vi "MainKinetics.vi"() -> ()   [LabVIEW 2017]
uses:
  <vilib>/Utility/miscctls.llb/LVRowAndColumnTypeDef.ctl
  <vilib>/Utility/sysdir.llb/System Directory Type.ctl
  <vilib>/Utility/config.llb/Read Key (String).vi
  <vilib>/Utility/config.llb/Write Key (String).vi
  <vilib>/Utility/cursorutil.llb/Set Cursor (Icon Pict).vi
  PCAN_Driver/ControlCAN.lvlib
  <vilib>/Utility/config.llb/NI_LVConfig.lvlib
panel:
  out "Motor Speed RPM Serial":dbl
  out "DAQmx Device Name":tag
  out "PN":string
  out "FileName":string
  out "Numeric":dbl
  out "BurnInSpeed":u16
  out "VenableSpeed":u16
  out "CurrentTest":T1(ring)
  out "TesterVersion":string
  out "ClosePanel":bool=TRUE
  out "UUT SN Report":string
  out "Automation":bool
  out "Test Failed":bool
  out "AuxiOFFResult":bool
  out "AuxiONResult":bool
  out "SensCalResult":bool
  out "VisualInspectionResult":bool
  out "BurnResult":bool
  out "BurnSpeed":bool
  out "BurnTemp":bool
  out "BurnDC":bool
  out "TempControlResult":bool
  out "MotorTempResult":bool
  out "VenableDirectionResult":bool
  out "VenableResult":bool
  out "ComTestResult":bool=TRUE
  out "UUT SoftwareVer":string
  out "Next SN":i32
  in  "SetSN":bool
  out "Current SN":i32
  out "AO[1]Meas":dbl
  out "FullSpeed2 Speed":dbl
  out "FullSpeed2 Current":dbl
  out "FullSpeed1 Current":dbl
  out "FullSpeed1 Speed":dbl
  out "MaxBurnInTempVal":dbl
  out "UUT":u8
  out "CAN Status":bool
  out "Array":u64[][](array[numeric]) format="%016x"
  out "Motor Phase Current RMS":dbl
  out "Ambient Temperature":dbl
  out "Speed error":bool
  out "Commutation err":bool
  out "Under voltage/Over voltage":bool
  out "Derated drive temp":bool
  out "Motor Over temperature":bool
  out "Motor Sensor temp Fauilre":bool
  out "Drive Over temperature":bool
  out "Drive Sensor temp Failure":bool
  out "Ambient Over temp":bool
  out "Ambient Sensor temp":bool
  out "DC Voltage":dbl
  out "DC Current":dbl
  out "Power transistor Heat sink Temp.":dbl
  out "Motor Stator Temp.":dbl
  out "Motor Speed RPM":dbl
  out "ECS State":u16
  out "UUT":string="EBAY"
  in  "Logger Path":path
  in  "Report":bool
  in  "Start":bool
  in  "ATR":string[][](table)=[["Test Communication", "-", "-", "-", "-", ""], ["Set S/N", "-", "-", "-", "-", ""], ["Set Board Number", "-", "-", "-", "-", ""], [" ", "", "", "", "", ""], ["Test Communication", "-", "-", "-", "-", ""], ["Get S/N", "-", "-", "-", "", ""], ["Get Board Number", "-", "-", "-", "", ""], ["Get FW", "-", "-", "-", "", ""], ["Enable Motor", "", "", "", "", ""], ["Small position command", "", "", "", "", ""], ["Measure delta", "", "", "", "", ""], ["Velocity command", "", "", "", "", ""]]
  in  "Settings":bool
  in  "Refresh Button":bool
  out "Status":bool
  in  "VISA Kinetics":refnum<visa-resource-name>="COM6"
  in  "Serial Com":bool
  in  "Help Button":bool
  out "Pannel User Message":string
  in  "Stop Button":bool
  # "Kinetics"
  # "REDLER TECHNOLOGIES LTD"
  # "ver 1.2p"
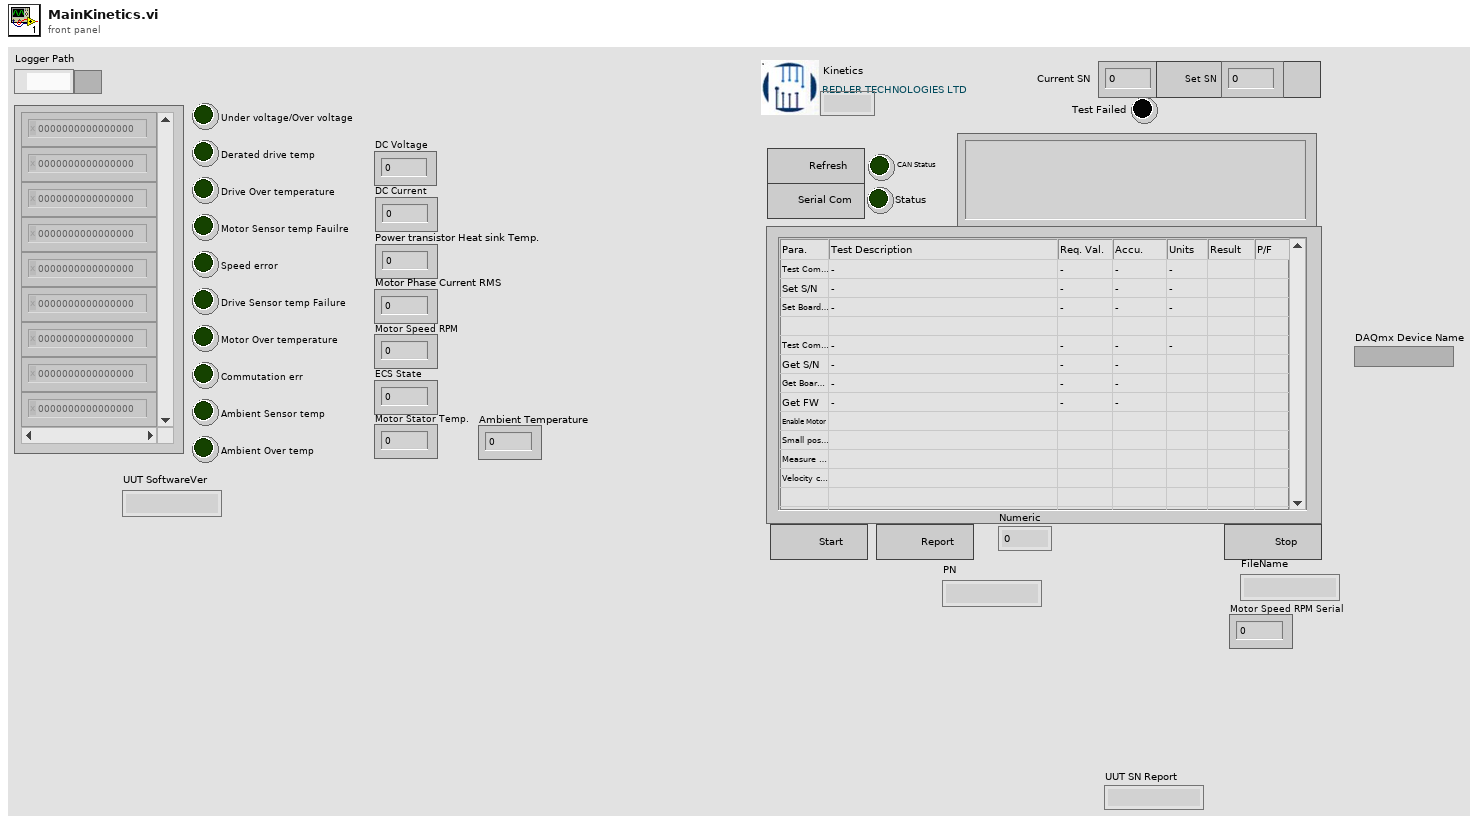
[diagram p1: front panel]
types:
  T1 = enum16{"Auxiliary", "Temp Sens Cal", "Com Test", "Enable Test", "Speed Command", "Stop Time", "Temp Control", "Burn in", "Visual Inspec", "Empty"}
  T2 = cluster{"VISA":refnum<visa-resource-name>, "Array Test":enum16{"Auxiliary", "Temp Sens Cal", "Com Test", "Enable Test", "Speed Command", "Stop Time", "Temp Control", "Burn in", "Visual Inspec", "Empty"}[]}
  T3 = cluster{"ID":u32, "MSGTYPE":u8, "LEN":u8, "aDATA":u8[]}[]
  T4 = enum16{"Erase ATR Table", "Stop", "MainProgram", "Initialize"}
  T5 = typedef "NI_LVConfig.lvlib/Config Data RefNum.ctl" = refnum<k1>
  T6 = enum16{"K15", "K16", "K17", "Venable", "Firmeware", "Fan", "Power", "120C", "110C", "100C", "90C", "80C", "70C", "60C", "50C", "40C", "30C", "25C", "20C", "10C", "0C"}
  T7 = enum16{"Stop", "Result", "FullSpeed2", "MD[1]=1", "FullSpeed1", "MD[1]=0"}
  T8 = enum8{"Term1", "Term2", "Current", "Fan", "TempCPU"}
  T9 = enum16{"Stop", "AO[1]=Meas.", "TA[5]", "AO[1]=0", "Start"}
  T10 = enum16{"Stop", "BurnIn", "Ambient Temp", "MotorSpeed", "DC Current Measure", "Start"}
  T11 = enum16{"Auxiliary", "Temp Sens Cal", "Com Test", "Enable Test", "Speed Command", "Stop Time", "Temp Control", "Burn in", "Visual Inspec", "Empty"}[]
  T12 = enum16{"K15", "K16", "K17", "Venable", "Firmeware", "Fan", "Power", "120C", "110C", "100C", "90C", "80C", "70C", "60C", "50C", "40C", "30C", "25C", "20C", "10C", "0C"}[]
  T13 = enum32{"6000", "11500", "15100", "11500-2", "6000-2"}[]
  T14 = enum8{"Enabled", "Disabled", "Disabled and Grayed Out"}
  T15 = typedef "LVRowAndColumnTypeDef.ctl" = cluster{"Row":i32, "Column":i32}
  T16 = enum32{"Invalid", "Standard", "Closed", "Hidden", "Minimized", "Maximized"}
  T17 = cluster{"ID":u32, "MSGTYPE":u8, "LEN":u8, "aDATA":u8[]}
  T18 = enum16{"open", "replace", "create", "open or create", "replace or create", "replace or create with confirmation"}
  T19 = typedef "ControlCAN.lvlib/DevType.ctl" = u32
  T20 = typedef "ControlCAN.lvlib/CAN Channel.ctl" = u32
  T21 = typedef "ControlCAN.lvlib/VCI_INIT_CONFIG.ctl" = cluster{"AccCode":u32, "AccMask":u32, "InitFlag":T22, "Fliter":T23, "Timing0":u8, "Timing1":u8, "Mode":T24}
  T22 = typedef "ControlCAN.lvlib/InitFlag.ctl" = u32
  T23 = typedef "ControlCAN.lvlib/Fliter.ctl" = u8
  T24 = typedef "ControlCAN.lvlib/Mode.ctl" = u8
  T25 = cluster{"DevType":T19, "DevIndex":u32, "CanIndex":T20, "VCI_INIT_CONFIG":T21}
  T26 = typedef "ControlCAN.lvlib/VCI_CAN_OBJ.ctl" = cluster{"ID":u32, "TimeStamp":u32, "TimeFlag":u8, "SendType":u8, "RemoteFlag":u8, "ExternFlag":u8, "DataLen":u8, "Data":u8[], "Reserved":u8[]}
  T27 = cluster{"Type":enum16{"接收", "发送"}, "Channel":T20, "Time":timestamp, "VCI_CAN_OBJ":T26}[]
  T28 = cluster{"Type":enum16{"接收", "发送"}, "Channel":T20, "Time":timestamp, "VCI_CAN_OBJ":T26}
  T29 = typedef "LVPoint32TypeDef.ctl" = cluster{"Horizontal":i32, "Vertical":i32}
  T30 = enum8{"Term1", "Term2", "Current", "Fan", "TempCPU"}[]
  T31 = typedef "System Directory Type.ctl" = i32
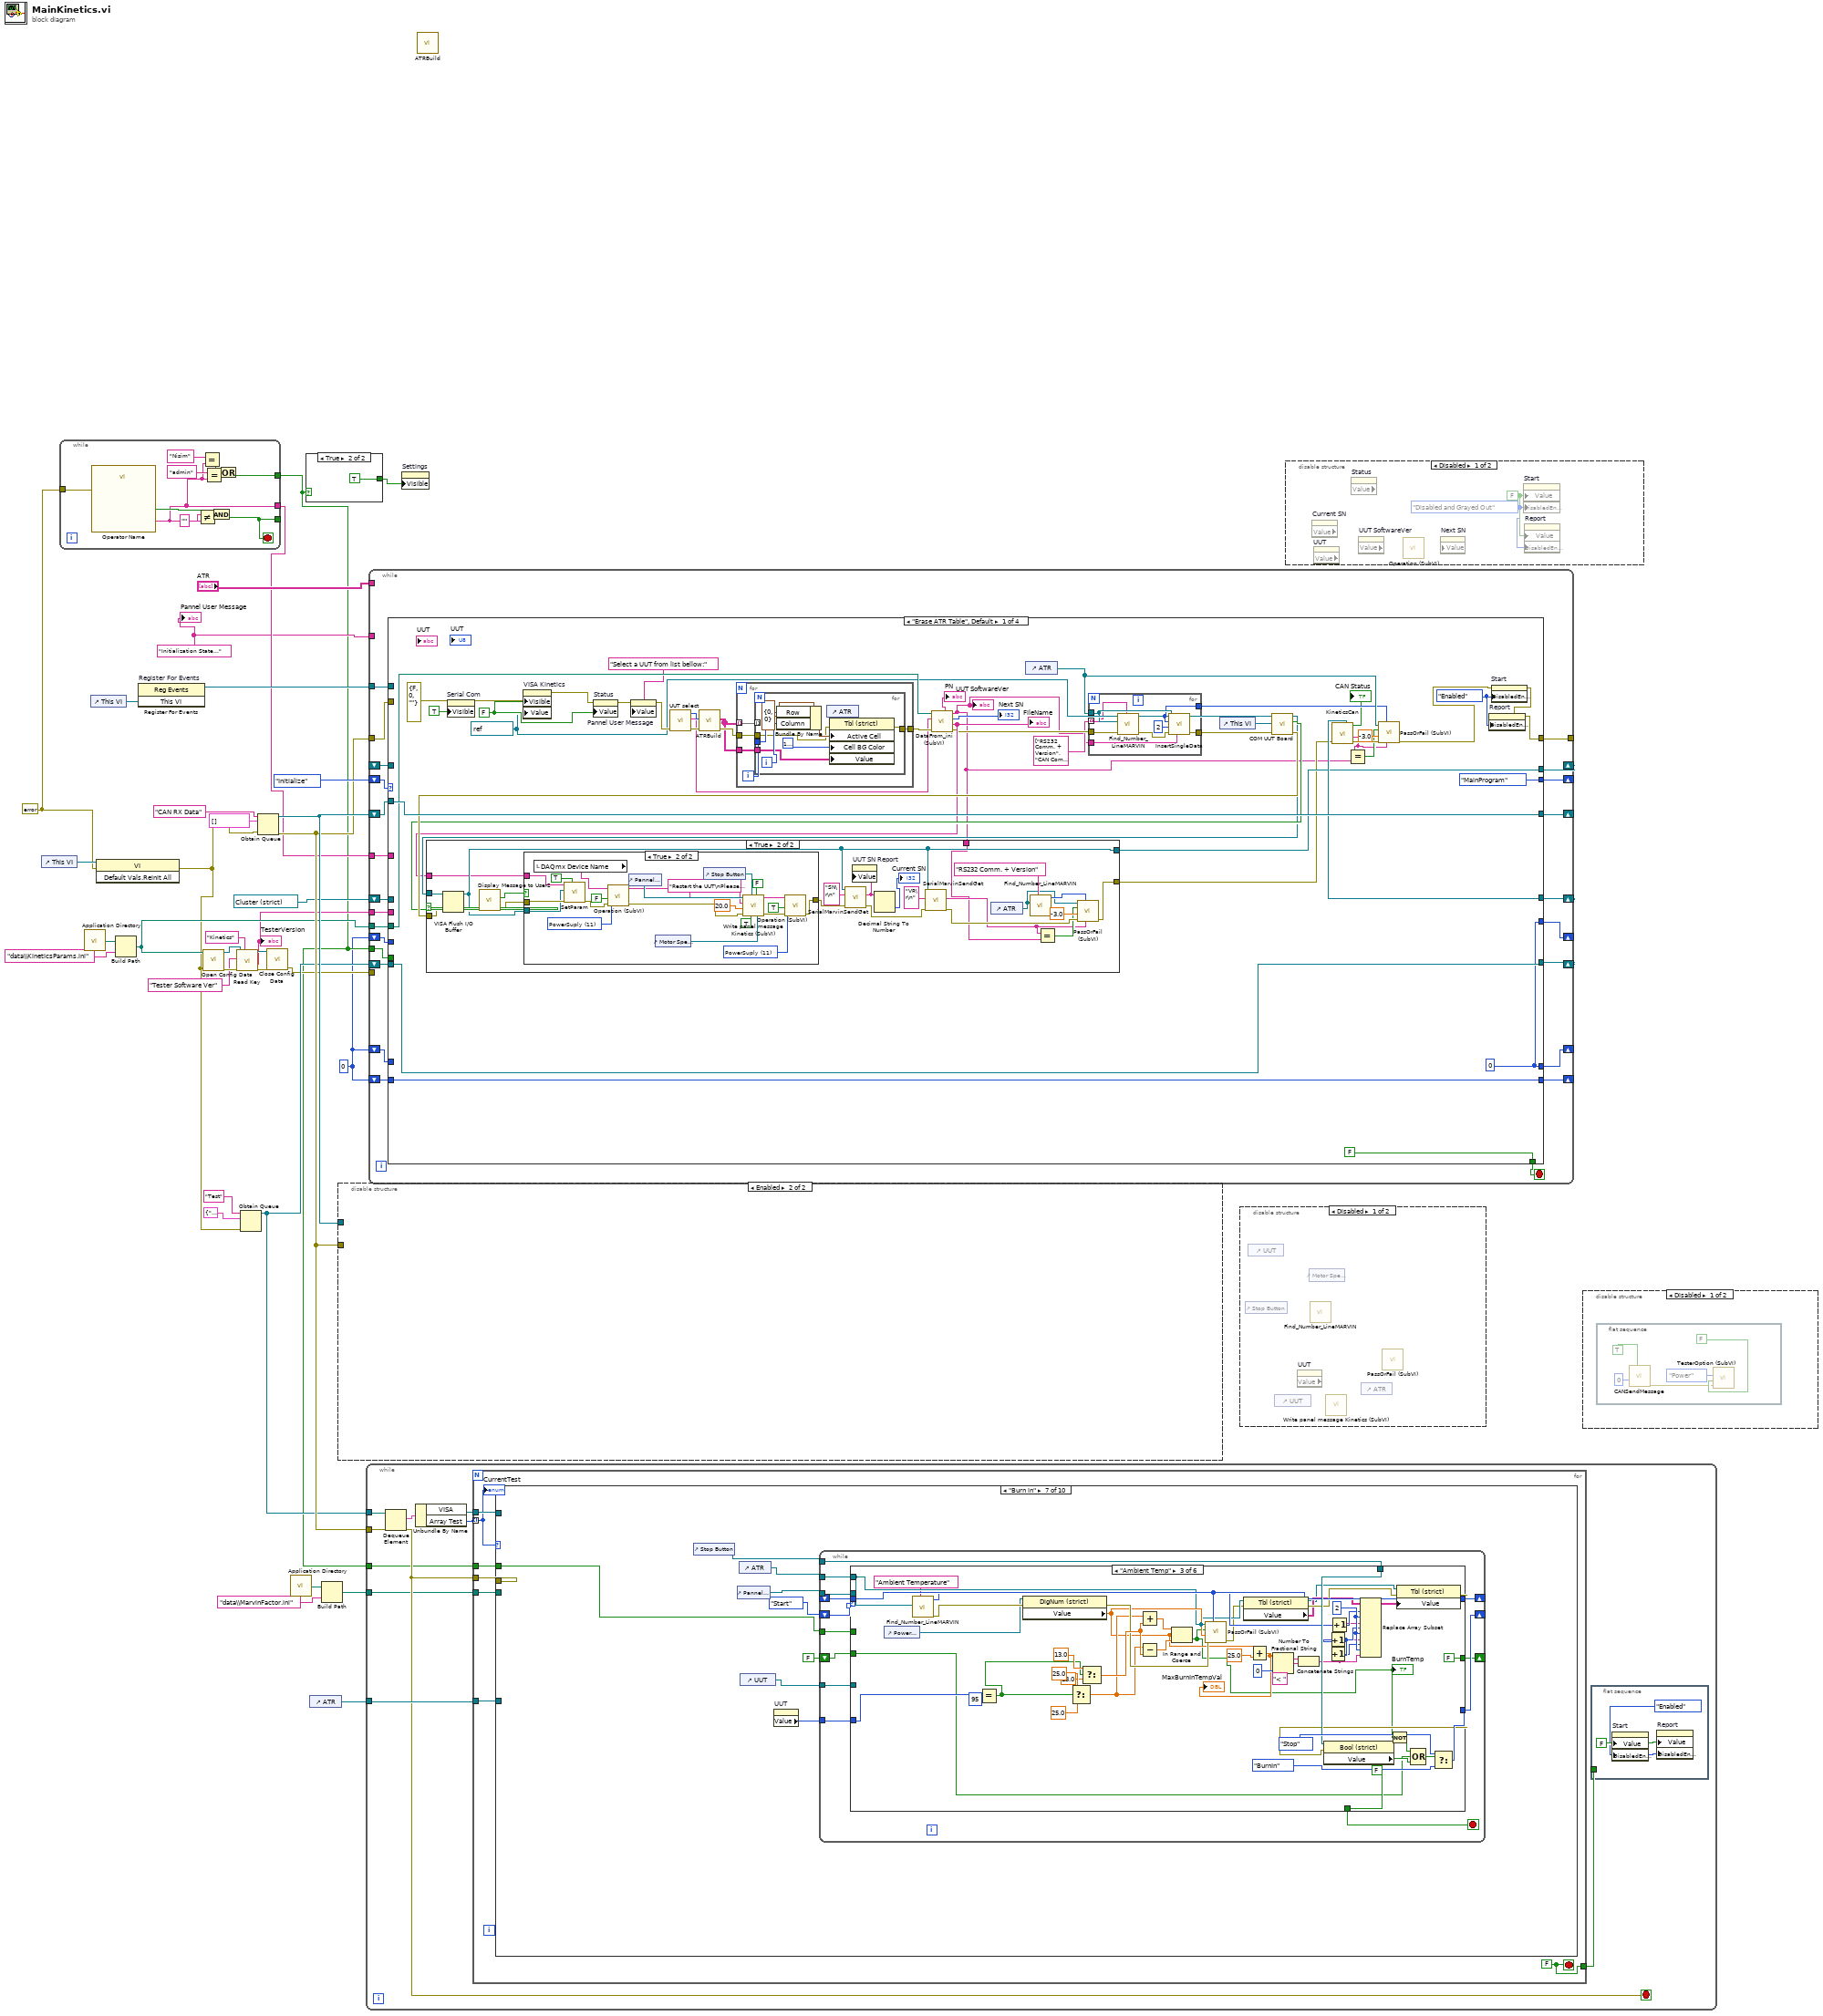
[diagram p0: block diagram]
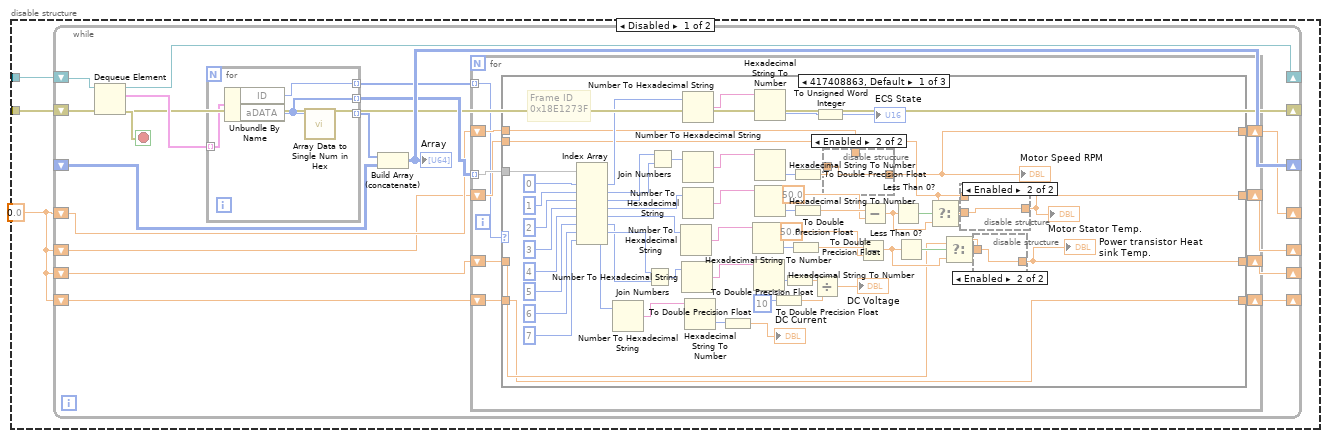
[diagram p2: hidden frame]
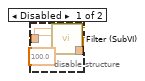
[diagram p3: hidden frame]
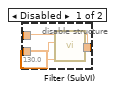
[diagram p4: hidden frame]
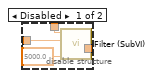
[diagram p5: hidden frame]
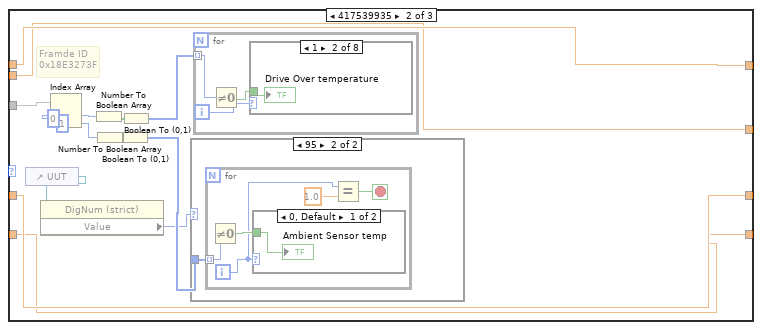
[diagram p6: hidden frame]
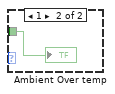
[diagram p8: hidden frame]
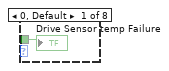
[diagram p9: hidden frame]
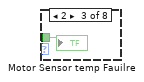
[diagram p10: hidden frame]
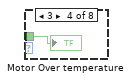
[diagram p11: hidden frame]
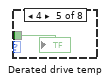
[diagram p12: hidden frame]
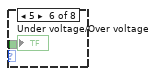
[diagram p13: hidden frame]
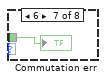
[diagram p14: hidden frame]
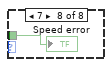
[diagram p15: hidden frame]
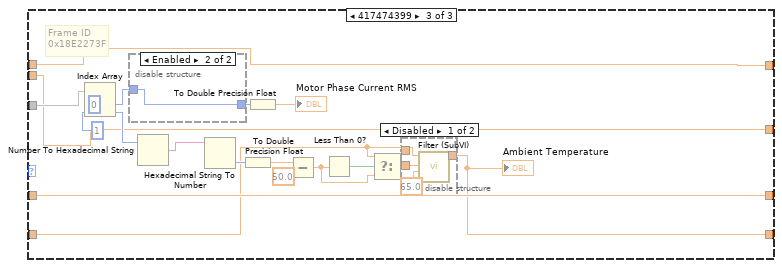
[diagram p16: hidden frame]
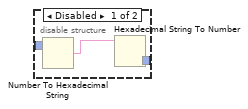
[diagram p18: hidden frame]
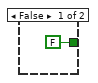
[diagram p19: hidden frame]
diagram:
  w19 = "Initialization State..."
  w1 = 0
  w4 = errorcluster {"status"=FALSE, "code"=0, "source"=""} ("error in (no error)")
  n1 = control-ref of="This VI"() -> (w5:refnum<vi>)
  n2 = while {
    tunnel: [w43] -> _
    tunnel: [w39] -> w21
    tunnel: [w40] -> w2
    tunnel: w4 -> [w36]
    stop <- w43 stop-if-true
    n3 = call "Operator Name"("error in (no error)"=w36) -> ("Operator Name"=w39:string, "OK"=w44:bool)  [unwired: 16 in, 1 out]
    n4 = Not Equal?(x=w39, y="") -> (x != y?=w45:bool)
    n5 = Equal?(x="Nisim", y=w39) -> (x = y?=w37:bool)
    n6 = Equal?(x="admin", y=w39) -> (x = y?=w41:bool)
    n7 = And(x=w44, y=w45) -> (x .and. y?=w43:bool)
    n8 = Or(x=w37, y=w41) -> (x .or. y?=w40:bool)
  }
  n9 = call <vilib>:"Application Directory.vi"() -> ("Application Directory"=w25:path)
  n10 = control-ref of="This VI"() -> (w23:refnum<vi>)
  n11 = invoke class="VI" method="Default Vals.Reinit All"(reference=w5, error in=w4) -> (error out=w3:errorcluster)  [unwired: 1 in, 2 out]
  n12 = Build Path(base path=w25, name or relative path="data\\KineticsParams.ini") -> (appended path=w8:path)
  n13 = register-events "Register For Events"(w23) -> (reference out=w22:refnum<event-registration>)  [unwired: 2 in, 1 out]
  n14 = call <vilib>:"Open Config Data.vi"("error in (no error)"=w3, "configuration file path"=w8) -> ("error out"=w14:errorcluster, "refnum"=w13:T5)  [unwired: 1 in, 7 out]
  n15 = call-poly <vilib>:"Read Key.vi"("section"="Kinetics", "error in (no error)"=w14, "key"="Tester Software Ver", "refnum"=w13) -> ("error out"=w11:errorcluster, "value"=w6:string, "refnum out"=w10:T5)  [unwired: 2 in, 3 out]
  "TesterVersion" <- w6
  n16 = Obtain Queue(name (unnamed)="Test", element data type=T2 {"VISA"="COM1", "Array Test"=[]}, error in (no error)=w3) -> (queue out=w29:refnum<queue>)  [unwired: 2 in, 2 out]
  n17 = Obtain Queue(name (unnamed)="CAN RX Data", element data type=T3 [], error in (no error)=w3) -> (queue out=w32:refnum<queue>, error out=w30:errorcluster)  [unwired: 2 in, 1 out]
  n18 = call <vilib>:"Close Config Data.vi"("error in (no error)"=w11, "refnum"=w10) -> ("error out"=w9:errorcluster)  [unwired: 8 in, 1 out]
  n19 = call <vilib>:"Application Directory.vi"() -> ("Application Directory"=w16:path)
  n20 = case shown="True" w2 {
    tunnel: [FALSE TRUE] -> w20
    frame False {
    }
    frame True {
    }
  }
  n21 = control-ref of="ATR"() -> (w18:refnum<vi>)
  n22 = Build Path(base path=w16, name or relative path="data\\MarvinFactor.ini") -> (appended path=w15:path)
  n23 = disable-structure shown="Enabled" {
    disable-tunnel: w32 -> [w51 _]
    disable-tunnel: w30 -> [w50 _]
    frame Disabled {
      w49 = 0.0
      n24 = while {
        shift-right: [w67] -> _
        shift-left: w51 -> [w69]
        shift-right: [w65] -> _
        shift-left: _ -> [w66]
        shift-right: [w61] -> _
        shift-left: w50 -> [w61]
        shift-right: [w59] -> _
        shift-left: w49 -> [w60]
        shift-right: [w58] -> _
        shift-left: w49 -> [w57]
        shift-right: [w56] -> _
        shift-left: w49 -> [w55]
        shift-right: [w54] -> _
        shift-left: w49 -> [w53]
        stop <- w68 stop-if-true
        n25 = Dequeue Element(queue=w69, error in (no error)=w61) -> (queue out=w67:refnum<queue>, element=w62:T3, error out=w68:errorcluster)  [unwired: 1 in, 1 out]
        n26 = for {
          tunnel: [w215] -> w64 mode=indexing
          tunnel: w62 -> [w214] mode=indexing
          tunnel: [w213] -> w63 mode=indexing
          tunnel: [w212] -> w52 mode=indexing
          n27 = Unbundle By Name(w214) -> ("ID"=w212:u32, "aDATA"=w213:u8[])
          n28 = call "Array Data to Single Num in Hex.vi"("aDATA"=w213) -> ("Numeric"=w215:u64)  [unwired: 10 in]
        }
        n29 = Build Array (concatenate)(w64, w66) -> (w65:u64[][])
        "Array" <- w65
        n30 = for {
          tunnel: w63 -> [w79] mode=indexing
          shift-right: [w77] -> w59
          shift-left: w60 -> [w78]
          shift-right: [w76] -> w58
          shift-left: w57 -> [w75]
          shift-right: [w74] -> w56
          shift-left: w55 -> [w73]
          shift-right: [w72] -> w54
          shift-left: w53 -> [w71]
          tunnel: w52 -> [w70] mode=indexing
          n31 = case shown="417408863, Default" w70 {
            tunnel: w79 -> [w116 w164 w202]
            tunnel: w78 -> [w90 w153 w191]
            tunnel: [w89 w153 w191] -> w77
            tunnel: [w86 w152 w190] -> w76
            tunnel: w75 -> [w85 w152 w190]
            tunnel: [w82 w151 w189] -> w74
            tunnel: w73 -> [w81 w151 w189]
            tunnel: [w80 w150 w185] -> w72
            tunnel: w71 -> [w80 w150 w184]
            frame 417408863, Default {
              # "Frame ID\n0x18E1273F"
              n32 = Index Array(array=w116, index #1=0 ("index"), index #2=1 ("index"), index #3=2 ("index"), index #4=3 ("index"), index #5=4 ("index"), index #6=5 ("index"), index #7=6 ("index"), index #8=7 ("index")) -> (element #1=w100:u8, element #2=w102:u8, element #3=w103:u8, element #4=w107:u8, element #5=w110:u8, element #6=w114:u8, element #7=w115:u8, element #8=w113:u8)
              n33 = Number To Hexadecimal String(2:w113) -> (0:w127:string)  [unwired: 1 in]
              n34 = Join Numbers(hi=w115, lo=w114) -> ((hi.lo)=w134:u16)
              n35 = Join Numbers(hi=w103, lo=w102) -> ((hi.lo)=w104:u16)
              n36 = Number To Hexadecimal String(2:w110) -> (0:w111:string)  [unwired: 1 in]
              n37 = Number To Hexadecimal String(2:w134) -> (0:w133:string)  [unwired: 1 in]
              n38 = Number To Hexadecimal String(2:w100) -> (0:w101:string)  [unwired: 1 in]
              n39 = Number To Hexadecimal String(2:w104) -> (0:w105:string)  [unwired: 1 in]
              n40 = Number To Hexadecimal String(2:w107) -> (0:w108:string)  [unwired: 1 in]
              n41 = Hexadecimal String To Number(string=w127) -> (number=w126:u32)  [unwired: 2 in, 1 out]
              n42 = To Double Precision Float(number=w126) -> (double precision float=→"DC Current":dbl)
              n43 = Hexadecimal String To Number(string=w111) -> (number=w112:u32)  [unwired: 2 in, 1 out]
              n44 = Hexadecimal String To Number(string=w133) -> (number=w132:u32)  [unwired: 2 in, 1 out]
              n45 = Hexadecimal String To Number(string=w101) -> (number=w98:u32)  [unwired: 2 in, 1 out]
              n46 = Hexadecimal String To Number(string=w105) -> (number=w106:u32)  [unwired: 2 in, 1 out]
              n47 = Hexadecimal String To Number(string=w108) -> (number=w109:u32)  [unwired: 2 in, 1 out]
              n48 = To Double Precision Float(number=u32 10 ("y")) -> (double precision float=w130:dbl)
              n49 = To Double Precision Float(number=w132) -> (double precision float=w129:dbl)
              n50 = To Double Precision Float(number=w112) -> (double precision float=w95:dbl)
              n51 = To Double Precision Float(number=w106) -> (double precision float=w91:dbl)
              n52 = To Double Precision Float(number=w109) -> (double precision float=w97:dbl)
              n53 = Divide(x=w129, y=w130) -> (x/y=→"DC Voltage":dbl)
              n54 = To Unsigned Word Integer(number=w98) -> (unsigned 16bit integer=→"ECS State":u16)
              n55 = disable-structure shown="Enabled" {
                disable-tunnel: w91 -> [w148 w149]
                disable-tunnel: w90 -> [w147 _]
                disable-tunnel: [w145 w149] -> w89
                frame Disabled {
                  n56 = call "Filter (SubVI).vi"("Delta"=5000.0, "NewVal"=w148, "OldVal"=w147) -> ("Val"=w145:dbl)  [unwired: 8 in]
                }
                frame Enabled {
                }
              }
              "Motor Speed RPM" <- w89
              n57 = Subtract(x=w95, y=50.0 ("x")) -> (x-y=w84:dbl)
              n58 = Subtract(x=w97, y=50.0 ("x")) -> (x-y=w87:dbl)
              n59 = Less Than 0?(x=w87) -> (x < 0?=w93:bool)
              n60 = Less Than 0?(x=w84) -> (x < 0?=w92:bool)
              n61 = Select(t=w85, s=w93, f=w87) -> (s? t:f=w88:dbl)
              n62 = Select(t=w81, s=w92, f=w84) -> (s? t:f=w83:dbl)
              n63 = disable-structure shown="Enabled" {
                disable-tunnel: w88 -> [w143 w144]
                disable-tunnel: [w142 w144] -> w86
                disable-tunnel: w85 -> [w141 _]
                frame Disabled {
                  n64 = call "Filter (SubVI).vi"("Delta"=130.0, "NewVal"=w143, "OldVal"=w141) -> ("Val"=w142:dbl)  [unwired: 8 in]
                }
                frame Enabled {
                }
              }
              "Motor Stator Temp." <- w86
              n65 = disable-structure shown="Enabled" {
                disable-tunnel: w83 -> [w138 w139]
                disable-tunnel: [w136 w139] -> w82
                disable-tunnel: w81 -> [w135 _]
                frame Disabled {
                  n66 = call "Filter (SubVI).vi"("Delta"=100.0, "NewVal"=w138, "OldVal"=w135) -> ("Val"=w136:dbl)  [unwired: 8 in]
                }
                frame Enabled {
                }
              }
              "Power transistor Heat sink Temp." <- w82
            }
            frame 417539935 {
              # "Framde ID\n0x18E3273F"
              n67 = control-ref of="UUT"() -> (w154:refnum<vi>)
              n68 = property on="Property Node" class="DigNum (strict)"(reference=w154) -> ("Value"=w155:u8)  [unwired: 1 in, 2 out]
              n69 = Index Array(array=w164, index #1=0 ("index"), index #2=1 ("index")) -> (element #1=w162:u8, element #2=w157:u8)
              n70 = Number To Boolean Array(number=w162) -> (Boolean array=w161:bool[])
              n71 = Number To Boolean Array(number=w157) -> (Boolean array=w159:bool[])
              n72 = Boolean To (0,1)(Boolean=w159) -> (0, 1=w156:i16[])
              n73 = Boolean To (0,1)(Boolean=w161) -> (0, 1=w160:i16[])
              n74 = case shown="95" w155 {
                tunnel: w156 -> [_ w165]
                frame 0, Default {
                }
                frame 95 {
                  n75 = for {
                    tunnel: w165 -> [w170] mode=indexing
                    i -> [w166]
                    stop <- w168 stop-if-true
                    n76 = Not Equal To 0?(x=w170) -> (x != 0?=w169:bool)
                    n77 = case shown="0, Default" w166 {
                      tunnel: w169 -> [w171 w172]
                      frame 0, Default {
                        "Ambient Sensor temp" <- w171
                      }
                      frame 1 {
                        "Ambient Over temp" <- w172
                      }
                    }
                    n78 = Equal?(x=w166, y=1.0) -> (x = y?=w168:bool)
                  }
                }
              }
              n79 = for {
                tunnel: w160 -> [w174] mode=indexing
                i -> [w175]
                n80 = Not Equal To 0?(x=w174) -> (x != 0?=w173:bool)
                n81 = case shown="1" w175 {
                  tunnel: w173 -> [w176 w177 w178 w179 w180 w181 w182 w183]
                  frame 0, Default {
                    "Drive Sensor temp Failure" <- w176
                  }
                  frame 1 {
                    "Drive Over temperature" <- w177
                  }
                  frame 2 {
                    "Motor Sensor temp Fauilre" <- w178
                  }
                  frame 3 {
                    "Motor Over temperature" <- w179
                  }
                  frame 4 {
                    "Derated drive temp" <- w180
                  }
                  frame 5 {
                    "Under voltage/Over voltage" <- w181
                  }
                  frame 6 {
                    "Commutation err" <- w182
                  }
                  frame 7 {
                    "Speed error" <- w183
                  }
                }
              }
            }
            frame 417474399 {
              # "Frame ID\n0x18E2273F"
              n82 = Index Array(array=w202, index #1=0 ("index"), index #2=1 ("index")) -> (element #1=w199:u8, element #2=w196:u8)
              n83 = disable-structure shown="Enabled" {
                disable-tunnel: [w210 w211] -> w200
                disable-tunnel: w199 -> [w209 w211]
                frame Disabled {
                  n84 = Number To Hexadecimal String(2:w209) -> (0:w208:string)  [unwired: 1 in]
                  n85 = Hexadecimal String To Number(string=w208) -> (number=w210:u32)  [unwired: 2 in, 1 out]
                }
                frame Enabled {
                }
              }
              n86 = Number To Hexadecimal String(2:w196) -> (0:w194:string)  [unwired: 1 in]
              n87 = Hexadecimal String To Number(string=w194) -> (number=w195:u32)  [unwired: 2 in, 1 out]
              n88 = To Double Precision Float(number=w195) -> (double precision float=w193:dbl)
              n89 = To Double Precision Float(number=w200) -> (double precision float=→"Motor Phase Current RMS":dbl)
              n90 = Subtract(x=w193, y=50.0) -> (x-y=w187:dbl)
              n91 = Less Than 0?(x=w187) -> (x < 0?=w188:bool)
              n92 = Select(t=w184, s=w188, f=w187) -> (s? t:f=w186:dbl)
              n93 = disable-structure shown="Disabled" {
                disable-tunnel: w186 -> [w206 w207]
                disable-tunnel: [w204 w207] -> w185
                disable-tunnel: w184 -> [w203 _]
                frame Disabled {
                  n94 = call "Filter (SubVI).vi"("Delta"=65.0, "NewVal"=w206, "OldVal"=w203) -> ("Val"=w204:dbl)  [unwired: 8 in]
                }
                frame Enabled {
                }
              }
              "Ambient Temperature" <- w185
            }
          }
        }
      }
    }
    frame Enabled {
    }
  }
  n95 = while {
    tunnel: w18 -> [w225]
    tunnel: w30 -> [w223]
    tunnel: w29 -> [w224]
    tunnel: w15 -> [w217]
    tunnel: w2 -> [w216]
    stop <- w219 stop-if-true
    n96 = Dequeue Element(queue=w224, error in (no error)=w223) -> (element=w222:T2, error out=w219:errorcluster)  [unwired: 1 in, 2 out]
    n97 = Unbundle By Name(w222) -> ("VISA"=w221:refnum<visa-resource-name>, "Array Test"=w220:T11)
    n98 = for {
      tunnel: w220 -> [w231] mode=indexing
      tunnel: w221 -> [w234]
      tunnel: w225 -> [w233]
      tunnel: w219 -> [w232]
      tunnel: [w230] -> w218
      tunnel: w217 -> [w229]
      tunnel: w216 -> [w228]
      stop <- w230 stop-if-true
      w230 = FALSE
      n99 = case shown="\"Burn in\"" w231 {
        tunnel: w234 -> [_ w257 _ _ w641 _ _ _ w1170 w1353]
        tunnel: w233 -> [_ w264 _ w625 w637 w792 _ w1131 w1177 w1364]
        tunnel: w232 -> [_ w261 _ w630 w647 w776 _ w1129 w1175 w1363]
        tunnel: w229 -> [_ _ _ _ _ w778 _ _ _ _]
        tunnel: w228 -> [_ _ _ _ _ _ w920 _ _ _]
        frame "Empty", Default {
        }
        frame "Com Test" {
          w242 = "Communication Test" ("Test Paragraph")
          n100 = control-ref of="Pannel User Message"() -> (w262:refnum<vi>)
          n101 = property class="Str"(reference=w262, error in=w261, "Value"="Communication Test in process") -> (error out=w260:errorcluster)  [unwired: 1 out]
          n102 = call "Table_ScrollaBarMarvin.vi"("error in"=w260, "Line to focus"=w242, "reference in"=w264) -> ("error out"=w263:errorcluster)  [unwired: 2 out]
          n103 = property class="Tbl (strict)"(reference=w264, error in=w263) -> (reference out=w243:refnum<vi>, error out=w270:errorcluster, "Value"=w271:string[][])
          n104 = Index Array(array=w271, index (col)=1 ("disabled index (col)")) -> (element=w272:string[])  [unwired: 1 in]
          n105 = call "Find_Number_Line.vi"("error in"=w270, "Test Paragraph"=w242, "Row Headers[]"=w272) -> ("error out"=w268:errorcluster, "Line number"=w267:i32)  [unwired: 1 out]
          n106 = call <vilib>:"Clear Errors.vi"("error in (no error)"=w268) -> ("error out"=w253:errorcluster)  [unwired: 5 in, 1 out]
          n107 = call "TesterOption (SubVI).vi"("2 Options"=FALSE, "error in (no error)"=w253, "On/Off"=FALSE, "Tester Option"=T6."Venable") -> ("error out"=w252:errorcluster)  [unwired: 6 in, 1 out]
          n108 = Increment(x=w267) -> (x+1=w235:i32)
          n109 = call "Time Delay3"("error in (no error)"=w252) -> ("error out"=w265:errorcluster)  [unwired: 10 in]
          n110 = call "Reset old test Values (SubVI).vi"("error in"=w265, "Atr in"=w243, "Test Paragraph"=w242) -> ("error out"=w237:errorcluster)  [unwired: 8 in]
          n111 = property on="CAN Status" class="Bool (strict)"(error in=w237) -> (error out=w236:errorcluster, "Value"=w238:bool)  [unwired: 1 in, 1 out]
          n112 = Increment(x=w235) -> (x+1=w266:i32)
          n113 = call "PassOrFail (SubVI).vi"("index (row)"=w266, "error in (no error)"=w236, "Data in"=-3.0, "Pass?Fail"=w238, "Table in"=w264) -> ("error out"=w256:errorcluster)  [unwired: 6 in]
          n114 = property on="Status" class="Bool (strict)"(error in=w256) -> ("Value"=w258:bool)  [unwired: 1 in, 2 out]
          n115 = case shown="True" w258 {
            tunnel: w257 -> [_ w279]
            tunnel: [FALSE w276] -> w240
            tunnel: ["" ("read buffer") w275] -> w255
            frame False {
              n116 = call "Display Message to User"() -> ()  [unwired: 10 in, 2 out]
            }
            frame True {
              n117 = property on="UUT SoftwareVer" class="Str"() -> ("Value"=w277:string)  [unwired: 2 in, 2 out]
              n118 = call "SerialMarvinSendGet.vi"("write buffer"="VR\r\n", "VISA resource name"=w279) -> ("read buffer"=w275:string)  [unwired: 8 in, 1 out]
              n119 = Equal?(x=w275, y=w277) -> (x = y?=w276:bool)
            }
          }
          n120 = call "PassOrFail (SubVI).vi"("String Res"=w255, "index (row)"=w235, "Data in"=-3.0, "Pass?Fail"=w240, "Table in"=w264) -> ("error out"=w248:errorcluster)  [unwired: 6 in]
          n121 = Build Array(w238, w240) -> (w241:bool[])
          n122 = And Array Elements(Boolean array=w241) -> (logical AND=→"ComTestResult":bool)
          n123 = call "TesterOption (SubVI).vi"("2 Options"=FALSE, "error in (no error)"=w248, "On/Off"=FALSE, "Tester Option"=T6."Venable") -> ()  [unwired: 6 in, 2 out]
        }
        frame "Enable Test" {
          n124 = control-ref of="Stop Button"() -> (w282:refnum<vi>)
          n125 = control-ref of="Pannel User Message"() -> (w284:refnum<vi>)
          n126 = control-ref of="ATR"() -> (w283:refnum<vi>)
          n127 = control-ref of="Motor Speed RPM"() -> (w285:refnum<vi>)
          n128 = control-ref of="UUT"() -> (w286:refnum<vi>)
          n129 = while {
            shift-right: [w289] -> _
            shift-left: enum16{"Stop", "Direction", "Venable", "Start"}."Start" -> [w295]
            tunnel: w282 -> [w294]
            tunnel: w283 -> [w293]
            tunnel: w284 -> [w292]
            tunnel: w285 -> [w291]
            tunnel: w286 -> [w287]
            tunnel: "Enable test in process..." ("Strin") -> [w288]
            stop <- w290 stop-if-true
            n130 = case shown="\"Stop\", Default" w295 {
              tunnel: w294 -> [_ w320 w569 w607]
              tunnel: w293 -> [_ w316 w567 w614]
              tunnel: w292 -> [_ w319 w570 w613]
              tunnel: w291 -> [_ w318 w571 w606]
              tunnel: w287 -> [w296 w312 w572 _]
              tunnel: [w298 FALSE FALSE FALSE] -> w290
              tunnel: [w297 w315 w568 w611] -> w289
              tunnel: w288 -> [_ w317 w566 w605]
              frame "Stop", Default {
                n131 = flat-sequence {
                  tunnel: w296 -> [_]
                  tunnel: [TRUE] -> w298
                  tunnel: [enum16{"Stop", "Direction", "Venable", "Start"}."Stop"] -> w297
                  frame #0 {
                    (unwired) u16 0 ("Motor Speed RPM")
                    (unwired) TRUE ("Remote")
                    n132 = property on="VISA Kinetics" class="VISAName"() -> (error out=w302:errorcluster, "Value"=w303:refnum<visa-resource-name>)  [unwired: 2 in, 1 out]
                    n133 = call "SerialMarvinSendGet.vi"("error in (no error)"=w302, "Clear Log"=FALSE, "write buffer"="EP=1\r\nMD[1]=1\r\n", "VISA resource name"=w303) -> ("error out"=w299:errorcluster)  [unwired: 6 in, 1 out]
                    n134 = call "CANSendMessage.vi"("error in (no error)"=w299) -> ("error out"=w308:errorcluster)  [unwired: 10 in]
                    n135 = call "TesterOption (SubVI).vi"("2 Options"=FALSE, "error in (no error)"=w308, "On/Off"=FALSE, "Tester Option"=T6."Venable") -> ("error out"=w304:errorcluster)  [unwired: 6 in, 1 out]
                    n136 = call "Time Delay9"("error in (no error)"=w304) -> ()  [unwired: 10 in, 1 out]
                  }
                  frame #1 {
                  }
                }
              }
              frame "Direction" {
                n137 = property on="UUT" class="DigNum (strict)"() -> ("Value"=w311:u8)  [unwired: 2 in, 2 out]
                n138 = while {
                  shift-right: [w331] -> w314
                  shift-left: T7."MD[1]=0" -> [w332]
                  tunnel: w312 -> [w329]
                  tunnel: w320 -> [w328]
                  tunnel: w319 -> [w327]
                  tunnel: w318 -> [w326]
                  tunnel: w317 -> [w325]
                  tunnel: w316 -> [w324]
                  tunnel: w311 -> [w323]
                  stop <- w330 stop-if-true
                  n139 = case shown="\"MD[1]=1\"" w332 {
                    tunnel: [T7."Stop" w356 w393 w463 w491 w561] -> w331
                    tunnel: [TRUE FALSE FALSE FALSE FALSE FALSE] -> w330
                    tunnel: w329 -> [_ _ _ _ _ _]
                    tunnel: w328 -> [_ w343 w370 w433 w471 w529]
                    tunnel: w327 -> [_ _ w369 w442 w470 w539]
                    tunnel: w326 -> [_ _ w386 w431 w485 w535]
                    tunnel: w325 -> [_ _ w381 w450 w483 w547]
                    tunnel: w324 -> [_ w347 _ _ _ _]
                    tunnel: w323 -> [_ w335 w367 _ w465 _]
                    frame "Stop", Default {
                    }
                    frame "Result" {
                      n140 = property on="FullSpeed1 Current" class="DigNum (strict)"() -> ("Value"=w351:dbl)  [unwired: 2 in, 2 out]
                      n141 = property on="FullSpeed2 Current" class="DigNum (strict)"() -> ("Value"=w352:dbl)  [unwired: 2 in, 2 out]
                      n142 = property on="FullSpeed2 Speed" class="DigNum (strict)"() -> ("Value"=w354:dbl)  [unwired: 2 in, 2 out]
                      n143 = property on="FullSpeed1 Speed" class="DigNum (strict)"() -> ("Value"=w353:dbl)  [unwired: 2 in, 2 out]
                      n144 = Subtract(x=w352, y=w351) -> (x-y=w350:dbl)
                      n145 = Absolute Value(x=w350) -> (abs(x)=w339:dbl)
                      n146 = Greater Or Equal?(x=w339, y=u32 5) -> (x >= y?=w345:bool)
                      n147 = Equal?(x=w335, y=u8 95) -> (x = y?=w337:bool)
                      n148 = case shown="True" w337 {
                        tunnel: w354 -> [_ w365]
                        tunnel: w353 -> [_ w364]
                        tunnel: [TRUE w361] -> w346
                        frame False {
                        }
                        frame True {
                          n149 = Subtract(x=w365, y=w364) -> (x-y=w366:dbl)
                          n150 = Absolute Value(x=w366) -> (abs(x)=w363:dbl)
                          n151 = Greater Or Equal?(x=w363, y=500.0) -> (x >= y?=w361:bool)
                        }
                      }
                      n152 = call "Find_Number_LineMARVIN.vi"("Test Paragraph"="Motor Rotation Direction", "TableIn"=w347) -> ("Line number"=w344:i32)  [unwired: 3 in, 3 out]
                      n153 = And(x=w346, y=w345) -> (x .and. y?=w336:bool)
                      "VenableDirectionResult" <- w336
                      n154 = call "PassOrFail (SubVI).vi"("String Res"="", "index (row)"=w344, "Data in"=-3.0, "Pass?Fail"=w336, "Table in"=w347) -> ("error out"=w342:errorcluster)  [unwired: 6 in]
                      n155 = property class="Bool (strict)"(reference=w343, error in=w342) -> ("Value"=w359:bool)  [unwired: 2 out]
                      n156 = Select(t=T7."Stop", s=w359, f=T7."Stop") -> (s? t:f=w356:T7)
                    }
                    frame "FullSpeed2" {
                      (unwired) TRUE ("Remote")
                      n157 = Concatenate Strings(w381, "\nFull speed operation " ("string")) -> (w368:string)
                      n158 = call "CANSendMessage.vi"() -> ("error out"=w388:errorcluster)  [unwired: 11 in]
                      n159 = call "Write panel message Kinetics (SubVI).vi"(4:"rpm"=w386, 5:"rpm"=TRUE ("rpm"), "PrintTime"=FALSE, "Stop"=w370, "error in (no error)"=w388, "Time to wait"=0.2, "Strin"=w368, "String in"=w369) -> ("error out"=w373:errorcluster)  [unwired: 3 in]
                      n160 = Equal?(x=w367, y=u8 95) -> (x = y?=w376:bool)
                      n161 = Select(t=u16 15100, s=w376, f=u16 12100 ("y")) -> ()  [unwired: 1 out]
                      n162 = flat-sequence {
                        tunnel: w373 -> [w398]
                        tunnel: [w398] -> w372
                        tunnel: [w397] -> w371
                        frame #0 {
                          n163 = call <vilib>:"High Resolution Relative Seconds.vi"() -> ("relative seconds"=w397:dbl)
                        }
                      }
                      n164 = Select(t=14500.0, s=w376, f=11500.0) -> (s? t:f=w375:dbl)
                      n165 = Select(t=47.0, s=w376, f=24.0) -> (s? t:f=w374:dbl)
                      n166 = while {
                        tunnel: w386 -> [w400]
                        tunnel: w372 -> [w424]
                        tunnel: [w407] -> w383
                        tunnel: w375 -> [w420]
                        tunnel: w374 -> [w419]
                        tunnel: w371 -> [w415]
                        tunnel: w370 -> [w405]
                        tunnel: w369 -> [w406]
                        tunnel: w368 -> [w403]
                        stop <- w417 stop-if-true
                        n167 = call <vilib>:"High Resolution Relative Seconds.vi"() -> ("relative seconds"=w416:dbl)
                        n168 = Subtract(x=w416, y=w415) -> (x-y=w414:dbl)
                        n169 = property class="DigNum (strict)"(reference=w400, error in=w424) -> ("Value"=w421:dbl)  [unwired: 2 out]
                        "FullSpeed2 Speed" <- w421
                        n170 = Greater Or Equal?(x=w414, y=120.0) -> (x >= y?=w412:bool)
                        n171 = Greater Or Equal?(x=w421, y=w420) -> (x >= y?=w411:bool)
                        n172 = property class="Bool (strict)"(reference=w405) -> ("Value"=w410:bool)  [unwired: 1 in, 2 out]
                        n173 = call "GetADCTester (SubVI).vi"("GetADCTester"=T8."Current", "TimeToGet"=5) -> ("error out"=w422:errorcluster, "ADCValOutput Single"=w418:dbl)  [unwired: 7 in, 1 out]
                        "FullSpeed2 Current" <- w418
                        n174 = Greater Or Equal?(x=w418, y=w419) -> (x >= y?=w408:bool)
                        n175 = And(x=w411, y=w408) -> (x .and. y?=w409:bool)
                        n176 = Compound Arithmetic op=OR(w410, w412, w409) -> (w417:bool)
                        n177 = call "Write panel message Kinetics (SubVI).vi"(4:"rpm"=w400, 5:"rpm"=TRUE ("rpm"), "PrintTime"=FALSE, "Stop"=w405, "error in (no error)"=w422, "Time to wait"=0.2, "Strin"=w403, "String in"=w406) -> ("error out"=w407:errorcluster)  [unwired: 3 in]
                      }
                      n178 = property class="Bool (strict)"(reference=w370, error in=w383) -> ("Value"=w396:bool)  [unwired: 2 out]
                      n179 = Select(t=T7."Stop", s=w396, f=T7."Result") -> (s? t:f=w393:T7)
                    }
                    frame "MD[1]=1" {
                      (unwired) TRUE ("Remote")
                      (unwired) u16 0 ("Motor Speed RPM")
                      n180 = Concatenate Strings(w450, "\nSet Parameters MD[1]=1" ("Strin")) -> (w441:string)
                      n181 = call "TesterOption (SubVI).vi"("2 Options"=FALSE, "On/Off"=FALSE, "Tester Option"=T6."Venable") -> ("error out"=w455:errorcluster, "VISA Refnum out"=w446:refnum<visa-resource-name>)  [unwired: 7 in]
                      n182 = call "CANSendMessage.vi"("error in (no error)"=w455) -> ("error out"=w457:errorcluster)  [unwired: 10 in]
                      n183 = call "Write panel message Kinetics (SubVI).vi"(4:"rpm"=w431, 5:"rpm"=FALSE ("rpm"), "PrintTime"=TRUE, "Stop"=w433, "error in (no error)"=w457, "Time to wait"=20.0, "Strin"=w441, "String in"=w442) -> ("error out"=w430:errorcluster)  [unwired: 3 in]
                      n184 = property on="VISA Kinetics" class="VISAName"(error in=w430) -> (error out=w456:errorcluster, "Value"=w459:refnum<visa-resource-name>)  [unwired: 1 in, 1 out]
                      n185 = call "SerialMarvinSendGet.vi"("error in (no error)"=w456, "Clear Log"=FALSE, "write buffer"="EP=1\r\nMD[1]=1\r\n", "VISA resource name"=w459) -> ("error out"=w445:errorcluster)  [unwired: 6 in, 1 out]
                      n186 = call "TesterOption (SubVI).vi"("2 Options"=FALSE, "error in (no error)"=w445, "On/Off"=FALSE, "Tester Option"=T6."Power", "VISA Refnum in"=w446) -> ("error out"=w443:errorcluster, "VISA Refnum out"=w434:refnum<visa-resource-name>)  [unwired: 5 in]
                      n187 = call "Write panel message Kinetics (SubVI).vi"(4:"rpm"=w431, 5:"rpm"=FALSE ("rpm"), "PrintTime"=TRUE, "Stop"=w433, "error in (no error)"=w443, "Time to wait"=25.0, "Strin"=w441, "String in"=w442) -> ("error out"=w435:errorcluster)  [unwired: 3 in]
                      n188 = call "TesterOption (SubVI).vi"("2 Options"=FALSE, "error in (no error)"=w435, "On/Off"=TRUE, "Tester Option"=T6."Venable", "VISA Refnum in"=w434) -> ("error out"=w432:errorcluster)  [unwired: 5 in, 1 out]
                      n189 = call "Time Delay8"("error in (no error)"=w432) -> ("error out"=w428:errorcluster)  [unwired: 10 in]
                      n190 = property class="Bool (strict)"(reference=w433, error in=w428) -> ("Value"=w464:bool)  [unwired: 2 out]
                      n191 = Select(t=T7."Stop", s=w464, f=T7."FullSpeed2") -> (s? t:f=w463:T7)
                    }
                    frame "FullSpeed1" {
                      (unwired) TRUE ("Remote")
                      n192 = call "CANSendMessage.vi"() -> ("error out"=w486:errorcluster)  [unwired: 11 in]
                      n193 = Concatenate Strings(w483, "\nFull speed operation " ("string")) -> (w469:string)
                      n194 = call "Write panel message Kinetics (SubVI).vi"(4:"rpm"=w485, 5:"rpm"=TRUE ("rpm"), "PrintTime"=FALSE, "Stop"=w471, "error in (no error)"=w486, "Time to wait"=0.2, "Strin"=w469, "String in"=w470) -> ("error out"=w474:errorcluster)  [unwired: 3 in]
                      n195 = Equal?(x=w465, y=u8 95) -> (x = y?=w481:bool)
                      n196 = flat-sequence {
                        tunnel: w474 -> [w496]
                        tunnel: [w496] -> w473
                        tunnel: [w495] -> w472
                        frame #0 {
                          n197 = call <vilib>:"High Resolution Relative Seconds.vi"() -> ("relative seconds"=w495:dbl)
                        }
                      }
                      n198 = Select(t=u16 15100, s=w481, f=u16 12100 ("y")) -> ()  [unwired: 1 out]
                      n199 = Select(t=13700.0, s=w481, f=11500.0) -> (s? t:f=w476:dbl)
                      n200 = Select(t=56.0, s=w481, f=33.0) -> (s? t:f=w475:dbl)
                      n201 = while {
                        tunnel: w485 -> [w498]
                        tunnel: w473 -> [w522]
                        tunnel: [w505] -> w484
                        tunnel: w476 -> [w517]
                        tunnel: w475 -> [w514]
                        tunnel: w472 -> [w512]
                        tunnel: w471 -> [w503]
                        tunnel: w470 -> [w504]
                        tunnel: w469 -> [w501]
                        stop <- w519 stop-if-true
                        n202 = property class="DigNum (strict)"(reference=w498, error in=w522) -> ("Value"=w518:dbl)  [unwired: 2 out]
                        "FullSpeed1 Speed" <- w518
                        n203 = call <vilib>:"High Resolution Relative Seconds.vi"() -> ("relative seconds"=w513:dbl)
                        n204 = Subtract(x=w513, y=w512) -> (x-y=w511:dbl)
                        n205 = Greater Or Equal?(x=w511, y=120.0) -> (x >= y?=w509:bool)
                        n206 = Greater Or Equal?(x=w518, y=w517) -> (x >= y?=w516:bool)
                        n207 = call "GetADCTester (SubVI).vi"("GetADCTester"=T8."Current", "TimeToGet"=5) -> ("error out"=w520:errorcluster, "ADCValOutput Single"=w515:dbl)  [unwired: 7 in, 1 out]
                        "FullSpeed1 Current" <- w515
                        n208 = Greater Or Equal?(x=w515, y=w514) -> (x >= y?=w506:bool)
                        n209 = And(x=w506, y=w516) -> (x .and. y?=w507:bool)
                        n210 = property class="Bool (strict)"(reference=w503) -> ("Value"=w508:bool)  [unwired: 1 in, 2 out]
                        n211 = call "Write panel message Kinetics (SubVI).vi"(4:"rpm"=w498, 5:"rpm"=TRUE ("rpm"), "PrintTime"=FALSE, "Stop"=w503, "error in (no error)"=w520, "Time to wait"=0.2, "Strin"=w501, "String in"=w504) -> ("error out"=w505:errorcluster)  [unwired: 3 in]
                        n212 = Compound Arithmetic op=OR(w508, w507, w509) -> (w519:bool)
                      }
                      n213 = property class="Bool (strict)"(reference=w471, error in=w484) -> ("Value"=w494:bool)  [unwired: 2 out]
                      n214 = Select(t=T7."Stop", s=w494, f=T7."MD[1]=1") -> (s? t:f=w491:T7)
                    }
                    frame "MD[1]=0" {
                      (unwired) TRUE ("Remote")
                      (unwired) u16 0 ("Motor Speed RPM")
                      n215 = Concatenate Strings(w547, "\nSet Parameters MD[1]=0" ("Strin")) -> (w538:string)
                      n216 = call "TesterOption (SubVI).vi"("2 Options"=FALSE, "On/Off"=FALSE, "Tester Option"=T6."Venable") -> ("error out"=w553:errorcluster, "VISA Refnum out"=w543:refnum<visa-resource-name>)  [unwired: 7 in]
                      n217 = call "CANSendMessage.vi"("error in (no error)"=w553) -> ("error out"=w555:errorcluster)  [unwired: 10 in]
                      n218 = call "Write panel message Kinetics (SubVI).vi"(4:"rpm"=w535, 5:"rpm"=FALSE ("rpm"), "PrintTime"=FALSE, "Stop"=w529, "error in (no error)"=w555, "Time to wait"=0.2, "Strin"=w538, "String in"=w539) -> ("error out"=w550:errorcluster)  [unwired: 3 in]
                      n219 = property on="VISA Kinetics" class="VISAName"(error in=w550) -> (error out=w554:errorcluster, "Value"=w557:refnum<visa-resource-name>)  [unwired: 1 in, 1 out]
                      n220 = call "SerialMarvinSendGet.vi"("error in (no error)"=w554, "Clear Log"=FALSE, "write buffer"="EP=1\r\nMD[1]=0\r\n", "VISA resource name"=w557) -> ("error out"=w542:errorcluster)  [unwired: 6 in, 1 out]
                      n221 = call "TesterOption (SubVI).vi"("2 Options"=FALSE, "error in (no error)"=w542, "On/Off"=FALSE, "Tester Option"=T6."Power", "VISA Refnum in"=w543) -> ("error out"=w540:errorcluster, "VISA Refnum out"=w530:refnum<visa-resource-name>)  [unwired: 5 in]
                      n222 = call "Write panel message Kinetics (SubVI).vi"(4:"rpm"=w535, 5:"rpm"=FALSE ("rpm"), "PrintTime"=TRUE, "Stop"=w529, "error in (no error)"=w540, "Time to wait"=25.0, "Strin"=w538, "String in"=w539) -> ("error out"=w531:errorcluster)  [unwired: 3 in]
                      n223 = call "TesterOption (SubVI).vi"("2 Options"=FALSE, "error in (no error)"=w531, "On/Off"=TRUE, "Tester Option"=T6."Venable", "VISA Refnum in"=w530) -> ("error out"=w528:errorcluster)  [unwired: 5 in, 1 out]
                      n224 = call "Time Delay4"("error in (no error)"=w528) -> ("error out"=w524:errorcluster)  [unwired: 10 in]
                      n225 = property class="Bool (strict)"(reference=w529, error in=w524) -> ("Value"=w562:bool)  [unwired: 2 out]
                      n226 = Select(t=T7."Stop", s=w562, f=T7."FullSpeed1") -> (s? t:f=w561:T7)
                    }
                  }
                }
                n227 = flat-sequence {
                  tunnel: [enum16{"Stop", "Direction", "Venable", "Start"}."Stop"] -> w315
                  tunnel: w314 -> [_]
                  frame #0 {
                  }
                }
              }
              frame "Venable" {
                n228 = call "Find_Number_LineMARVIN.vi"("Test Paragraph"="Enable Test", "TableIn"=w567) -> ("Line number"=w573:i32)  [unwired: 3 in, 3 out]
                n229 = Increment(x=w573) -> (x+1=w563:i32)
                n230 = for {
                  tunnel: u16[] [5000, 0, 5000] -> [w598] mode=indexing
                  tunnel: bool[] [TRUE, FALSE, TRUE] -> [w596] mode=indexing
                  tunnel: w563 -> [w599]
                  tunnel: w572 -> [_]
                  tunnel: w571 -> [w589]
                  tunnel: w570 -> [w592]
                  tunnel: w569 -> [w591]
                  tunnel: w567 -> [w585]
                  tunnel: w566 -> [w583]
                  tunnel: [w582] -> w565 mode=indexing
                  i -> [w600]
                  (unwired) u16 5000 ("Motor Speed RPM")
                  (unwired) TRUE ("Remote")
                  w601 = 200.0 ("y")
                  n231 = call "CANSendMessage.vi"() -> ("error out"=w595:errorcluster)  [unwired: 11 in]
                  n232 = Add(x=w599, y=w600) -> (x+y=w586:i32)
                  n233 = call "TesterOption (SubVI).vi"("2 Options"=FALSE, "error in (no error)"=w595, "On/Off"=w596, "Tester Option"=T6."Venable") -> ("error out"=w594:errorcluster)  [unwired: 6 in, 1 out]
                  n234 = call "Write panel message Kinetics (SubVI).vi"(4:"rpm"=w589, 5:"rpm"=TRUE ("rpm"), "PrintTime"=TRUE, "Stop"=w591, "error in (no error)"=w594, "Time to wait"=15.0, "Strin"=w583, "String in"=w592) -> ("error out"=w593:errorcluster)  [unwired: 3 in]
                  n235 = property class="DigNum (strict)"(reference=w589, error in=w593) -> ("Value"=w584:dbl)  [unwired: 2 out]
                  n236 = Add(x=w598, y=w601) -> (x+y=w603:dbl)
                  n237 = Subtract(x=w598, y=w601) -> (x-y=w602:dbl)
                  n238 = In Range and Coerce(upper limit=w603, x=w584, lower limit=w602) -> (In Range?=w582:bool)  [unwired: 1 out]
                  n239 = call "PassOrFail (SubVI).vi"("index (row)"=w586, "Data in"=w584, "Pass?Fail"=w582, "Table in"=w585) -> ()  [unwired: 7 in, 1 out]
                }
                n240 = property class="Bool (strict)"(reference=w569) -> ("Value"=w580:bool)  [unwired: 1 in, 2 out]
                n241 = And Array Elements(Boolean array=w565) -> (logical AND=→"VenableResult":bool)
                n242 = Select(t=enum16{"Stop", "Direction", "Venable", "Start"}."Stop", s=w580, f=enum16{"Stop", "Direction", "Venable", "Start"}."Direction") -> (s? t:f=w568:enum16{"Stop", "Direction", "Venable", "Start"})
              }
              frame "Start" {
                w619 = "Enable Test" ("Test Paragraph")
                n243 = property class="Str"(reference=w613, "Value"=w605) -> (reference out=w620:refnum<vi>, error out=w610:errorcluster)  [unwired: 1 in]
                n244 = call "Table_ScrollaBarMarvin.vi"("error in"=w610, "Line to focus"=w619, "reference in"=w614) -> ("error out"=w616:errorcluster)  [unwired: 2 out]
                n245 = call "Reset old test Values (SubVI).vi"("error in"=w616, "Atr in"=w614, "Test Paragraph"=w619) -> ()  [unwired: 8 in, 1 out]
                n246 = property class="Bool (strict)"(reference=w607) -> ("Value"=w624:bool)  [unwired: 1 in, 2 out]
                n247 = call "TesterOption (SubVI).vi"("2 Options"=FALSE, "On/Off"=TRUE, "Tester Option"=T6."Venable") -> ("error out"=w615:errorcluster)  [unwired: 7 in, 1 out]
                n248 = Select(t=enum16{"Stop", "Direction", "Venable", "Start"}."Stop", s=w624, f=enum16{"Stop", "Direction", "Venable", "Start"}."Venable") -> (s? t:f=w611:enum16{"Stop", "Direction", "Venable", "Start"})
                n249 = call "Write panel message Kinetics (SubVI).vi"(4:"rpm"=w606, 5:"rpm"=FALSE ("rpm"), "PrintTime"=FALSE, "Stop"=w607, "error in (no error)"=w615, "Time to wait"=0.2, "Strin"=w605, "String in"=w620) -> ()  [unwired: 3 in, 1 out]
              }
            }
          }
        }
        frame "Speed Command" {
          w626 = "Speed Command Test" ("Test Paragraph")
          n250 = control-ref of="Pannel User Message"() -> (w631:refnum<vi>)
          n251 = property class="Str"(reference=w631, error in=w630, "Value"="Speed Command Test in process...") -> (error out=w629:errorcluster)  [unwired: 1 out]
          n252 = call "Table_ScrollaBarMarvin.vi"("error in"=w629, "Line to focus"=w626, "reference in"=w625) -> ("error out"=w632:errorcluster)  [unwired: 2 out]
          n253 = property class="Tbl (strict)"(reference=w625, error in=w632) -> (error out=w634:errorcluster, "Value"=w635:string[][])  [unwired: 1 out]
          n254 = Index Array(array=w635, index (col)=1 ("disabled index (col)")) -> (element=w636:string[])  [unwired: 1 in]
          n255 = call "Find_Number_Line.vi"("error in"=w634, "Test Paragraph"=w626, "Row Headers[]"=w636) -> ("error out"=w627:errorcluster)  [unwired: 2 out]
          n256 = call "Reset old test Values (SubVI).vi"("error in"=w627, "Atr in"=w625, "Test Paragraph"=w626) -> ()  [unwired: 8 in, 1 out]
        }
        frame "Stop Time" {
          w640 = "Motor Temperature test in process..." ("Value")
          w638 = "Motor Termistor Input Test" ("Test Paragraph")
          n257 = control-ref of="Pannel User Message"() -> (w648:refnum<vi>)
          n258 = property class="Str"(reference=w648, error in=w647, "Value"=w640) -> (error out=w646:errorcluster)  [unwired: 1 out]
          n259 = call "Table_ScrollaBarMarvin.vi"("error in"=w646, "Line to focus"=w638, "reference in"=w637) -> ("error out"=w650:errorcluster)  [unwired: 2 out]
          n260 = property class="Tbl (strict)"(reference=w637, error in=w650) -> (reference out=w643:refnum<vi>, error out=w652:errorcluster, "Value"=w653:string[][])
          n261 = Index Array(array=w653, index (col)=1 ("disabled index (col)")) -> (element=w654:string[])  [unwired: 1 in]
          n262 = call "Find_Number_LineMARVIN.vi"("Test Paragraph"=w638, "error in"=w652, "TableIn"=w637, "Row Headers[]"=w654) -> ("error out"=w649:errorcluster, "Line number"=w642:i32)  [unwired: 1 in, 2 out]
          n263 = call "Reset old test Values (SubVI).vi"("error in"=w649, "Atr in"=w637, "Test Paragraph"=w638) -> ("error out"=w639:errorcluster)  [unwired: 8 in]
          n264 = property on="Status" class="Bool (strict)"(error in=w639) -> (error out=w644:errorcluster, "Value"=w645:bool)  [unwired: 1 in, 1 out]
          n265 = case shown="True" w645 {
            selector: w645 -> [w658 _]
            tunnel: w644 -> [w660 _]
            tunnel: w643 -> [w657 _]
            tunnel: w642 -> [w656 w663]
            tunnel: w641 -> [_ w666]
            tunnel: w640 -> [_ w664]
            frame False {
              n266 = flat-sequence {
                tunnel: w660 -> [w661]
                tunnel: [w661] -> w659
                frame #0 {
                  n267 = One Button Dialog(message="Please establish RS connection.") -> ()  [unwired: 1 in, 1 out]
                }
              }
              n268 = Increment(x=w656) -> (x+1=w655:i32)
              n269 = call "PassOrFail (SubVI).vi"("index (row)"=w655, "error in (no error)"=w659, "Pass?Fail"=w658, "Table in"=w657) -> ()  [unwired: 7 in, 1 out]
            }
            frame True {
              n270 = control-ref of="Pannel User Message"() -> (w669:refnum<vi>)
              n271 = control-ref of="ATR"() -> (w670:refnum<vi>)
              n272 = control-ref of="Motor Speed RPM"() -> (w671:refnum<vi>)
              n273 = control-ref of="UUT"() -> (w665:refnum<vi>)
              n274 = control-ref of="Stop Button"() -> (w668:refnum<vi>)
              n275 = while {
                shift-right: [w675] -> _
                shift-left: T9."Start" -> [w682]
                tunnel: w668 -> [w681]
                tunnel: w669 -> [w680]
                tunnel: w670 -> [w679]
                tunnel: w671 -> [w678]
                tunnel: w666 -> [w677]
                tunnel: w665 -> [w676]
                tunnel: w664 -> [w673]
                tunnel: w663 -> [w672]
                stop <- w674 stop-if-true
                n276 = case shown="\"Start\"" w682 {
                  tunnel: w681 -> [_ w695 w756]
                  tunnel: w680 -> [_ w703 w758]
                  tunnel: w679 -> [_ w693 _]
                  tunnel: w678 -> [_ w702 w754]
                  tunnel: w677 -> [_ w705 _]
                  tunnel: w676 -> [_ _ _]
                  tunnel: [w683 w696 w750] -> w675
                  tunnel: [w684 FALSE FALSE] -> w674
                  tunnel: w673 -> [_ w704 _]
                  tunnel: w672 -> [_ w692 _]
                  frame "Stop", Default {
                    n277 = flat-sequence {
                      tunnel: [TRUE] -> w684
                      tunnel: [T9."Stop"] -> w683
                      frame #0 {
                        n278 = call "TesterOption (SubVI).vi"("2 Options"=FALSE, "On/Off"=FALSE, "Tester Option"=T6."Venable") -> ()  [unwired: 7 in, 2 out]
                      }
                      frame #1 {
                      }
                    }
                  }
                  frame "TA[5]" {
                    w706 = T12 [enum."60C", enum."90C", enum."120C"] items=["K15", "K16", "K17", "Venable", "Firmeware", "Fan", "Power", "120C", "110C", "100C", "90C", "80C", "70C", "60C", "50C", "40C", "30C", "25C", "20C", "10C", "0C"]
                    n279 = for {
                      tunnel: w706 -> [w728] mode=indexing
                      tunnel: w705 -> [w727]
                      tunnel: w704 -> [w726]
                      tunnel: w703 -> [w725]
                      tunnel: w695 -> [w724]
                      tunnel: w702 -> [w723]
                      tunnel: dbl[] [60.0, 90.0, 120.0] -> [w713] mode=indexing
                      tunnel: [w712] -> w694
                      tunnel: w693 -> [w719]
                      tunnel: w692 -> [w718]
                      tunnel: [w707] -> w691 mode=indexing
                      i -> [w716]
                      w711 = 3.0 ("y")
                      n280 = for {
                        N: 5 -> [_]
                        tunnel: w728 -> [w730]
                        tunnel: w727 -> [w744]
                        tunnel: w726 -> [w739]
                        tunnel: w725 -> [w738]
                        tunnel: w724 -> [w737]
                        tunnel: w723 -> [w733]
                        tunnel: [w732] -> w722 mode=indexing
                        tunnel: [w731] -> w720
                        n281 = call "TesterOption (SubVI).vi"("2 Options"=FALSE, "On/Off"=TRUE, "Tester Option"=w730) -> ("error out"=w741:errorcluster)  [unwired: 7 in, 1 out]
                        n282 = call "Write panel message Kinetics (SubVI).vi"(4:"rpm"=w733, 5:"rpm"=FALSE ("rpm"), "PrintTime"=FALSE, "Stop"=w737, "error in (no error)"=w741, "Time to wait"=1.0, "Strin"=w739, "String in"=w738) -> ("error out"=w740:errorcluster)  [unwired: 3 in]
                        n283 = call "SerialMarvinSendGet.vi"("error in (no error)"=w740, "write buffer"="TA[2]\r\n", "VISA resource name"=w744) -> ("error out"=w731:errorcluster, "read buffer"=w742:string)  [unwired: 7 in]
                        n284 = Fract/Exp String To Number(string=w742) -> (number=w732:dbl)  [unwired: 3 in, 1 out]
                      }
                      n285 = Increment(x=w716) -> (x+1=w715:i32)
                      n286 = Add Array Elements(numeric array=w722) -> (sum=w721:dbl)
                      n287 = Add(x=w713, y=w711) -> (x+y=w710:dbl)
                      n288 = Subtract(x=w713, y=w711) -> (x-y=w709:dbl)
                      n289 = Divide(x=w721, y=5.0) -> (x/y=w708:dbl)
                      n290 = In Range and Coerce(upper limit=w710, x=w708, lower limit=w709) -> (In Range?=w707:bool)  [unwired: 1 out]
                      n291 = Add(x=w718, y=w715) -> (x+y=w717:i32)
                      n292 = call "PassOrFail (SubVI).vi"("index (row)"=w717, "error in (no error)"=w720, "Data in"=w708, "Pass?Fail"=w707, "Table in"=w719) -> ("error out"=w712:errorcluster)  [unwired: 6 in]
                    }
                    n293 = property class="Bool (strict)"(reference=w695, error in=w694) -> ("Value"=w700:bool)  [unwired: 2 out]
                    n294 = Select(t=T9."Stop", s=w700, f=T9."Stop") -> (s? t:f=w696:T9)
                    n295 = And Array Elements(Boolean array=w691) -> (logical AND=→"MotorTempResult":bool)
                  }
                  frame "Start" {
                    (unwired) TRUE ("Remote")
                    (unwired) u16 0 ("Motor Speed RPM")
                    n296 = call "Write panel message Kinetics (SubVI).vi"(4:"rpm"=w754, 5:"rpm"=FALSE ("rpm"), "PrintTime"=FALSE, "Stop"=w756, "Time to wait"=0.1, "Strin"="Motor Temperature test in process...\nInitialization state...", "String in"=w758) -> ("error out"=w759:errorcluster)  [unwired: 4 in]
                    n297 = call "TesterOption (SubVI).vi"("2 Options"=FALSE, "error in (no error)"=w759, "On/Off"=FALSE, "Tester Option"=T6."Venable") -> ("error out"=w760:errorcluster)  [unwired: 6 in, 1 out]
                    n298 = call "CANSendMessage.vi"("error in (no error)"=w760) -> ("error out"=w748:errorcluster)  [unwired: 10 in]
                    n299 = property class="Bool (strict)"(reference=w756, error in=w748) -> ("Value"=w764:bool)  [unwired: 2 out]
                    n300 = Select(t=T9."Stop", s=w764, f=T9."TA[5]") -> (s? t:f=w750:T9)
                  }
                }
              }
            }
          }
        }
        frame "Temp Control" {
          w782 = "Temperature control test in process..." ("Value")
          w780 = "Temperature Control Algorithm Test" ("Test Paragraph")
          n301 = control-ref of="Pannel User Message"() -> (w791:refnum<vi>)
          n302 = call <vilib>:"Open Config Data.vi"("error in (no error)"=w776, "create file if necessary (T)"=FALSE, "configuration file path"=w778) -> ("error out"=w779:errorcluster, "refnum"=w775:T5)  [unwired: 7 out]
          n303 = property class="Str"(reference=w791, error in=w776, "Value"=w782) -> (error out=w790:errorcluster)  [unwired: 1 out]
          n304 = call-poly <vilib>:"Read Key.vi"("section"="Marvin", "error in (no error)"=w779, "default value"="10", "key"="Temp Algorithm", "refnum"=w775) -> ("error out"=w771:errorcluster, "value"=w769:string, "refnum out"=w770:T5)  [unwired: 1 in, 3 out]
          n305 = Decimal String To Number(string=w769) -> (number=w767:i32)  [unwired: 2 in, 1 out]
          n306 = Less Or Equal To 0?(x=w767) -> (x <= 0?=w768:bool)
          n307 = Select(t=10, s=w768, f=w767) -> (s? t:f=w766:i32)
          n308 = call <vilib>:"Close Config Data.vi"("error in (no error)"=w771, "refnum"=w770) -> ()  [unwired: 8 in, 2 out]
          n309 = control-ref of="Pannel User Message"() -> (w785:refnum<vi>)
          n310 = control-ref of="Motor Speed RPM"() -> (w784:refnum<vi>)
          n311 = control-ref of="Stop Button"() -> (w787:refnum<vi>)
          n312 = control-ref of="ATR"() -> (w786:refnum<vi>)
          n313 = control-ref of="UUT"() -> (w783:refnum<vi>)
          n314 = call "Table_ScrollaBarMarvin.vi"("error in"=w790, "Line to focus"=w780, "reference in"=w792) -> ("error out"=w789:errorcluster)  [unwired: 2 out]
          n315 = call "Reset old test Values (SubVI).vi"("error in"=w789, "Atr in"=w792, "Test Paragraph"=w780) -> ("error out"=w781:errorcluster)  [unwired: 8 in]
          n316 = while {
            tunnel: w781 -> [w803]
            shift-right: [w801] -> _
            shift-left: enum16{"Stop", "Algorithm", "Start"}."Start" -> [w802]
            tunnel: w787 -> [w800]
            tunnel: w786 -> [w799]
            tunnel: w785 -> [w798]
            tunnel: w784 -> [w797]
            tunnel: w783 -> [w796]
            tunnel: w782 -> [w794]
            tunnel: w766 -> [w793]
            stop <- w795 stop-if-true
            n317 = case shown="\"Algorithm\"" w802 {
              tunnel: w803 -> [_ _ w918]
              tunnel: [w804 w819 w908] -> w801
              tunnel: w800 -> [_ w829 w912]
              tunnel: w799 -> [_ w826 _]
              tunnel: w798 -> [_ w830 _]
              tunnel: w797 -> [_ w827 _]
              tunnel: w796 -> [w806 _ _]
              tunnel: [w805 FALSE FALSE] -> w795
              tunnel: w794 -> [_ w828 _]
              tunnel: w793 -> [_ w813 _]
              frame "Stop", Default {
                n318 = flat-sequence {
                  tunnel: w806 -> [_]
                  tunnel: [TRUE] -> w805
                  tunnel: [enum16{"Stop", "Algorithm", "Start"}."Stop"] -> w804
                  frame #0 {
                    (unwired) u16 0 ("Motor Speed RPM")
                    (unwired) TRUE ("Remote")
                    n319 = call "CANSendMessage.vi"() -> ("error out"=w807:errorcluster)  [unwired: 11 in]
                    n320 = call "TesterOption (SubVI).vi"("2 Options"=FALSE, "error in (no error)"=w807, "On/Off"=FALSE, "Tester Option"=T6."Venable") -> ()  [unwired: 6 in, 2 out]
                  }
                  frame #1 {
                  }
                  frame #2 {
                  }
                }
              }
              frame "Algorithm" {
                w814 = T13 [enum."6000", enum."11500", enum."15100", enum."11500-2", enum."6000-2"] items=["6000", "11500", "15100", "11500-2", "6000-2"]
                # "Speed Goal"
                # "Speed Ind"
                # "Temp Goal"
                # "50 Deg"
                n321 = for {
                  tunnel: w830 -> [w857]
                  tunnel: w829 -> [w856]
                  tunnel: w828 -> [w855]
                  tunnel: w827 -> [w854]
                  tunnel: w826 -> [w841]
                  tunnel: string[] ["Tair <   67 ± 3 °C", "Tair >= 67 ± 3 °C", "Tair >= 83 ± 3 °C", "Tair <= 80 ± 3 °C", "Tair <= 64 ± 3 °C"] -> [w839] mode=indexing
                  shift-right: [w851] -> _
                  shift-left: 1202.0 ("Rt") -> [w852]
                  tunnel: dbl[] [67.0, 67.0, 83.0, 80.0, 64.0] -> [w850] mode=indexing
                  tunnel: dbl[] [11500.0, 12700.0, 14700.0, 12700.0, 11500.0] -> [w849] mode=indexing
                  tunnel: dbl[] [11500.0, 11900.0, 13000.0, 13900.0, 12200.0] -> [w848] mode=indexing
                  tunnel: [w837] -> w820
                  tunnel: [w836] -> w816 mode=indexing
                  tunnel: [w835] -> w817 mode=indexing
                  tunnel: w814 -> [w834] mode=indexing
                  tunnel: w813 -> [w833]
                  stop <- w853 stop-if-true
                  n322 = call <vilib>:"High Resolution Relative Seconds.vi"() -> ("relative seconds"=w847:dbl)
                  n323 = while {
                    tunnel: w857 -> [w886]
                    tunnel: w856 -> [w879]
                    tunnel: w855 -> [w865]
                    tunnel: w854 -> [w887]
                    shift-right: [w884] -> w851
                    shift-left: w852 -> [w883]
                    tunnel: w834 -> [w885]
                    tunnel: w850 -> [w882]
                    tunnel: w849 -> [w881]
                    tunnel: w848 -> [w880]
                    tunnel: w847 -> [w876]
                    tunnel: [w871] -> w842
                    tunnel: [w870] -> w835
                    tunnel: [w869] -> w840
                    tunnel: [w868] -> w836
                    tunnel: [w867] -> w838
                    tunnel: w833 -> [w859]
                    stop <- w877 stop-if-true
                    n324 = call "DegToDAC (SubVI).vi"("R2"=0.0, "Rt"=w883) -> ("error out"=w858:errorcluster, "output array"=w893:u8[])  [unwired: 8 in]
                    n325 = call <vilib>:"High Resolution Relative Seconds.vi"() -> ("relative seconds"=w875:dbl)
                    n326 = Byte Array To String(unsigned byte array=w893) -> ()  [unwired: 1 out]
                    n327 = Subtract(x=w876, y=w875) -> (x-y=w874:dbl)
                    n328 = Greater Or Equal?(x=w874, y=120.0) -> (x >= y?=w872:bool)
                    n329 = call <vilib>:"Clear Errors.vi"("error in (no error)"=w858) -> ("error out"=w892:errorcluster)  [unwired: 5 in, 1 out]
                    n330 = control-ref of="Ambient Temperature"() -> (w866:refnum<vi>)
                    n331 = property class="DigNum (strict)"(reference=w866) -> ("Value"=w864:dbl)  [unwired: 1 in, 2 out]
                    n332 = property class="Bool (strict)"(reference=w879) -> ("Value"=w878:bool)  [unwired: 1 in, 2 out]
                    n333 = Number To Fractional String(number=w864, precision (6)=i16 2) -> (F-format string=w861:string)  [unwired: 2 in]
                    n334 = Concatenate Strings(w865, "\nAmbient  Temp. [C]: " ("string"), w861) -> (w860:string)
                    n335 = call "Write panel message Kinetics (SubVI).vi"(4:"rpm"=w887, 5:"rpm"=TRUE ("rpm"), "PrintTime"=TRUE, "Stop"=w879, "error in (no error)"=w892, "Time to wait"=5.0, "Strin"=w860, "String in"=w886) -> ("error out"=w891:errorcluster)  [unwired: 3 in]
                    n336 = call "TempAlgoTest (SubVI).vi"("Temp"=w866, "Speed Ind"=w880, "Motor Speed RPM"=w887, "Round"=w885, "Temp Up In"=w883, "error in (no error)"=w891, "String in"=w886, "Temp Goal"=w882, "Stop"=w879, "Speed Goal"=w881, "AD Resistor Step"=w859, "Strin"=w860) -> (14:"Speed Pass/Fail"=w870:bool, "Temp  Pass/Fail"=w869:dbl, "Temp Up Out"=w884:dbl, 17:"Speed Pass/Fail"=w871:dbl, "Temp Pass/Fail"=w868:bool, "error out"=w867:errorcluster)  [unwired: 2 in]
                    n337 = Compound Arithmetic op=OR(w872, w870, w878) -> (w877:bool)
                  }
                  n338 = property class="Bool (strict)"(reference=w856) -> ("Value"=w853:bool)  [unwired: 1 in, 2 out]
                  n339 = call "Find_Number_LineMARVIN.vi"("Test Paragraph"=w839, "error in"=w838, "TableIn"=w841) -> ("error out"=w843:errorcluster, "Line number"=w846:i32)  [unwired: 2 in, 2 out]
                  n340 = Increment(x=w846) -> (x+1=w845:i32)
                  n341 = call "PassOrFail (SubVI).vi"("index (row)"=w845, "error in (no error)"=w843, "Data in"=w840, "Pass?Fail"=w836, "Table in"=w841) -> ("error out"=w844:errorcluster)  [unwired: 6 in]
                  n342 = call "PassOrFail (SubVI).vi"("index (row)"=w846, "error in (no error)"=w844, "Data in"=w842, "Pass?Fail"=w835, "Table in"=w841) -> ("error out"=w837:errorcluster)  [unwired: 6 in]
                }
                n343 = Build Array (concatenate)(w817, w816) -> (w818:bool[])
                n344 = flat-sequence {
                  tunnel: w820 -> [_]
                  tunnel: [enum16{"Stop", "Algorithm", "Start"}."Stop"] -> w819
                  frame #0 {
                  }
                }
                n345 = And Array Elements(Boolean array=w818) -> (logical AND=→"TempControlResult":bool)
              }
              frame "Start" {
                (unwired) u16 0 ("Motor Speed RPM")
                (unwired) TRUE ("Remote")
                (unwired) u16 0 ("Motor Speed RPM")
                (unwired) FALSE ("Remote")
                n346 = call <vilib>:"Clear Errors.vi"("error in (no error)"=w918) -> ("error out"=w901:errorcluster)  [unwired: 5 in, 1 out]
                n347 = call "CANSendMessage.vi"("error in (no error)"=w901) -> ("error out"=w899:errorcluster)  [unwired: 10 in]
                n348 = call "Time Delay15"("error in (no error)"=w899) -> ("error out"=w898:errorcluster)  [unwired: 10 in]
                n349 = call "DegToDAC (SubVI).vi"("error in (no error)"=w898, "R2"=0.0, "Rt"=1202.0) -> ("error out"=w895:errorcluster, "output array"=w904:u8[])  [unwired: 7 in]
                n350 = Byte Array To String(unsigned byte array=w904) -> ()  [unwired: 1 out]
                n351 = call "Time Delay16"("error in (no error)"=w895) -> ("error out"=w900:errorcluster)  [unwired: 10 in]
                n352 = call "TesterOption (SubVI).vi"("On/Off 2"=TRUE, "Tester Option 2"=T6."Venable", "2 Options"=TRUE, "error in (no error)"=w900, "On/Off"=TRUE, "Tester Option"=T6."K16") -> ("error out"=w906:errorcluster)  [unwired: 4 in, 1 out]
                n353 = call "Time Delay12"("error in (no error)"=w906) -> ("error out"=w905:errorcluster)  [unwired: 10 in]
                n354 = call "CANSendMessage.vi"("error in (no error)"=w905) -> ("error out"=w897:errorcluster)  [unwired: 10 in]
                n355 = call "Time Delay17"("error in (no error)"=w897) -> ("error out"=w896:errorcluster)  [unwired: 10 in]
                n356 = property class="Bool (strict)"(reference=w912, error in=w896) -> ("Value"=w911:bool)  [unwired: 2 out]
                n357 = Select(t=enum16{"Stop", "Algorithm", "Start"}."Stop", s=w911, f=enum16{"Stop", "Algorithm", "Start"}."Algorithm") -> (s? t:f=w908:enum16{"Stop", "Algorithm", "Start"})
              }
            }
          }
        }
        frame "Burn in" {
          n358 = control-ref of="Stop Button"() -> (w923:refnum<vi>)
          n359 = control-ref of="Pannel User Message"() -> (w925:refnum<vi>)
          n360 = control-ref of="ATR"() -> (w922:refnum<vi>)
          n361 = control-ref of="UUT"() -> (w924:refnum<vi>)
          n362 = property on="UUT" class="DigNum (strict)"() -> ("Value"=w921:u8)  [unwired: 2 in, 2 out]
          n363 = while {
            tunnel: w925 -> [w937]
            tunnel: w922 -> [w936]
            tunnel: w924 -> [w935]
            tunnel: w923 -> [w934]
            shift-right: [w933] -> _
            shift-left: T10."Start" -> [w939]
            shift-right: [w938] -> _
            shift-left: _ -> [w931]
            tunnel: w921 -> [w930]
            tunnel: w920 -> [w929]
            shift-right: [w928] -> _
            shift-left: FALSE -> [w927]
            stop <- w932 stop-if-true
            n364 = case shown="\"Ambient Temp\"" w939 {
              tunnel: [w944 w969 w1032 w1059 w1088 w1118] -> w938
              tunnel: w937 -> [_ w962 _ _ _ w1117]
              tunnel: w936 -> [_ w965 w1005 w1046 w1075 w1105]
              tunnel: w935 -> [w940 w959 _ _ _ _]
              tunnel: w934 -> [_ _ w1034 w1061 w1091 w1111]
              tunnel: [w942 T10."Stop" w1035 w1062 w1092 w1107] -> w933
              tunnel: [w943 FALSE FALSE FALSE FALSE FALSE] -> w932
              tunnel: w931 -> [w944 w969 w1032 w1059 w1088 _]
              tunnel: w930 -> [_ w956 w999 w1041 w1070 w1099]
              tunnel: w929 -> [_ _ _ _ _ _]
              tunnel: [FALSE ("Stop Burn-in") FALSE ("Stop Burn-in") FALSE w1039 w1067 FALSE ("Stop Burn-in")] -> w928
              tunnel: w927 -> [_ _ w994 _ _ _]
              frame "Stop", Default {
                n365 = flat-sequence {
                  tunnel: w940 -> [_]
                  tunnel: [TRUE] -> w943
                  tunnel: [T10."Stop"] -> w942
                  frame #0 {
                    (unwired) u16 0 ("Motor Speed RPM")
                    (unwired) TRUE ("Remote")
                    (unwired) FALSE ("Visible")
                    n366 = call "CANSendMessage.vi"() -> ("error out"=w945:errorcluster)  [unwired: 11 in]
                    n367 = call "TesterOption (SubVI).vi"("2 Options"=FALSE, "error in (no error)"=w945, "On/Off"=FALSE, "Tester Option"=T6."Venable") -> ()  [unwired: 6 in, 2 out]
                  }
                  frame #1 {
                  }
                }
              }
              frame "BurnIn" {
                n368 = control-ref of="Motor Speed RPM"() -> (w964:refnum<vi>)
                n369 = control-ref of="Stop Button"() -> (w963:refnum<vi>)
                n370 = Equal?(x=w956, y=u8 95) -> (x = y?=w955:bool)
                n371 = call "Find_Number_LineMARVIN.vi"("Test Paragraph"="After 10 min of operation", "TableIn"=w965) -> ("error out"=w967:errorcluster, "Line number"=w968:i32)  [unwired: 3 in, 2 out]
                n372 = Select(t=u16 14700, s=w955, f=u16 12100 ("y")) -> (s? t:f=w957:u16)
                n373 = for {
                  tunnel: w967 -> [w981]
                  tunnel: dbl[] [600.0, 600.0, 600.0] -> [w985] mode=indexing
                  tunnel: w968 -> [w990]
                  tunnel: w965 -> [w980]
                  tunnel: w964 -> [w979]
                  tunnel: w963 -> [w978]
                  tunnel: w962 -> [w977]
                  tunnel: w959 -> [_]
                  tunnel: w957 -> [_]
                  tunnel: [w974] -> _
                  tunnel: [w973] -> w954 mode=indexing
                  i -> [w987]
                  (unwired) TRUE ("Remote")
                  n374 = call "CANSendMessage.vi"("error in (no error)"=w981) -> ("error out"=w976:errorcluster)  [unwired: 10 in]
                  n375 = Add(x=w990, y=w987) -> (x+y=w986:i32)
                  n376 = call "Write panel message Kinetics (SubVI).vi"(4:"rpm"=w979, 5:"rpm"=TRUE ("rpm"), "PrintTime"=TRUE, "Stop"=w978, "error in (no error)"=w976, "Time to wait"=w985, "Strin"="Burn-in test in process...", "String in"=w977) -> ("error out"=w982:errorcluster)  [unwired: 3 in]
                  n377 = control-ref of="Power transistor Heat sink Temp."() -> (w991:refnum<vi>)
                  n378 = property on="MaxBurnInTempVal" class="DigNum (strict)"() -> ("Value"=w989:dbl)  [unwired: 2 in, 2 out]
                  n379 = property class="DigNum (strict)"(reference=w991, error in=w982) -> (error out=w975:errorcluster, "Value"=w988:dbl)  [unwired: 1 out]
                  n380 = Less Or Equal?(x=w988, y=w989) -> (x <= y?=w973:bool)
                  n381 = call "PassOrFail (SubVI).vi"("index (row)"=w986, "error in (no error)"=w975, "Data in"=w988, "Pass?Fail"=w973, "Table in"=w980) -> ("error out"=w974:errorcluster)  [unwired: 6 in]
                }
                n382 = And Array Elements(Boolean array=w954) -> (logical AND=→"BurnResult":bool)
              }
              frame "Ambient Temp" {
                w1010 = 2 ("disabled index (col)")
                n383 = control-ref of="Power transistor Heat sink Temp."() -> (w1020:refnum<vi>)
                n384 = call "Find_Number_LineMARVIN.vi"("Test Paragraph"="Ambient Temperature", "TableIn"=w1005) -> ("error out"=w1031:errorcluster, "Line number"=w1011:i32)  [unwired: 3 in, 2 out]
                n385 = Equal?(x=w999, y=u8 95) -> (x = y?=w1000:bool)
                n386 = property class="DigNum (strict)"(reference=w1020, error in=w1031) -> (error out=w1022:errorcluster, "Value"=w1012:dbl)  [unwired: 1 out]
                n387 = Select(t=25.0 ("y"), s=w1000, f=25.0 ("y")) -> (s? t:f=w1021:dbl)
                n388 = Select(t=13.0 ("y"), s=w1000, f=13.0) -> (s? t:f=w1023:dbl)
                n389 = Add(x=w1021, y=w1023) -> (x+y=w1030:dbl)
                n390 = Subtract(x=w1021, y=w1023) -> (x-y=w1029:dbl)
                n391 = In Range and Coerce(upper limit=w1030, x=w1012, lower limit=w1029) -> (In Range?=w996:bool)  [unwired: 1 out]
                "BurnTemp" <- w996
                n392 = call "PassOrFail (SubVI).vi"("index (row)"=w1011, "error in (no error)"=w1022, "Data in"=w1012, "Pass?Fail"=w996, "Table in"=w1005) -> ("error out"=w1002:errorcluster)  [unwired: 6 in]
                n393 = property class="Tbl (strict)"(reference=w1005, error in=w1002) -> (reference out=w1004:refnum<vi>, error out=w1019:errorcluster, "Value"=w1018:string[][])
                n394 = Add(x=w1012, y=25.0) -> (x+y=w1003:dbl)
                "MaxBurnInTempVal" <- w1003
                n395 = Number To Fractional String(number=w1003, precision (6)=i16 0) -> (F-format string=w1017:string)  [unwired: 2 in]
                n396 = Concatenate Strings("< " ("string"), w1017) -> (w1006:string)
                n397 = Increment(x=w1011) -> (x+1=w1009:i32)
                n398 = Increment(x=w1009) -> (x+1=w1008:i32)
                n399 = Increment(x=w1008) -> (x+1=w1007:i32)
                n400 = Replace Array Subset(array=w1018, new element #1=w1006, index (row) #1=w1009, index (col) #1=w1010, new element #2=w1006, index (row) #2=w1008, index (col) #2=w1010, new element #3=w1006, index (row) #3=w1007, index (col) #3=w1010) -> (w1016:string[][])
                n401 = Not(x=w996) -> (.not. x?=w995:bool)
                n402 = property class="Tbl (strict)"(reference=w1004, error in=w1019, "Value"=w1016) -> (error out=w1001:errorcluster)  [unwired: 1 out]
                n403 = property class="Bool (strict)"(reference=w1034, error in=w1001) -> ("Value"=w997:bool)  [unwired: 2 out]
                n404 = Compound Arithmetic op=OR(w995, w994, w997) -> (w998:bool)
                n405 = Select(t=T10."Stop", s=w998, f=T10."BurnIn") -> (s? t:f=w1035:T10)
              }
              frame "MotorSpeed" {
                n406 = control-ref of="Motor Speed RPM"() -> (w1044:refnum<vi>)
                n407 = Equal?(x=w1041, y=u8 95) -> (x = y?=w1042:bool)
                n408 = call "Find_Number_LineMARVIN.vi"("Test Paragraph"="Fan speed", "TableIn"=w1046) -> ("error out"=w1058:errorcluster, "Line number"=w1049:i32)  [unwired: 3 in, 2 out]
                n409 = property class="DigNum (strict)"(reference=w1044, error in=w1058) -> (error out=w1047:errorcluster, "Value"=w1048:dbl)  [unwired: 1 out]
                n410 = Select(t=14700.0 ("y"), s=w1042, f=12100.0 ("y")) -> (s? t:f=w1045:dbl)
                n411 = Select(t=200.0 ("y"), s=w1042, f=200.0) -> (s? t:f=w1050:dbl)
                n412 = Add(x=w1045, y=w1050) -> (x+y=w1057:dbl)
                n413 = Subtract(x=w1045, y=w1050) -> (x-y=w1056:dbl)
                n414 = In Range and Coerce(upper limit=w1057, x=w1048, lower limit=w1056) -> (In Range?=w1040:bool)  [unwired: 1 out]
                "BurnSpeed" <- w1040
                n415 = call "PassOrFail (SubVI).vi"("index (row)"=w1049, "error in (no error)"=w1047, "Data in"=w1048, "Pass?Fail"=w1040, "Table in"=w1046) -> ("error out"=w1043:errorcluster)  [unwired: 6 in]
                n416 = property class="Bool (strict)"(reference=w1061, error in=w1043) -> ("Value"=w1065:bool)  [unwired: 2 out]
                n417 = Select(t=T10."Stop", s=w1065, f=T10."Ambient Temp") -> (s? t:f=w1062:T10)
                n418 = Not(x=w1040) -> (.not. x?=w1039:bool)
              }
              frame "DC Current Measure" {
                n419 = call "GetADCTester (SubVI).vi"("GetADCTester"=T8."Current", "TimeToGet"=10) -> ("error out"=w1087:errorcluster, "ADCValOutput Single"=w1074:dbl)  [unwired: 7 in, 1 out]
                n420 = Equal?(x=w1070, y=u8 95) -> (x = y?=w1071:bool)
                n421 = call "Find_Number_LineMARVIN.vi"("Test Paragraph"="DC Input Current", "error in"=w1087, "TableIn"=w1075) -> ("error out"=w1086:errorcluster, "Line number"=w1076:i32)  [unwired: 2 in, 2 out]
                n422 = Select(t=45.0 ("y"), s=w1071, f=28.0 ("y")) -> (s? t:f=w1078:dbl)
                n423 = Select(t=5.0 ("y"), s=w1071, f=3.0) -> (s? t:f=w1077:dbl)
                n424 = Add(x=w1078, y=w1077) -> (x+y=w1085:dbl)
                n425 = Subtract(x=w1078, y=w1077) -> (x-y=w1084:dbl)
                n426 = In Range and Coerce(upper limit=w1085, x=w1074, lower limit=w1084) -> (In Range?=w1069:bool)  [unwired: 1 out]
                "BurnDC" <- w1069
                n427 = call "PassOrFail (SubVI).vi"("index (row)"=w1076, "error in (no error)"=w1086, "Data in"=w1074, "Pass?Fail"=w1069, "Table in"=w1075) -> ("error out"=w1073:errorcluster)  [unwired: 6 in]
                n428 = property class="Bool (strict)"(reference=w1091, error in=w1073) -> ("Value"=w1068:bool)  [unwired: 2 out]
                n429 = Not(x=w1069) -> (.not. x?=w1067:bool)
                n430 = Select(t=T10."Stop", s=w1068, f=T10."MotorSpeed") -> (s? t:f=w1092:T10)
              }
              frame "Start" {
                w1095 = "Burn-in Test" ("Line to focus")
                (unwired) TRUE ("Remote")
                w1097 = "Burn-in test in process...\nFull Speed Operation" ("Value")
                n431 = Equal?(x=w1099, y=u8 95) -> (x = y?=w1100:bool)
                n432 = property class="Str"(reference=w1117, "Value"=w1097) -> (reference out=w1115:refnum<vi>, error out=w1101:errorcluster)  [unwired: 1 in]
                n433 = call "Find_Number_LineMARVIN.vi"("Test Paragraph"=w1095, "error in"=w1101, "TableIn"=w1105) -> ("error out"=w1123:errorcluster, "Line number"=w1124:i32)  [unwired: 2 in, 2 out]
                n434 = Select(t=u16 14700 ("y"), s=w1100, f=u16 12100 ("y")) -> ()  [unwired: 1 out]
                n435 = call "Table_ScrollaBarMarvin.vi"("error in"=w1123, "Line to focus"=w1095, "reference in"=w1105) -> ("error out"=w1125:errorcluster)  [unwired: 2 out]
                n436 = call "Reset old test Values (SubVI).vi"("error in"=w1125, "Atr in"=w1105, "Test Paragraph"=w1095) -> ()  [unwired: 8 in, 1 out]
                n437 = Increment(x=w1124) -> (x+1=w1118:i32)
                n438 = call "TesterOption (SubVI).vi"("2 Options"=FALSE, "On/Off"=TRUE, "Tester Option"=T6."Venable") -> ("error out"=w1126:errorcluster)  [unwired: 7 in, 1 out]
                n439 = call "CANSendMessage.vi"("error in (no error)"=w1126) -> ("error out"=w1116:errorcluster)  [unwired: 10 in]
                n440 = control-ref of="Motor Speed RPM"() -> (w1104:refnum<vi>)
                n441 = call "Write panel message Kinetics (SubVI).vi"(4:"rpm"=w1104, 5:"rpm"=TRUE ("rpm"), "PrintTime"=TRUE, "Stop"=w1111, "error in (no error)"=w1116, "Time to wait"=50.0, "Strin"=w1097, "String in"=w1115) -> ("error out"=w1103:errorcluster)  [unwired: 3 in]
                n442 = property class="Bool (strict)"(reference=w1111, error in=w1103) -> ("Value"=w1110:bool)  [unwired: 2 out]
                n443 = Select(t=T10."Stop", s=w1110, f=T10."DC Current Measure") -> (s? t:f=w1107:T10)
              }
            }
          }
        }
        frame "Visual Inspec" {
          n444 = control-ref of="Stop Button"() -> (w1130:refnum<vi>)
          n445 = property class="Bool (strict)"(reference=w1130, error in=w1129) -> (error out=w1128:errorcluster, "Value"=w1127:bool)  [unwired: 1 out]
          n446 = case shown="False" w1127 {
            tunnel: w1131 -> [w1144 _]
            tunnel: w1128 -> [w1132 _]
            frame False {
              n447 = call "TesterOption (SubVI).vi"("2 Options"=FALSE, "error in (no error)"=w1132, "On/Off"=FALSE, "Tester Option"=T6."Venable") -> ("error out"=w1140:errorcluster)  [unwired: 6 in, 1 out]
              n448 = local read "UUT"() -> (w1136:u8)
              n449 = Equal?(x=w1136, y=u8 95) -> (x = y?=w1137:bool)
              n450 = case shown="True" w1137 {
                tunnel: w1144 -> [w1148 w1158]
                tunnel: w1140 -> [w1147 w1157]
                tunnel: [w1149 w1160] -> w1139
                tunnel: [w1150 w1159] -> w1135
                tunnel: string[] ["Verification of Components Not Installed", "Manufacturing Defects", "DC Input Current Drawn", "12V", "5V", "3.3V", "1.8V", "Reverse Polarity Test - DC Input Current", "Weight Check", "J3.B to Chassis", "J1.16 to Chassis", "J1 Body to Chassis", "J2  Body to Chassis", "J3  Body to Chassis", "J1.17 to J1.18", "Sealing Test", "Mounting Holes Test - Jig Fit"] ("deleted portion 3") -> [w1145 w1155]
                frame False {
                  # "AHU"
                  n451 = for {
                    tunnel: w1145 -> [w1154] mode=indexing
                    tunnel: w1148 -> [w1153]
                    tunnel: w1147 -> [w1152]
                    tunnel: [w1151] -> w1146
                    n452 = call "Reset old test Values (SubVI).vi"("error in"=w1152, "Atr in"=w1153, "Test Paragraph"=w1154) -> ("error out"=w1151:errorcluster)  [unwired: 8 in]
                  }
                  n453 = call "VisualInspectionAHUold.vi"("error in (no error)"=w1146, "TableRef"=w1148) -> ("error out"=w1150:errorcluster, "VisualInspectionResult"=w1149:bool)  [unwired: 8 in]
                }
                frame True {
                  # "EBAY"
                  n454 = for {
                    tunnel: w1158 -> [w1164]
                    tunnel: w1157 -> [w1163]
                    tunnel: [w1162] -> w1156
                    tunnel: w1155 -> [w1161] mode=indexing
                    n455 = call "Reset old test Values (SubVI).vi"("error in"=w1163, "Atr in"=w1164, "Test Paragraph"=w1161) -> ("error out"=w1162:errorcluster)  [unwired: 8 in]
                  }
                  n456 = call "VisualInspectionEBAYold.vi"("error in (no error)"=w1156, "TableRef"=w1158) -> ("error out"=w1159:errorcluster, "VisualInspectionResult"=w1160:bool)  [unwired: 8 in]
                }
              }
              "VisualInspectionResult" <- w1139
              n457 = property on="Automation" class="Bool (strict)"(error in=w1135) -> ("Value"=w1134:bool)  [unwired: 1 in, 2 out]
              n458 = case shown="True" w1134 {
                frame False {
                }
                frame True {
                  w1165 = TRUE ("Value (Signaling)")
                  n459 = property on="SetSN" class="Bool (strict)"("Val(Sgnl)"=w1165, "Value"=w1165) -> ()  [unwired: 2 in, 2 out]
                }
              }
            }
            frame True {
            }
          }
        }
        frame "Temp Sens Cal" {
          w1169 = "Temperature sensor calibration test in process..." ("Value")
          w1167 = "Temperature Sensor Calibration" ("Test Paragraph")
          n460 = control-ref of="Pannel User Message"() -> (w1176:refnum<vi>)
          n461 = property class="Str"(reference=w1176, error in=w1175, "Value"=w1169) -> (error out=w1174:errorcluster)  [unwired: 1 out]
          n462 = call "Table_ScrollaBarMarvin.vi"("error in"=w1174, "Line to focus"=w1167, "reference in"=w1177) -> ("error out"=w1179:errorcluster)  [unwired: 2 out]
          n463 = property class="Tbl (strict)"(reference=w1177, error in=w1179) -> (reference out=w1166:refnum<vi>, error out=w1181:errorcluster, "Value"=w1182:string[][])
          n464 = Index Array(array=w1182, index (col)=1 ("disabled index (col)")) -> (element=w1183:string[])  [unwired: 1 in]
          n465 = call "Find_Number_Line.vi"("error in"=w1181, "Test Paragraph"=w1167, "Row Headers[]"=w1183) -> ("error out"=w1178:errorcluster, "Line number"=w1171:i32)  [unwired: 1 out]
          n466 = property on="Status" class="Bool (strict)"(error in=w1178) -> (error out=w1172:errorcluster, "Value"=w1173:bool)  [unwired: 1 in, 1 out]
          n467 = call "Reset old test Values (SubVI).vi"("error in"=w1172, "Atr in"=w1166, "Test Paragraph"=w1167) -> ("error out"=w1168:errorcluster)  [unwired: 8 in]
          n468 = case shown="True" w1173 {
            selector: w1173 -> [w1187 _]
            tunnel: w1168 -> [w1189 _]
            tunnel: w1166 -> [w1186 _]
            tunnel: w1171 -> [w1185 _]
            tunnel: w1170 -> [_ w1194]
            tunnel: w1169 -> [_ w1192]
            frame False {
              n469 = flat-sequence {
                tunnel: w1189 -> [w1190]
                tunnel: [w1190] -> w1188
                frame #0 {
                  n470 = One Button Dialog(message="Please establish RS connection.") -> ()  [unwired: 1 in, 1 out]
                }
              }
              n471 = Increment(x=w1185) -> (x+1=w1184:i32)
              n472 = call "PassOrFail (SubVI).vi"("index (row)"=w1184, "error in (no error)"=w1188, "Pass?Fail"=w1187, "Table in"=w1186) -> ()  [unwired: 7 in, 1 out]
            }
            frame True {
              n473 = control-ref of="Pannel User Message"() -> (w1197:refnum<vi>)
              n474 = control-ref of="ATR"() -> (w1198:refnum<vi>)
              n475 = control-ref of="Motor Speed RPM"() -> (w1199:refnum<vi>)
              n476 = control-ref of="UUT"() -> (w1193:refnum<vi>)
              n477 = control-ref of="Stop Button"() -> (w1196:refnum<vi>)
              n478 = while {
                shift-right: [w1202] -> _
                shift-left: T9."Start" -> [w1209]
                tunnel: w1196 -> [w1208]
                tunnel: w1197 -> [w1207]
                tunnel: w1198 -> [w1206]
                tunnel: w1199 -> [w1205]
                tunnel: w1194 -> [w1204]
                tunnel: w1193 -> [w1203]
                tunnel: w1192 -> [w1200]
                stop <- w1201 stop-if-true
                n479 = case shown="\"Stop\", Default" w1209 {
                  tunnel: w1208 -> [_ w1242 w1259 w1302 w1344]
                  tunnel: w1207 -> [_ w1240 w1267 w1314 w1346]
                  tunnel: w1206 -> [_ w1220 _ _ _]
                  tunnel: w1205 -> [_ w1243 w1266 w1316 w1342]
                  tunnel: w1204 -> [_ w1251 w1269 w1324 w1339]
                  tunnel: w1203 -> [_ _ _ _ _]
                  tunnel: [w1210 w1229 w1260 w1305 w1330] -> w1202
                  tunnel: [w1211 FALSE FALSE FALSE FALSE] -> w1201
                  tunnel: w1200 -> [_ _ w1268 _ _]
                  frame "Stop", Default {
                    n480 = flat-sequence {
                      tunnel: [TRUE] -> w1211
                      tunnel: [T9."Stop"] -> w1210
                      frame #0 {
                        n481 = call "TesterOption (SubVI).vi"("2 Options"=FALSE, "On/Off"=FALSE, "Tester Option"=T6."Venable") -> ()  [unwired: 7 in, 2 out]
                      }
                      frame #1 {
                      }
                    }
                  }
                  frame "AO[1]=Meas." {
                    n482 = property on="AO[1]Meas" class="DigNum (strict)"() -> ("Value"=w1223:dbl)  [unwired: 2 in, 2 out]
                    n483 = Number To Fractional String(number=w1223) -> (F-format string=w1231:string)  [unwired: 3 in]
                    n484 = Search and Replace String(input string="EP=1\r\nAO[1]=0\r\n" ("write buffer"), search string="0", replace string=w1231) -> (result string=w1230:string)  [unwired: 5 in, 3 out]
                    n485 = call "SerialMarvinSendGet.vi"("Clear Log"=FALSE, "write buffer"=w1230, "VISA resource name"=w1251) -> ("error out"=w1247:errorcluster)  [unwired: 7 in, 1 out]
                    n486 = call "TesterOption (SubVI).vi"("2 Options"=FALSE, "error in (no error)"=w1247, "On/Off"=FALSE, "Tester Option"=T6."Power") -> ("error out"=w1246:errorcluster, "VISA Refnum out"=w1234:refnum<visa-resource-name>)  [unwired: 6 in]
                    n487 = call "Write panel message Kinetics (SubVI).vi"(4:"rpm"=w1243, 5:"rpm"=FALSE ("rpm"), "PrintTime"=TRUE, "Stop"=w1242, "error in (no error)"=w1246, "Time to wait"=20.0, "Strin"="Temperature sensor calibration test in process...\nSet Parameters...", "String in"=w1240) -> ("error out"=w1235:errorcluster)  [unwired: 3 in]
                    n488 = call "TesterOption (SubVI).vi"("2 Options"=FALSE, "error in (no error)"=w1235, "On/Off"=FALSE, "Tester Option"=T6."Venable", "VISA Refnum in"=w1234) -> ("error out"=w1228:errorcluster)  [unwired: 5 in, 1 out]
                    n489 = flat-sequence {
                      tunnel: [T9."Stop"] -> w1229
                      tunnel: w1221 -> [_]
                      frame #0 {
                      }
                    }
                    n490 = In Range and Coerce(upper limit=0.1, x=w1223, lower limit=-0.1) -> (In Range?=w1218:bool)  [unwired: 1 out]
                    "SensCalResult" <- w1218
                    n491 = call "Find_Number_LineMARVIN.vi"("Test Paragraph"="Sensor Reading Analog Offset", "error in"=w1228, "TableIn"=w1220) -> ("error out"=w1222:errorcluster, "Line number"=w1226:i32)  [unwired: 2 in, 2 out]
                    n492 = call "PassOrFail (SubVI).vi"("Test#"="2", "index (row)"=w1226, "error in (no error)"=w1222, "Data in"=w1223, "Pass?Fail"=w1218, "Table in"=w1220) -> ("error out"=w1221:errorcluster)  [unwired: 5 in]
                  }
                  frame "TA[5]" {
                    w1270 = T12 [enum."50C", enum."80C", enum."100C", enum."120C"] items=["K15", "K16", "K17", "Venable", "Firmeware", "Fan", "Power", "120C", "110C", "100C", "90C", "80C", "70C", "60C", "50C", "40C", "30C", "25C", "20C", "10C", "0C"]
                    n493 = for {
                      tunnel: w1270 -> [w1283] mode=indexing
                      tunnel: w1269 -> [w1282]
                      tunnel: w1268 -> [w1281]
                      tunnel: w1267 -> [w1280]
                      tunnel: w1259 -> [w1279]
                      tunnel: w1266 -> [w1278]
                      tunnel: dbl[] [0.59774, 0.65238, 0.68545, 0.71584] -> [w1273] mode=indexing
                      tunnel: [w1272] -> w1255 mode=indexing
                      tunnel: [w1271] -> w1258
                      n494 = for {
                        N: 5 -> [_]
                        tunnel: w1283 -> [w1299]
                        tunnel: w1282 -> [w1298]
                        tunnel: w1281 -> [w1293]
                        tunnel: w1280 -> [w1292]
                        tunnel: w1279 -> [w1291]
                        tunnel: w1278 -> [w1287]
                        tunnel: [w1286] -> w1277 mode=indexing
                        tunnel: [w1285] -> w1271
                        n495 = call "TesterOption (SubVI).vi"("2 Options"=FALSE, "On/Off"=TRUE, "Tester Option"=w1299) -> ("error out"=w1295:errorcluster)  [unwired: 7 in, 1 out]
                        n496 = call "Write panel message Kinetics (SubVI).vi"(4:"rpm"=w1287, 5:"rpm"=FALSE ("rpm"), "PrintTime"=FALSE, "Stop"=w1291, "error in (no error)"=w1295, "Time to wait"=1.0, "Strin"=w1293, "String in"=w1292) -> ("error out"=w1294:errorcluster)  [unwired: 3 in]
                        n497 = call "SerialMarvinSendGet.vi"("error in (no error)"=w1294, "write buffer"="TA[5]\r\n", "VISA resource name"=w1298) -> ("error out"=w1285:errorcluster, "read buffer"=w1296:string)  [unwired: 7 in]
                        n498 = Fract/Exp String To Number(string=w1296) -> (number=w1286:dbl)  [unwired: 3 in, 1 out]
                      }
                      n499 = Add Array Elements(numeric array=w1277) -> (sum=w1276:dbl)
                      n500 = Divide(x=w1276, y=5.0) -> (x/y=w1274:dbl)
                      n501 = Subtract(x=w1274, y=w1273) -> (x-y=w1272:dbl)
                    }
                    n502 = property class="Bool (strict)"(reference=w1259, error in=w1258) -> ("Value"=w1264:bool)  [unwired: 2 out]
                    n503 = Select(t=T9."Stop", s=w1264, f=T9."AO[1]=Meas.") -> (s? t:f=w1260:T9)
                    n504 = Array Size(array=w1255) -> (size(s)=w1254:i32)
                    n505 = Add Array Elements(numeric array=w1255) -> (sum=w1257:dbl)
                    n506 = Divide(x=w1257, y=w1254) -> (x/y=→"AO[1]Meas":dbl)
                  }
                  frame "AO[1]=0" {
                    n507 = call "SerialMarvinSendGet.vi"("write buffer"="EP=1\r\nAO[1]=0\r\n", "VISA resource name"=w1324) -> ("error out"=w1320:errorcluster)  [unwired: 8 in, 1 out]
                    n508 = call "TesterOption (SubVI).vi"("2 Options"=FALSE, "error in (no error)"=w1320, "On/Off"=FALSE, "Tester Option"=T6."Power") -> ("error out"=w1319:errorcluster, "VISA Refnum out"=w1308:refnum<visa-resource-name>)  [unwired: 6 in]
                    n509 = call "Write panel message Kinetics (SubVI).vi"(4:"rpm"=w1316, 5:"rpm"=FALSE ("rpm"), "PrintTime"=TRUE, "Stop"=w1302, "error in (no error)"=w1319, "Time to wait"=20.0, "Strin"="Temperature sensor calibration test in process...\nSet Parameters...", "String in"=w1314) -> ("error out"=w1309:errorcluster)  [unwired: 3 in]
                    n510 = call "TesterOption (SubVI).vi"("2 Options"=FALSE, "error in (no error)"=w1309, "On/Off"=FALSE, "Tester Option"=T6."Venable", "VISA Refnum in"=w1308) -> ("error out"=w1303:errorcluster)  [unwired: 5 in, 1 out]
                    n511 = property class="Bool (strict)"(reference=w1302, error in=w1303) -> ("Value"=w1307:bool)  [unwired: 2 out]
                    n512 = Select(t=T9."Stop", s=w1307, f=T9."TA[5]") -> (s? t:f=w1305:T9)
                  }
                  frame "Start" {
                    (unwired) TRUE ("Remote")
                    (unwired) u16 0 ("Motor Speed RPM")
                    n513 = call "Write panel message Kinetics (SubVI).vi"(4:"rpm"=w1342, 5:"rpm"=FALSE ("rpm"), "PrintTime"=FALSE, "Stop"=w1344, "Time to wait"=0.1, "Strin"="Temperature sensor calibration test in process...\nInitialization state...", "String in"=w1346) -> ("error out"=w1347:errorcluster)  [unwired: 4 in]
                    n514 = call "TesterOption (SubVI).vi"("2 Options"=FALSE, "error in (no error)"=w1347, "On/Off"=FALSE, "Tester Option"=T6."Venable") -> ("error out"=w1348:errorcluster)  [unwired: 6 in, 1 out]
                    n515 = call "CANSendMessage.vi"("error in (no error)"=w1348) -> ("error out"=w1337:errorcluster)  [unwired: 10 in]
                    n516 = call "SerialMarvinSendGet.vi"("error in (no error)"=w1337, "write buffer"="AO[1]\r\n", "VISA resource name"=w1339) -> ("error out"=w1327:errorcluster, "read buffer"=w1336:string)  [unwired: 7 in]
                    n517 = Equal?(x=w1336, y="0.0") -> (x = y?=w1328:bool)
                    n518 = property class="Bool (strict)"(reference=w1344, error in=w1327) -> ("Value"=w1352:bool)  [unwired: 2 out]
                    n519 = Select(t=T9."TA[5]", s=w1328, f=T9."AO[1]=0") -> (s? t:f=w1332:T9)
                    n520 = Select(t=T9."Stop", s=w1352, f=w1332) -> (s? t:f=w1330:T9)
                  }
                }
              }
            }
          }
        }
        frame "Auxiliary" {
          w1356 = "Auxiliary test in process..." ("Value")
          w1367 = "Auxiliary Fan Test" ("Test Paragraph")
          n521 = control-ref of="Pannel User Message"() -> (w1366:refnum<vi>)
          n522 = property class="Str"(reference=w1366, error in=w1363, "Value"=w1356) -> (error out=w1365:errorcluster)  [unwired: 1 out]
          n523 = call "Table_ScrollaBarMarvin.vi"("error in"=w1365, "Line to focus"=w1367, "reference in"=w1364) -> ("error out"=w1373:errorcluster)  [unwired: 2 out]
          n524 = property class="Tbl (strict)"(reference=w1364, error in=w1373) -> (reference out=w1362:refnum<vi>, error out=w1372:errorcluster, "Value"=w1371:string[][])
          n525 = Index Array(array=w1371, index (col)=1 ("disabled index (col)")) -> (element=w1370:string[])  [unwired: 1 in]
          n526 = call "Find_Number_Line.vi"("error in"=w1372, "Test Paragraph"=w1367, "Row Headers[]"=w1370) -> ("error out"=w1368:errorcluster, "Line number"=w1355:i32)  [unwired: 1 out]
          n527 = call "Reset old test Values (SubVI).vi"("error in"=w1368, "Atr in"=w1362, "Test Paragraph"=w1367) -> ("error out"=w1360:errorcluster)  [unwired: 8 in]
          n528 = control-ref of="Stop Button"() -> (w1358:refnum<vi>)
          n529 = control-ref of="Pannel User Message"() -> (w1359:refnum<vi>)
          n530 = control-ref of="ATR"() -> (w1354:refnum<vi>)
          n531 = control-ref of="Motor Speed RPM"() -> (w1357:refnum<vi>)
          n532 = while {
            shift-right: [w1379] -> _
            shift-left: enum16{"Stop", "CoolingON", "HotGunON", "Start"}."Start" -> [w1384]
            tunnel: w1360 -> [w1377]
            tunnel: w1359 -> [w1383]
            tunnel: w1358 -> [w1382]
            tunnel: w1357 -> [w1381]
            tunnel: w1356 -> [w1380]
            tunnel: w1355 -> [w1376]
            tunnel: w1354 -> [w1375]
            tunnel: w1353 -> [w1374]
            stop <- w1378 stop-if-true
            n533 = case shown="\"HotGunON\"" w1384 {
              tunnel: w1383 -> [_ w1427 w1516 w1564]
              tunnel: w1382 -> [_ w1423 w1512 w1563]
              tunnel: w1381 -> [_ w1426 w1515 w1561]
              tunnel: w1380 -> [_ w1418 w1507 w1562]
              tunnel: [w1386 w1420 w1509 w1555] -> w1379
              tunnel: [w1385 FALSE FALSE FALSE] -> w1378
              tunnel: w1377 -> [_ w1417 w1506 _]
              tunnel: w1376 -> [_ w1412 w1501 w1556]
              tunnel: w1375 -> [_ w1408 w1498 w1558]
              tunnel: w1374 -> [_ _ _ w1565]
              frame "Stop", Default {
                n534 = flat-sequence {
                  tunnel: [enum16{"Stop", "CoolingON", "HotGunON", "Start"}."Stop"] -> w1386
                  tunnel: [TRUE] -> w1385
                  frame #0 {
                    n535 = call "TesterOption (SubVI).vi"("2 Options"=FALSE, "On/Off"=FALSE, "Tester Option"=T6."Venable") -> ()  [unwired: 7 in, 2 out]
                  }
                  frame #1 {
                  }
                }
              }
              frame "CoolingON" {
                n536 = while {
                  tunnel: w1427 -> [w1460]
                  tunnel: w1426 -> [w1456]
                  tunnel: [w1453] -> w1397
                  tunnel: w1423 -> [w1444]
                  tunnel: w1418 -> [w1448]
                  tunnel: w1417 -> [w1445]
                  shift-right: [w1437] -> w1392
                  shift-left: 0.0 -> [w1438]
                  shift-right: [w1433] -> w1396
                  shift-left: 0.0 ("Value") -> [w1435]
                  tunnel: [w1429] -> w1400
                  stop <- w1442 stop-if-true
                  n537 = control-ref of="Power transistor Heat sink Temp."() -> (w1454:refnum<vi>)
                  n538 = property class="DigNum (strict)"(reference=w1454, error in=w1445) -> (error out=w1451:errorcluster, "Value"=w1433:dbl)  [unwired: 1 out]
                  n539 = Equal?(x=w1433, y=w1435) -> (x = y?=w1434:bool)
                  n540 = Number To Fractional String(number=w1433, precision (6)=i16 2) -> (F-format string=w1447:string)  [unwired: 2 in]
                  n541 = case shown="True" w1434 {
                    tunnel: w1438 -> [_ w1478]
                    tunnel: [0.0 w1476] -> w1437
                    tunnel: [FALSE w1475] -> w1436
                    frame False {
                    }
                    frame True {
                      n542 = Increment(x=w1478) -> (x+1=w1476:dbl)
                      n543 = Greater Or Equal?(x=w1476, y=300.0) -> (x >= y?=w1475:bool)
                    }
                  }
                  n544 = Concatenate Strings(w1448, "\nPCB Temperature [C]: " ("string"), w1447) -> (w1446:string)
                  n545 = call "Write panel message Kinetics (SubVI).vi"(4:"rpm"=w1456, 5:"rpm"=FALSE ("rpm"), "PrintTime"=FALSE, "Stop"=w1444, "error in (no error)"=w1451, "Time to wait"=0.2, "Strin"=w1446, "String in"=w1460) -> ("error out"=w1450:errorcluster)  [unwired: 3 in]
                  n546 = property class="Bool (strict)"(reference=w1444) -> ("Value"=w1443:bool)  [unwired: 1 in, 2 out]
                  n547 = Less Or Equal?(x=w1433, y=52.0) -> (x <= y?=w1432:bool)
                  n548 = call "GetADCTester (SubVI).vi"("error in (no error)"=w1450, "GetADCTester"=T8."Fan") -> ("error out"=w1453:errorcluster, "ADCValOutput Single"=w1440:dbl)  [unwired: 7 in, 1 out]
                  n549 = Greater?(x=w1440, y=u32 2400) -> (0:w1430:bool)
                  n550 = case shown="True" w1432 {
                    tunnel: [w1466 w1472] -> w1431
                    tunnel: w1432 -> [w1466 w1472]
                    tunnel: [w1461 w1467] -> w1429
                    frame False {
                      n551 = call "Time Delay11"() -> ("error out"=w1464:errorcluster)  [unwired: 11 in]
                      n552 = call "GetADCTester (SubVI).vi"("error in (no error)"=w1464, "GetADCTester"=T8."Fan") -> ("ADCValOutput Single"=w1463:dbl)  [unwired: 7 in, 2 out]
                      n553 = Greater?(x=w1463, y=2400.0) -> (0:w1461:bool)
                    }
                    frame True {
                      n554 = call "Time Delay10"() -> ("error out"=w1470:errorcluster)  [unwired: 11 in]
                      n555 = call "GetADCTester (SubVI).vi"("error in (no error)"=w1470, "GetADCTester"=T8."Fan") -> ("ADCValOutput Single"=w1469:dbl)  [unwired: 7 in, 2 out]
                      n556 = Greater?(x=w1469, y=2400.0) -> (0:w1467:bool)
                    }
                  }
                  n557 = Compound Arithmetic op=OR(w1430, w1443, w1431, w1436) -> (w1442:bool)
                }
                "Numeric" <- w1392
                n558 = In Range and Coerce(upper limit=58.0, x=w1396, lower limit=52.0) -> (In Range?=w1399:bool)  [unwired: 1 out]
                n559 = Build Array(w1400, w1399) -> (w1401:bool[])
                n560 = And Array Elements(Boolean array=w1401) -> (logical AND=→"AuxiOFFResult":bool)
                n561 = Add(x=w1412, y=3) -> (x+y=w1410:i32)
                n562 = call "PassOrFail (SubVI).vi"("index (row)"=w1410, "error in (no error)"=w1397, "Data in"=w1396, "Pass?Fail"=w1399, "Table in"=w1408) -> ("error out"=w1414:errorcluster)  [unwired: 6 in]
                n563 = Select(t="OFF", s=w1400, f="ON") -> (s? t:f=w1404:string)
                n564 = Increment(x=w1410) -> (x+1=w1409:i32)
                n565 = call "PassOrFail (SubVI).vi"("String Res"=w1404, "index (row)"=w1409, "error in (no error)"=w1414, "Data in"=-3.0, "Pass?Fail"=w1400, "Table in"=w1408) -> ("error out"=w1413:errorcluster)  [unwired: 5 in]
                n566 = call "TesterOption (SubVI).vi"("2 Options"=FALSE, "error in (no error)"=w1413, "On/Off"=FALSE, "Tester Option"=T6."Venable" ("Tester Option 2")) -> ("error out"=w1394:errorcluster)  [unwired: 6 in, 1 out]
                n567 = call "Time Delay14"("error in (no error)"=w1394) -> ("error out"=w1393:errorcluster)  [unwired: 10 in]
                n568 = property class="Bool (strict)"(reference=w1423, error in=w1393) -> ("Value"=w1428:bool)  [unwired: 2 out]
                n569 = Select(t=enum16{"Stop", "CoolingON", "HotGunON", "Start"}."Stop", s=w1428, f=enum16{"Stop", "CoolingON", "HotGunON", "Start"}."Stop") -> (s? t:f=w1420:enum16{"Stop", "CoolingON", "HotGunON", "Start"})
              }
              frame "HotGunON" {
                n570 = while {
                  tunnel: w1516 -> [w1547]
                  tunnel: w1515 -> [w1543]
                  tunnel: [w1540] -> w1488
                  tunnel: w1512 -> [w1531]
                  tunnel: w1507 -> [w1535]
                  tunnel: w1506 -> [w1532]
                  shift-right: [w1524] -> _
                  shift-left: 0.0 -> [w1525]
                  shift-right: [w1521] -> _
                  shift-left: 0.0 ("Value") -> [w1522]
                  tunnel: [w1519] -> w1486
                  stop <- w1529 stop-if-true
                  n571 = control-ref of="Power transistor Heat sink Temp."() -> (w1541:refnum<vi>)
                  n572 = property class="DigNum (strict)"(reference=w1541, error in=w1532) -> (error out=w1538:errorcluster, "Value"=w1521:dbl)  [unwired: 1 out]
                  n573 = Equal?(x=w1521, y=w1522) -> (x = y?=w1520:bool)
                  n574 = Number To Fractional String(number=w1521, precision (6)=i16 2) -> (F-format string=w1534:string)  [unwired: 2 in]
                  n575 = case shown="True" w1520 {
                    tunnel: w1525 -> [_ w1553]
                    tunnel: [0.0 w1551] -> w1524
                    tunnel: [FALSE w1550] -> w1523
                    frame False {
                    }
                    frame True {
                      n576 = Increment(x=w1553) -> (x+1=w1551:dbl)
                      n577 = Greater Or Equal?(x=w1551, y=300.0) -> (x >= y?=w1550:bool)
                    }
                  }
                  n578 = Concatenate Strings(w1535, "\nPCB Temperature [C]: " ("string"), w1534) -> (w1533:string)
                  n579 = call "Write panel message Kinetics (SubVI).vi"(4:"rpm"=w1543, 5:"rpm"=FALSE ("rpm"), "PrintTime"=FALSE, "Stop"=w1531, "error in (no error)"=w1538, "Time to wait"=0.2, "Strin"=w1533, "String in"=w1547) -> ("error out"=w1537:errorcluster)  [unwired: 3 in]
                  n580 = property class="Bool (strict)"(reference=w1531) -> ("Value"=w1530:bool)  [unwired: 1 in, 2 out]
                  n581 = call "GetADCTester (SubVI).vi"("error in (no error)"=w1537, "GetADCTester"=T8."Fan") -> ("error out"=w1540:errorcluster, "ADCValOutput Single"=w1527:dbl)  [unwired: 7 in, 1 out]
                  n582 = Greater Or Equal?(x=w1521, y=61.0) -> (x >= y?=w1518:bool)
                  n583 = Less?(x=w1527, y=u32 100) -> (x < y?=w1519:bool)
                  n584 = Compound Arithmetic op=OR(w1519, w1530, w1518, w1523) -> (w1529:bool)
                }
                n585 = control-ref of="Power transistor Heat sink Temp."() -> (w1491:refnum<vi>)
                n586 = property class="DigNum (strict)"(reference=w1491, error in=w1488) -> (error out=w1490:errorcluster, "Value"=w1489:dbl)  [unwired: 1 out]
                n587 = In Range and Coerce(upper limit=62.0, x=w1489, lower limit=58.0) -> (In Range?=w1485:bool)  [unwired: 1 out]
                n588 = Build Array(w1486, w1485) -> (w1487:bool[])
                n589 = Increment(x=w1501) -> (x+1=w1500:i32)
                n590 = call "PassOrFail (SubVI).vi"("index (row)"=w1500, "error in (no error)"=w1490, "Data in"=w1489, "Pass?Fail"=w1485, "Table in"=w1498) -> ("error out"=w1503:errorcluster)  [unwired: 6 in]
                n591 = And Array Elements(Boolean array=w1487) -> (logical AND=→"AuxiONResult":bool)
                n592 = Increment(x=w1500) -> (x+1=w1499:i32)
                n593 = Select(t="ON", s=w1486, f="OFF") -> (s? t:f=w1496:string)
                n594 = call "PassOrFail (SubVI).vi"("String Res"=w1496, "index (row)"=w1499, "error in (no error)"=w1503, "Data in"=-3.0, "Pass?Fail"=w1486, "Table in"=w1498) -> ("error out"=w1502:errorcluster)  [unwired: 5 in]
                n595 = call "TesterOption (SubVI).vi"("On/Off 2"=FALSE, "Tester Option 2"=T6."Venable", "2 Options"=TRUE, "error in (no error)"=w1502, "On/Off"=FALSE, "Tester Option"=T6."Fan") -> ("error out"=w1480:errorcluster)  [unwired: 4 in, 1 out]
                n596 = call "Time Delay13"("error in (no error)"=w1480) -> ("error out"=w1479:errorcluster)  [unwired: 10 in]
                n597 = property class="Bool (strict)"(reference=w1512, error in=w1479) -> ("Value"=w1517:bool)  [unwired: 2 out]
                n598 = Select(t=enum16{"Stop", "CoolingON", "HotGunON", "Start"}."Stop", s=w1517, f=enum16{"Stop", "CoolingON", "HotGunON", "Start"}."CoolingON") -> (s? t:f=w1509:enum16{"Stop", "CoolingON", "HotGunON", "Start"})
              }
              frame "Start" {
                n599 = call "Write panel message Kinetics (SubVI).vi"(4:"rpm"=w1561, 5:"rpm"=FALSE ("rpm"), "PrintTime"=FALSE, "Stop"=w1563, "Time to wait"=1.0, "Strin"=w1562, "String in"=w1564) -> ("error out"=w1571:errorcluster)  [unwired: 4 in]
                n600 = call "TesterOption (SubVI).vi"("2 Options"=FALSE, "error in (no error)"=w1571, "On/Off"=FALSE, "Tester Option"=T6."Venable") -> ("error out"=w1566:errorcluster)  [unwired: 6 in, 1 out]
                n601 = while {
                  tunnel: w1566 -> [w1590]
                  tunnel: w1565 -> [w1589]
                  tunnel: w1564 -> [w1588]
                  tunnel: w1563 -> [w1587]
                  tunnel: w1562 -> [w1586]
                  tunnel: w1561 -> [w1585]
                  shift-right: [w1583] -> _
                  shift-left: enum16{"Wait", "OFF", "ON", "Start"}."Start" -> [w1584]
                  shift-right: [w1581] -> _
                  shift-left: 0 -> [w1582]
                  tunnel: w1558 -> [w1579]
                  shift-right: [w1578] -> w1554
                  shift-left: TRUE -> [w1577]
                  tunnel: w1556 -> [w1576]
                  stop <- w1580 stop-if-true
                  n602 = case shown="\"Start\"" w1584 {
                    tunnel: w1590 -> [_ w1635 _ w1695]
                    tunnel: w1589 -> [w1605 w1634 _ w1694]
                    tunnel: w1588 -> [_ w1632 _ w1692]
                    tunnel: w1587 -> [_ w1612 _ w1677]
                    tunnel: w1586 -> [_ w1631 _ w1691]
                    tunnel: w1585 -> [_ w1630 _ w1690]
                    tunnel: [w1608 w1614 enum16{"Wait", "OFF", "ON", "Start"}."OFF" w1674] -> w1583
                    tunnel: w1582 -> [w1609 w1622 _ w1682]
                    tunnel: [w1609 w1621 0 w1681] -> w1581
                    tunnel: [w1607 FALSE FALSE FALSE] -> w1580
                    tunnel: w1579 -> [w1593 _ w1670 _]
                    tunnel: [FALSE w1618 TRUE w1678] -> w1578
                    tunnel: w1577 -> [w1596 _ w1671 _]
                    tunnel: w1576 -> [w1595 _ w1669 _]
                    frame "Wait", Default {
                      n603 = call "SerialMarvinSendGet.vi"("write buffer"="EP=1\r\nAU=0\r\n", "VISA resource name"=w1605) -> ("error out"=w1604:errorcluster)  [unwired: 8 in, 1 out]
                      n604 = call "Time Delay19"("error in (no error)"=w1604) -> ("error out"=w1592:errorcluster)  [unwired: 10 in]
                      n605 = Not(x=w1596) -> (.not. x?=w1598:bool)
                      n606 = Select(t="OFF", s=w1598, f="ON") -> (s? t:f=w1597:string)
                      n607 = Add(x=2, y=w1595) -> (x+y=w1602:i32)
                      n608 = call "PassOrFail (SubVI).vi"("String Res"=w1597, "index (row)"=w1602, "error in (no error)"=w1592, "Data in"=-3.0, "Pass?Fail"=w1598, "Table in"=w1593) -> ("error out"=w1591:errorcluster)  [unwired: 5 in]
                      n609 = flat-sequence {
                        tunnel: [enum16{"Wait", "OFF", "ON", "Start"}."Wait"] -> w1608
                        tunnel: [TRUE] -> w1607
                        tunnel: w1591 -> [_]
                        frame #0 {
                        }
                      }
                    }
                    frame "OFF" {
                      n610 = call "SerialMarvinSendGet.vi"("error in (no error)"=w1635, "write buffer"="EP=1\r\nAU=0\r\n", "VISA resource name"=w1634) -> ("error out"=w1625:errorcluster)  [unwired: 7 in, 1 out]
                      n611 = call "Time Delay"("error in (no error)"=w1625) -> ("error out"=w1620:errorcluster)  [unwired: 10 in]
                      n612 = call "GetADCTester (SubVI).vi"("error in (no error)"=w1620, "GetADCTester"=T8."Fan", "TimeToGet"=5) -> ("error out"=w1624:errorcluster, "ADCValOutput Single"=w1627:dbl)  [unwired: 6 in, 1 out]
                      n613 = Greater?(x=w1627, y=2400.0) -> (0:w1623:bool)
                      n614 = case shown="True" w1623 {
                        tunnel: w1632 -> [_ w1653]
                        tunnel: w1612 -> [_ w1652]
                        tunnel: w1631 -> [_ w1651]
                        tunnel: w1630 -> [_ w1650]
                        tunnel: w1624 -> [w1637 w1649]
                        tunnel: [w1638 w1647] -> w1613
                        tunnel: w1622 -> [w1642 _]
                        tunnel: [w1643 0] -> w1621
                        tunnel: [w1637 w1645] -> w1615
                        tunnel: [w1636 FALSE] -> w1618
                        frame False {
                          n615 = Increment(x=w1642) -> (x+1=w1643:i32)
                          n616 = Greater Or Equal?(x=w1642, y=10) -> (x >= y?=w1636:bool)
                          n617 = Select(t=enum16{"Wait", "OFF", "ON", "Start"}."Wait", s=w1636, f=enum16{"Wait", "OFF", "ON", "Start"}."OFF") -> (s? t:f=w1638:enum16{"Wait", "OFF", "ON", "Start"})
                        }
                        frame True {
                          n618 = call "Write panel message Kinetics (SubVI).vi"(4:"rpm"=w1650, 5:"rpm"=FALSE ("rpm"), "PrintTime"=TRUE, "Stop"=w1652, "error in (no error)"=w1649, "Time to wait"=5.0, "Strin"=w1651, "String in"=w1653) -> ("error out"=w1648:errorcluster)  [unwired: 3 in]
                          n619 = flat-sequence {
                            tunnel: w1648 -> [w1657]
                            tunnel: [enum16{"Wait", "OFF", "ON", "Start"}."Wait"] -> w1647
                            tunnel: [w1657] -> w1645
                            frame #0 {
                            }
                          }
                        }
                      }
                      n620 = property class="Bool (strict)"(reference=w1612, error in=w1615) -> ("Value"=w1617:bool)  [unwired: 2 out]
                      n621 = Select(t=enum16{"Wait", "OFF", "ON", "Start"}."Wait", s=w1617, f=w1613) -> (s? t:f=w1614:enum16{"Wait", "OFF", "ON", "Start"})
                    }
                    frame "ON" {
                      n622 = Not(x=w1671) -> (.not. x?=w1664:bool)
                      n623 = Select(t="ON", s=w1664, f="OFF") -> (s? t:f=w1663:string)
                      n624 = Increment(x=w1669) -> (x+1=w1668:i32)
                      n625 = call "PassOrFail (SubVI).vi"("String Res"=w1663, "index (row)"=w1668, "Data in"=-3.0, "Pass?Fail"=w1664, "Table in"=w1670) -> ()  [unwired: 6 in, 1 out]
                    }
                    frame "Start" {
                      n626 = call "SerialMarvinSendGet.vi"("error in (no error)"=w1695, "write buffer"="EP=1\r\nAU=1\r\n", "VISA resource name"=w1694) -> ("error out"=w1685:errorcluster)  [unwired: 7 in, 1 out]
                      n627 = call "Time Delay18"("error in (no error)"=w1685) -> ("error out"=w1680:errorcluster)  [unwired: 10 in]
                      n628 = call "GetADCTester (SubVI).vi"("error in (no error)"=w1680, "GetADCTester"=T8."Fan", "TimeToGet"=5) -> ("error out"=w1684:errorcluster, "ADCValOutput Single"=w1687:dbl)  [unwired: 6 in, 1 out]
                      n629 = Less?(x=w1687, y=100.0) -> (x < y?=w1683:bool)
                      n630 = case shown="False" w1683 {
                        tunnel: w1692 -> [_ w1713]
                        tunnel: w1677 -> [_ w1712]
                        tunnel: w1691 -> [_ w1711]
                        tunnel: w1690 -> [_ w1710]
                        tunnel: w1684 -> [w1697 w1709]
                        tunnel: [w1698 w1707] -> w1675
                        tunnel: w1682 -> [w1702 _]
                        tunnel: [w1703 0] -> w1681
                        tunnel: [w1697 w1705] -> w1672
                        tunnel: [w1696 FALSE] -> w1678
                        frame False {
                          n631 = Increment(x=w1702) -> (x+1=w1703:i32)
                          n632 = Greater Or Equal?(x=w1702, y=5) -> (x >= y?=w1696:bool)
                          n633 = Select(t=enum16{"Wait", "OFF", "ON", "Start"}."ON", s=w1696, f=enum16{"Wait", "OFF", "ON", "Start"}."Start") -> (s? t:f=w1698:enum16{"Wait", "OFF", "ON", "Start"})
                        }
                        frame True {
                          n634 = call "Write panel message Kinetics (SubVI).vi"(4:"rpm"=w1710, 5:"rpm"=FALSE ("rpm"), "PrintTime"=TRUE, "Stop"=w1712, "error in (no error)"=w1709, "Time to wait"=60.0, "Strin"=w1711, "String in"=w1713) -> ("error out"=w1708:errorcluster)  [unwired: 3 in]
                          n635 = flat-sequence {
                            tunnel: w1708 -> [w1717]
                            tunnel: [enum16{"Wait", "OFF", "ON", "Start"}."ON"] -> w1707
                            tunnel: [w1717] -> w1705
                            frame #0 {
                            }
                          }
                        }
                      }
                      n636 = property class="Bool (strict)"(reference=w1677, error in=w1672) -> ("Value"=w1676:bool)  [unwired: 2 out]
                      n637 = Select(t=enum16{"Wait", "OFF", "ON", "Start"}."Wait", s=w1676, f=w1675) -> (s? t:f=w1674:enum16{"Wait", "OFF", "ON", "Start"})
                    }
                  }
                }
                n638 = flat-sequence {
                  tunnel: [enum16{"Stop", "CoolingON", "HotGunON", "Start"}."Stop"] -> w1555
                  tunnel: w1554 -> [_]
                  frame #0 {
                  }
                }
              }
            }
          }
        }
      }
      "CurrentTest" <- w231
    }
    n639 = flat-sequence {
      tunnel: w218 -> [_]
      frame #0 {
        w226 = T14."Enabled" ("Disabled")
        w227 = FALSE ("Start")
        n640 = property on="Start" class="Bool (strict)"("Value"=w227, "DisabledEnum"=w226) -> ()  [unwired: 2 in, 2 out]
        n641 = property on="Report" class="Bool (strict)"("Value"=w227, "DisabledEnum"=w226) -> ()  [unwired: 2 in, 2 out]
      }
    }
  }
  n642 = while {
    shift-right: [w1723] -> _
    shift-left: T4."Initialize" -> [w1742]
    shift-right: [w1739] -> _
    shift-left: _ -> [w1738]
    shift-right: [w1737] -> _
    shift-left: w32 -> [w1735]
    shift-right: [w1736] -> _
    shift-left: refnum<vi> refnum ("Config_CANAT") -> [w1734]
    shift-right: [w1732] -> _
    shift-left: w29 -> [w1733]
    tunnel: "ATR" -> [_]
    tunnel: w22 -> [w1731]
    tunnel: w21 -> [w1730]
    shift-right: [w1728] -> _
    shift-left: w1 -> [w1729]
    tunnel: w8 -> [w1727]
    tunnel: w2 -> [w1726]
    tunnel: w19 -> [_]
    tunnel: w30 -> [w1741]
    tunnel: [w1740] -> _
    tunnel: w9 -> [_]
    tunnel: w6 -> [w1724]
    shift-right: [w1721] -> _
    shift-left: w1 -> [w1722]
    shift-right: [w1719] -> _
    shift-left: w1 -> [w1720]
    stop <- w1725 stop-if-true
    n643 = case shown="\"Erase ATR Table\", Default" w1742 {
      tunnel: [T4."MainProgram" w1894 w1966 T4."Erase ATR Table"] -> w1723
      tunnel: [FALSE w1880 FALSE FALSE] -> w1725
      tunnel: [w1762 w1885 w1960 w2751] -> w1740
      tunnel: w1741 -> [_ w1857 w1964 _]
      tunnel: [w1757 refnum<visa-resource-name> refnum ("VISA resource name") w1961 w2771] -> w1739
      tunnel: w1738 -> [_ w1910 w1962 _]
      tunnel: [w1784 w1874 w1956 w2768] -> w1737
      tunnel: [w1765 refnum<vi> refnum ("Config_CANAT") w1957 w2752] -> w1736
      tunnel: w1735 -> [w1784 w1912 w1959 w2768]
      tunnel: w1734 -> [_ w1897 w1958 w2752]
      tunnel: w1733 -> [w1783 w1905 w1955 w2767]
      tunnel: [w1783 w1873 w1954 w2767] -> w1732
      tunnel: w1731 -> [_ _ w1953 _]
      tunnel: w1730 -> [_ _ w1952 _]
      tunnel: w1729 -> [w1781 w1899 w1951 w2765]
      tunnel: [w1781 w1899 w1950 w2765] -> w1728
      tunnel: w1727 -> [w1780 _ w1949 _]
      tunnel: w1726 -> [_ _ w1948 _]
      tunnel: w1724 -> [_ _ w1947 _]
      tunnel: w1722 -> [_ _ w1946 _]
      tunnel: [w1777 w1872 w1945 w2758] -> w1721
      tunnel: w1720 -> [_ _ w1944 _]
      tunnel: [w1777 w1872 w1943 w2758] -> w1719
      frame "Erase ATR Table", Default {
        w1764 = refnum<visa-resource-name> "COMx" ("VISA Kinetics")
        w1777 = 0
        w1779 = T14."Enabled" ("Disabled")
        w1786 = FALSE ("Visible")
        n644 = property on="Serial Com" class="Bool"(error in=errorcluster {"status"=FALSE, "code"=0, "source"=""} ("error out"), "Visible"=TRUE) -> (error out=w1782:errorcluster)  [unwired: 1 in, 1 out]
        n645 = property on="VISA Kinetics" class="VISAName"(error in=w1782, "Visible"=w1786, "Value"=w1764) -> (error out=w1788:errorcluster)  [unwired: 1 in, 1 out]
        n646 = property on="Status" class="Bool (strict)"(error in=w1788, "Value"=w1786) -> (error out=w1775:errorcluster)  [unwired: 1 in, 1 out]
        n647 = property on="Pannel User Message" class="Str"(error in=w1775, "Value"="Select a UUT from list bellow:") -> (error out=w1774:errorcluster)  [unwired: 1 in, 1 out]
        n648 = call "UUT select.vi"("error constant"=w1774) -> ("error constant 2"=w1773:errorcluster, 2:"UUT Out"=w1767:string, 3:"UUT Out"=w1772:u16)  [unwired: 8 in]
        n649 = call "ATRBuild.vi"("error constant"=w1773, "UUT In"=w1772) -> ("error constant 2"=w1771:errorcluster, "TestArray Out"=w1770:string[][])  [unwired: 8 in]
        n650 = for {
          tunnel: w1770 -> [w1847] mode=indexing
          tunnel: w1771 -> [w1845]
          tunnel: [w1844] -> w1778
          tunnel: w1770 -> [w1843]
          i -> [w1846]
          n651 = for {
            tunnel: w1847 -> [_] mode=indexing
            tunnel: w1846 -> [w1853]
            tunnel: w1845 -> [w1850]
            tunnel: [w1849] -> w1844
            tunnel: w1843 -> [w1848]
            i -> [w1854]
            n652 = Bundle By Name(cluster=T15 {"Row"=0, "Column"=0} ("Active Cell:Active Cell"), "Row"=w1853, "Column"=w1854) -> (w1852:T15)
            n653 = control-ref of="ATR"() -> (w1851:refnum<vi>)
            n654 = property class="Tbl (strict)"(reference=w1851, error in=w1850, "Active Cell"=w1852, "Cell BG Color"=u32 16777226, "Value"=w1848) -> (error out=w1849:errorcluster)  [unwired: 1 out]
          }
        }
        n655 = call "DataFrom_ini (SubVI).vi"("error in (no error)"=w1778, "UUT"=w1767, "appended path"=w1780) -> ("error out"=w1755:errorcluster, "FileName"=w1758:string, "Next SN"=→"Next SN":i32, "UUT SoftwareVer"=w1745:string, "PN"=→"PN":string)  [unwired: 4 in]
        "UUT SoftwareVer" <- w1745
        "FileName" <- w1758
        n656 = control-ref of="ATR"() -> (w1750:refnum<vi>)
        n657 = for {
          tunnel: w1755 -> [w1796]
          tunnel: w1750 -> [w1794]
          tunnel: string[] ["RS232 Comm. + Version", "CAN Comm."] -> [w1793] mode=indexing
          tunnel: w1745 -> [w1792]
          tunnel: [w1791] -> w1753
          tunnel: [w1790] -> w1749
          n658 = call "Find_Number_LineMARVIN.vi"("Test Paragraph"=w1793, "error in"=w1796, "TableIn"=w1794) -> ("error out"=w1795:errorcluster, "Line number"=w1790:i32)  [unwired: 2 in, 2 out]
          n659 = call "InsertSingleData.vi"("String In"=w1792, "error in (no error)"=w1795, "Col"=2, "Row"=w1790, "Table in"=w1794) -> ("error out"=w1791:errorcluster)  [unwired: 6 in]
        }
        n660 = control-ref of="This VI"() -> (w1746:refnum<vi>)
        n661 = call "COM UUT Board.vi"("error in (no error)"=w1753, "VI reference (current VI)"=w1746, "VISA resource name 2"=w1764) -> ("error out"=w1761:errorcluster, ".not. x?"=w1760:bool, "VISA resource name out"=w1759:refnum<visa-resource-name>)  [unwired: 6 in]
        n662 = case shown="True" w1760 {
          tunnel: w1761 -> [w1798 w1821]
          tunnel: w1759 -> [w1799 w1820]
          tunnel: [w1799 w1811] -> w1757
          tunnel: [w1798 w1805] -> w1756
          tunnel: w1758 -> [_ w1804]
          tunnel: w1745 -> [_ w1800]
          frame False {
          }
          frame True {
            n663 = VISA Flush I/O Buffer(VISA resource name=w1820, error in (no error)=w1821) -> (VISA resource name out=w1811:refnum<visa-resource-name>, error out=w1819:errorcluster)  [unwired: 1 in]
            n664 = call "Display Message to User2"("error in (no error)"=w1819) -> ("error out"=w1818:errorcluster, "Yes"=w1817:bool)  [unwired: 9 in]
            n665 = case shown="True" w1817 {
              tunnel: w1818 -> [w1822 w1842]
              tunnel: [w1822 w1825] -> w1816
              tunnel: w1811 -> [_ w1840]
              tunnel: w1804 -> [_ w1833]
              frame False {
              }
              frame True {
                w1826 = u16 11 items=["Init", "0 ohm", "6 ohm", "13.2 ohm", "15 ohm", "25.9 ohm", "33 ohm", "Down", "Up", "Venable", "Firmware", "PowerSuply"] ("Operation")
                w1831 = u16 11 items=["Init", "0 ohm", "6 ohm", "13.2 ohm", "15 ohm", "25.9 ohm", "33 ohm", "Down", "Up", "Venable", "Firmware", "PowerSuply"] ("Operation")
                n666 = local read "DAQmx Device Name"() -> (w1823:tag)
                n667 = call "SetParam.vi"("RS"=TRUE, "error in (no error)"=w1842, "Visa"=w1840, "Filein"=w1833) -> ("error out"=w1829:errorcluster)  [unwired: 7 in]
                n668 = call "Operation (SubVI).vi"("error in (no error)"=w1829, "On/Off"=FALSE, "Operation"=w1831, "DAQmx Device Name"=w1823) -> ("error out"=w1828:errorcluster)  [unwired: 7 in]
                n669 = control-ref of="Pannel User Message"() -> (w1839:refnum<vi>)
                n670 = control-ref of="Motor Speed RPM Serial"() -> (w1837:refnum<vi>)
                n671 = control-ref of="Stop Button"() -> (w1838:refnum<vi>)
                n672 = call "Write panel message Kinetics (SubVI).vi"(4:"rpm"=w1837, 5:"rpm"=FALSE ("rpm"), "PrintTime"=TRUE, "Stop"=w1838, "error in (no error)"=w1828, "Time to wait"=20.0, "Strin"="Restart the UUT\nPlease wait...", "String in"=w1839) -> ("error out"=w1824:errorcluster)  [unwired: 3 in]
                n673 = call "Operation (SubVI).vi"("error in (no error)"=w1824, "On/Off"=TRUE, "Operation"=w1826, "DAQmx Device Name"=w1823) -> ("error out"=w1825:errorcluster)  [unwired: 7 in]
              }
            }
            n674 = call "SerialMarvinSendGet.vi"("error in (no error)"=w1816, "write buffer"="SN\r\n", "VISA resource name"=w1811) -> ("error out"=w1812:errorcluster, "read buffer"=w1806:string)  [unwired: 7 in]
            n675 = property on="UUT SN Report" class="Str"("Value"=w1806) -> ()  [unwired: 2 in, 2 out]
            n676 = Decimal String To Number(string=w1806) -> (number=→"Current SN":i32)  [unwired: 2 in, 1 out]
            n677 = call "SerialMarvinSendGet.vi"("error in (no error)"=w1812, "write buffer"="VR\r\n", "VISA resource name"=w1811) -> ("error out"=w1807:errorcluster, "read buffer"=w1801:string)  [unwired: 7 in]
            n678 = control-ref of="ATR"() -> (w1808:refnum<vi>)
            n679 = call "Find_Number_LineMARVIN.vi"("Test Paragraph"="RS232 Comm. + Version", "TableIn"=w1808) -> ("Line number"=w1809:i32)  [unwired: 3 in, 3 out]
            n680 = Equal?(x=w1801, y=w1800) -> (x = y?=w1802:bool)
            n681 = call "PassOrFail (SubVI).vi"("String Res"=w1801, "index (row)"=w1809, "error in (no error)"=w1807, "Data in"=-3.0, "Pass?Fail"=w1802, "Table in"=w1808) -> ("error out"=w1805:errorcluster)  [unwired: 5 in]
          }
        }
        n682 = call "KineticsCan.vi"("error in"=w1756) -> ("error out"=w1752:errorcluster, "Version"=w1743:string, "Res_Pass_T"=→"CAN Status":bool, "Config_CANAT_out"=w1765:refnum<vi>)  [unwired: 7 in]
        n683 = Equal?(x=w1743, y=w1745) -> (x = y?=w1744:bool)
        n684 = call "PassOrFail (SubVI).vi"("String Res"=w1743, "index (row)"=w1749, "error in (no error)"=w1752, "Data in"=-3.0, "Pass?Fail"=w1744, "Table in"=w1750) -> ("error out"=w1751:errorcluster)  [unwired: 5 in]
        n685 = property on="Start" class="Bool (strict)"(error in=w1751, "DisabledEnum"=w1779) -> (error out=w1763:errorcluster)  [unwired: 1 in, 1 out]
        n686 = property on="Report" class="Bool (strict)"(error in=w1763, "DisabledEnum"=w1779) -> (error out=w1762:errorcluster)  [unwired: 1 in, 1 out]
      }
      frame "Stop" {
        w1872 = 0
        n687 = control-ref of="ATR"() -> (w1871:refnum<vi>)
        n688 = call "PassFailUUT (SubVI).vi"("error in (no error)"=w1857, "Table in"=w1871) -> ("PassFaileUUTresult"=w1864:bool)  [unwired: 7 in, 2 out]
        n689 = property on="Test Failed" class="Bool (strict)"("Value"=w1864) -> ()  [unwired: 2 in, 2 out]
        n690 = flat-sequence {
          tunnel: w1857 -> [w1940]
          tunnel: [w1939] -> w1898
          frame #0 {
            n691 = control-ref of="Pannel User Message"() -> (w1942:refnum<vi>)
            n692 = property class="Str"(reference=w1942, error in=w1940, "Value"="Program Stopped...\r\nPlease turn OFF All Power sinks") -> (error out=w1939:errorcluster)  [unwired: 1 out]
          }
        }
        n693 = Select(t="PASS" ("name or relative path"), s=w1864, f="FAIL" ("name or relative path")) -> (s? t:f=w1863:string)
        n694 = call <vilib>:"Application Directory.vi"() -> ("Application Directory"=w1867:path)
        n695 = Build Path(base path=w1867, name or relative path="data\\TestResult.ini") -> (appended path=w1870:path)
        n696 = call <vilib>:"Open Config Data.vi"("configuration file path"=w1870) -> ("error out"=w1868:errorcluster, "refnum"=w1869:T5)  [unwired: 2 in, 7 out]
        n697 = call-poly <vilib>:"Write Key.vi"("section"="Kinetics", "error in (no error)"=w1868, "value"=w1863, "key"="Result", "refnum"=w1869) -> ("error out"=w1866:errorcluster, "refnum out"=w1865:T5)  [unwired: 4 in, 1 out]
        n698 = call <vilib>:"Close Config Data.vi"("error in (no error)"=w1866, "refnum"=w1865) -> ()  [unwired: 8 in, 2 out]
        n699 = disable-structure shown="Enabled" {
          disable-tunnel: w1898 -> [w1927 w1928]
          disable-tunnel: w1897 -> [w1925 _]
          disable-tunnel: [w1924 w1928] -> w1884
          frame Disabled {
            n700 = call "Clear CAN Buffer.vi"("error in (no error)"=w1927, "Cluster in"=w1925) -> ("error out"=w1926:errorcluster)  [unwired: 8 in, 1 out]
            n701 = call "Close CAN Device.vi"("error in (no error)"=w1926, "Cluster in"=w1925) -> ("error out"=w1924:errorcluster)  [unwired: 8 in, 1 out]
          }
          frame Enabled {
          }
        }
        n702 = VISA Close(VISA resource name=w1910, error in (no error)=w1898) -> (error out=w1904:errorcluster)
        n703 = property on="Stop Button" class="Bool (strict)"() -> ("Value"=w1876:bool)  [unwired: 2 in, 2 out]
        n704 = call "TesterOption (SubVI).vi"("2 Options"=FALSE, "On/Off"=FALSE, "Tester Option"=T6."Power") -> ("error out"=w1893:errorcluster, "VISA Refnum out"=w1903:refnum<visa-resource-name>)  [unwired: 7 in]
        n705 = property on="ClosePanel" class="Bool (strict)"() -> ("Value"=w1877:bool)  [unwired: 2 in, 2 out]
        n706 = VISA Close(VISA resource name=w1903, error in (no error)=w1893) -> (error out=w1890:errorcluster)
        n707 = Or(x=w1877, y=w1876) -> (x .or. y?=w1875:bool)
        n708 = Flush Queue(queue=w1905, error in (no error)=w1904) -> (queue out=w1907:refnum<queue>, error out=w1906:errorcluster)  [unwired: 1 out]
        n709 = Flush Queue(queue=w1912, error in (no error)=w1904) -> (queue out=w1911:refnum<queue>, error out=w1913:errorcluster)  [unwired: 1 out]
        n710 = case shown="False" w1875 {
          tunnel: w1913 -> [w1915 w1923]
          tunnel: w1911 -> [w1917 w1919]
          tunnel: w1907 -> [w1916 w1918]
          tunnel: w1906 -> [w1914 w1922]
          tunnel: [w1915 w1921] -> w1892
          tunnel: [w1914 w1920] -> w1891
          tunnel: [w1917 w1919] -> w1874
          tunnel: [w1916 w1918] -> w1873
          frame False {
          }
          frame True {
            n711 = Release Queue(queue=w1918, error in (no error)=w1922) -> (error out=w1920:errorcluster)  [unwired: 1 in, 2 out]
            n712 = Release Queue(queue=w1919, error in (no error)=w1923) -> (error out=w1921:errorcluster)  [unwired: 1 in, 2 out]
          }
        }
        n713 = Merge Errors(w1892, w1891, w1890, w1884) -> (w1889:errorcluster)
        n714 = property on="Refresh Button" class="Bool (strict)"() -> ("Value"=w1878:bool)  [unwired: 2 in, 2 out]
        n715 = call <vilib>:"Clear Errors.vi"("error in (no error)"=w1889) -> ("error out"=w1888:errorcluster)  [unwired: 5 in, 1 out]
        n716 = property on="Stop Button" class="Bool (strict)"() -> ("Value"=w1882:bool)  [unwired: 2 in, 2 out]
        n717 = property on="ClosePanel" class="Bool (strict)"(error in=w1888) -> (error out=w1886:errorcluster, "Value"=w1887:bool)  [unwired: 1 in, 1 out]
        n718 = Not(x=w1878) -> (.not. x?=w1879:bool)
        n719 = Select(t=T4."Initialize", s=w1878, f=T4."Stop") -> (s? t:f=w1894:T4)
        n720 = Not(x=w1882) -> (.not. x?=w1881:bool)
        n721 = Compound Arithmetic op=AND(w1887, w1881, w1879) -> (w1883:bool)
        n722 = case shown="False" w1883 {
          tunnel: w1886 -> [w1931 w1935]
          tunnel: [w1931 w1935] -> w1885
          tunnel: [w1930 w1934] -> w1880
          tunnel: w1878 -> [w1929 _]
          frame False {
            n723 = case shown="False" w1929 {
              tunnel: [TRUE FALSE] -> w1930
              frame False {
              }
              frame True {
              }
            }
          }
          frame True {
            n724 = flat-sequence {
              tunnel: [TRUE] -> w1934
              frame #0 {
              }
              frame #1 {
                n725 = control-ref of="This VI"() -> (w1938:refnum<vi>)
                n726 = property class="VI"(reference=w1938, "FP.State"=T16."Closed" ("Front Panel Window:State")) -> ()  [unwired: 1 in, 2 out]
              }
            }
          }
        }
      }
      frame "MainProgram" {
        n727 = event shown="[0] Timeout" {
          selector: w1953 -> [_ _ _ _ _ _ _ _ _ _ _ _ _]
          dyn-events: _ -> [_ _ _ _ _ _ _ _ _ _ _ _ _]
          timeout: 5000 -> [_ _ _ _ _ _ _ _ _ _ _ _ _]
          tunnel: [T4."MainProgram" T4."MainProgram" T4."MainProgram" T4."MainProgram" T4."MainProgram" T4."Stop" T4."MainProgram" w2583 T4."MainProgram" T4."MainProgram" T4."MainProgram" T4."Stop" T4."MainProgram"] -> w1966
          tunnel: [w1972 w2081 w2152 w2161 w2172 w2192 w2210 w2631 w2702 w2717 _ w2739 w2740] -> w1960
          tunnel: w1964 -> [w1981 w2081 w2151 w2163 w2172 w2192 w2217 w2631 w2703 w2716 w2724 w2739 w2740]
          tunnel: [w1969 w2075 w2153 w2162 w2173 w2190 w2206 w2588 w2700 w2714 _ w2737 w2744] -> w1961
          tunnel: w1962 -> [w1969 w2075 w2153 w2162 w2173 w2190 w2206 w2588 w2700 w2714 _ w2737 w2744]
          tunnel: w1959 -> [w1983 w2087 w2147 w2158 w2169 w2189 w2215 w2615 w2699 w2713 w2728 w2736 w2747]
          tunnel: w1958 -> [w1979 w2086 w2148 w2159 w2170 w2188 w2197 w2614 w2698 w2712 w2727 w2735 w2743]
          tunnel: [w1980 w2086 w2148 w2159 w2170 w2188 w2197 w2614 w2698 w2712 w2727 w2735 w2743] -> w1957
          tunnel: [w1982 w2087 w2147 w2158 w2169 w2189 w2215 w2615 w2699 w2713 w2728 w2736 w2747] -> w1956
          tunnel: w1955 -> [w1977 w2085 w2146 w2157 w2168 w2187 w2214 w2613 w2697 w2711 w2726 w2734 w2746]
          tunnel: [w1977 w2085 w2146 w2157 w2168 w2187 w2209 w2613 w2697 w2711 w2726 w2734 w2746] -> w1954
          tunnel: w1952 -> [_ _ _ _ _ _ _ w2560 _ _ _ _ _]
          tunnel: w1951 -> [w1978 w2084 w2145 w2156 w2167 w2185 w2204 w2592 w2696 w2710 w2725 w2733 w2745]
          tunnel: [w1978 w2084 w2145 w2156 w2167 w2185 w2204 w2591 w2696 w2710 w2725 w2733 w2745] -> w1950
          tunnel: w1949 -> [_ w2082 _ _ _ _ _ w2590 _ _ _ _ _]
          tunnel: w1948 -> [_ w2074 _ _ _ _ _ _ _ _ _ _ _]
          tunnel: w1947 -> [_ _ _ _ _ _ _ _ w2695 _ _ _ _]
          tunnel: w1946 -> [_ w2055 w2144 w2155 w2166 w2182 w2196 w2562 w2693 w2709 w2722 w2732 w2742]
          tunnel: [_ w2055 w2144 w2155 w2166 w2182 w2196 w2562 w2693 w2709 w2722 w2732 w2742] -> w1945
          tunnel: w1944 -> [w1971 w2054 w2143 w2154 w2165 w2181 w2195 w2551 w2692 w2708 w2721 w2731 w2741]
          tunnel: [w1970 w2054 w2143 w2154 w2165 w2181 w2195 w2551 w2692 w2708 w2721 w2731 w2741] -> w1943
          event Timeout {
            n728 = event-data() -> ()  [unwired: 1 in, 3 out]
            n729 = property on="Automation" class="Bool (strict)"() -> ("Value"=w1974:bool)  [unwired: 2 in, 2 out]
            n730 = property on="Start" class="Bool (strict)"() -> ("Value"=w1976:bool)  [unwired: 2 in, 2 out]
            n731 = disable-structure shown="Enabled" {
              disable-tunnel: w1983 -> [w2000 w2052]
              disable-tunnel: [w1999 w2052] -> w1982
              disable-tunnel: w1981 -> [w1998 w2051]
              disable-tunnel: [w1997 w2049] -> w1980
              disable-tunnel: w1979 -> [w1996 w2049]
              disable-tunnel: [w1993 w2051] -> w1972
              disable-tunnel: w1971 -> [w1991 w2050]
              disable-tunnel: [w1990 w2050] -> w1970
              frame Disabled {
                n732 = property class="Clust (strict)"(reference=w1996, error in=w1998) -> (reference out=w1997:refnum<vi>, error out=w1992:errorcluster, "Value"=w2003:T25)
                n733 = Unbundle By Name(w2003) -> ("DevType"=w2004:T19, "CanIndex"=w2002:T20)
                n734 = call "VCI_Receive.vi"("CANIndex"=w2002, "DevIndex"=u32 0, "DevType"=w2004) -> ("Recieve"=w2001:T26[])  [unwired: 3 in, 5 out]
                n735 = Empty Array?(array=w2001) -> (empty?=w1995:bool)
                n736 = case shown="False" w1995 {
                  tunnel: w2002 -> [w2018 _]
                  tunnel: w1997 -> [w2016 _]
                  tunnel: w2000 -> [w2015 w2048]
                  tunnel: w1992 -> [w2014 w2047]
                  tunnel: w2001 -> [w2019 _]
                  tunnel: [w2009 w2047] -> w1993
                  tunnel: [w2008 w2048] -> w1999
                  tunnel: [TRUE w2042] -> w1994
                  tunnel: w1991 -> [_ w2046]
                  tunnel: [0 w2045] -> w1990
                  frame False {
                    n737 = call "Demo_MakeDispBuff.vi"("Channel"=w2018, "Type"=enum16{"接收", "发送"}."接收", "OBJs"=w2019) -> ("Buffer"=w2017:T27)
                    n738 = for {
                      N: 3 -> [_]
                      tunnel: w2017 -> [w2033]
                      tunnel: w2016 -> [w2032]
                      tunnel: w2015 -> [w2023]
                      tunnel: w2014 -> [w2022]
                      tunnel: [w2025] -> w2012 mode=indexing
                      tunnel: [w2023] -> w2011
                      tunnel: [w2022] -> w2010
                      i -> [w2021]
                      n739 = property class="Clust (strict)"(reference=w2032) -> ("Value"=w2030:T25)  [unwired: 1 in, 2 out]
                      n740 = Index Array(array=w2033, index=w2021) -> (element=w2026:T28)
                      n741 = Unbundle By Name(w2026) -> ("Channel"=w2028:T20, "VCI_CAN_OBJ"=w2031:T26)  [unwired: 2 out]
                      n742 = Unbundle By Name(w2030) -> ("CanIndex"=w2029:T20)
                      n743 = Equal?(x=w2029, y=w2028) -> (x = y?=w2027:bool)
                      n744 = case shown="True" w2027 {
                        tunnel: w2031 -> [_ w2041]
                        tunnel: [w2034 w2037] -> w2025
                        tunnel: T17 {"ID"=0, "MSGTYPE"=0, "LEN"=0, "aDATA"=[]} ("Msg") -> [w2034 w2036]
                        frame False {
                        }
                        frame True {
                          n745 = Unbundle By Name(w2041) -> ("ID"=w2035:u32, "DataLen"=w2040:u8, "Data"=w2038:u8[])
                          n746 = Bundle By Name(cluster=w2036, "ID"=w2035, "MSGTYPE"=u8 0, "LEN"=w2040, "aDATA"=w2038) -> (w2037:T17)
                        }
                      }
                    }
                    n747 = Enqueue Element(queue=w2011, element=w2012, error in (no error)=w2010) -> (queue out=w2008:refnum<queue>, error out=w2009:errorcluster)  [unwired: 2 out]
                  }
                  frame True {
                    n748 = Increment(x=w2046) -> (x+1=w2045:i32)
                    n749 = Greater Or Equal?(x=w2045, y=7) -> (x >= y?=w2043:bool)
                    n750 = Not(x=w2043) -> (.not. x?=w2042:bool)
                  }
                }
                n751 = property on="CAN Status" class="Bool (strict)"("Value"=w1994) -> ()  [unwired: 2 in, 2 out]
              }
              frame Enabled {
              }
            }
            n752 = Or(x=w1974, y=w1976) -> (x .or. y?=w1975:bool)
            n753 = property on="ClosePanel" class="Bool (strict)"("Value"=FALSE ("ClosePanel")) -> ()  [unwired: 2 in, 2 out]
            n754 = case shown="False" w1975 {
              frame False {
                n755 = property on="Pannel User Message" class="Str"("Value"="You can press start to execute(s) test(s).") -> ()  [unwired: 2 in, 2 out]
              }
              frame True {
              }
            }
            n756 = Not Equal?(x=w1969, y=refnum<visa-resource-name> "COMx") -> (x != y?=w1967:bool)
            n757 = case shown="True" w1967 {
              tunnel: w1969 -> [_ w1989]
              frame False {
              }
              frame True {
                n758 = call "Serial.vi"("Clear Log"=FALSE, "write buffer"="VC\r\n", "VISA resource name"=w1989) -> ("read buffer"=w1986:string)  [unwired: 7 in, 1 out]
                n759 = Fract/Exp String To Number(string=w1986) -> (number=→"Motor Speed RPM Serial":dbl)  [unwired: 3 in, 1 out]
              }
            }
          }
          event "SetSN": Value Change {
            n760 = event-data() -> ()  [unwired: 1 in, 6 out]
            n761 = property on="UUT" class="DigNum (strict)"() -> ("Value"=w2065:u8)  [unwired: 2 in, 2 out]
            n762 = Equal?(x=w2065, y=u8 95) -> (x = y?=w2063:bool)
            n763 = control-ref of="ATR"() -> (w2066:refnum<vi>)
            n764 = Select(t=u8 50 ("y"), s=w2063, f=u8 36 ("y")) -> (s? t:f=w2058:u8)
            n765 = property on="Current SN" class="DigNum (strict)"(error in=w2081) -> (error out=w2060:errorcluster, "Value"=w2080:i32)  [unwired: 1 in, 1 out]
            n766 = call "PassFailUUT (SubVI).vi"("error in (no error)"=w2060, "Table in"=w2066) -> ("Total Pass"=w2059:u8)  [unwired: 7 in, 2 out]
            n767 = Equal To 0?(x=w2080) -> (x = 0?=w2077:bool)
            n768 = Equal?(x=w2080, y=-1) -> (x = y?=w2078:bool)
            n769 = Equal?(x=w2059, y=w2058) -> (x = y?=w2057:bool)
            n770 = Or(x=w2078, y=w2077) -> (x .or. y?=w2076:bool)
            n771 = property on="CAN Status" class="Bool (strict)"() -> ("Value"=w2067:bool)  [unwired: 2 in, 2 out]
            n772 = property on="Status" class="Bool (strict)"() -> ("Value"=w2072:bool)  [unwired: 2 in, 2 out]
            n773 = And(x=w2072, y=w2067) -> (x .and. y?=w2068:bool)
            n774 = case shown="True" w2068 {
              tunnel: w2082 -> [_ w2101]
              tunnel: w2076 -> [_ w2090]
              tunnel: w2075 -> [_ w2100]
              tunnel: w2074 -> [_ w2099]
              tunnel: [errorcluster {"status"=FALSE, "code"=0, "source"=""} ("error out") w2098] -> w2071
              tunnel: [w2088 w2097] -> w2073
              tunnel: w2057 -> [_ w2091]
              frame False {
                w2088 = FALSE ("Value")
                n775 = property on="SetSN" class="Bool (strict)"("Value"=w2088) -> ()  [unwired: 2 in, 2 out]
                n776 = call "Display Message to User10"() -> ()  [unwired: 10 in, 2 out]
              }
              frame True {
                n777 = property on="Test Failed" class="Bool (strict)"() -> ("Value"=w2095:bool)  [unwired: 2 in, 2 out]
                n778 = property on="Automation" class="Bool (strict)"() -> ("Value"=w2097:bool)  [unwired: 2 in, 2 out]
                n779 = Not(x=w2095) -> (.not. x?=w2096:bool)
                n780 = Select(t=w2096, s=w2097, f=w2099) -> (s? t:f=w2093:bool)
                n781 = Or(x=w2091, y=w2093) -> (x .or. y?=w2092:bool)
                n782 = And(x=w2090, y=w2092) -> (x .and. y?=w2094:bool)
                n783 = case shown="True" w2094 {
                  tunnel: w2101 -> [_ w2131]
                  tunnel: w2100 -> [_ w2124]
                  tunnel: [w2103 w2116] -> w2098
                  tunnel: w2090 -> [w2102 _]
                  frame False {
                    n784 = case shown="True" w2102 {
                      tunnel: [w2105 w2106] -> w2103
                      frame False {
                        n785 = call "Display Message to User9"() -> ("error out"=w2105:errorcluster)  [unwired: 10 in, 1 out]
                      }
                      frame True {
                        n786 = call "Display Message to User3"() -> ("error out"=w2106:errorcluster)  [unwired: 10 in, 1 out]
                      }
                    }
                    n787 = property on="Automation" class="Bool (strict)"(error in=w2103, "Value"=FALSE ("Automation")) -> ()  [unwired: 1 in, 2 out]
                  }
                  frame True {
                    w2123 = FALSE ("SetSN")
                    n788 = property on="Next SN" class="DigNum (strict)"() -> ("Value"=w2108:i32)  [unwired: 2 in, 2 out]
                    n789 = call "TesterOption (SubVI).vi"("2 Options"=FALSE, "On/Off"=FALSE, "Tester Option"=T6."Venable") -> ("error out"=w2110:errorcluster)  [unwired: 7 in, 1 out]
                    n790 = call <vilib>:"Clear Errors.vi"("error in (no error)"=w2110) -> ("error out"=w2111:errorcluster)  [unwired: 5 in, 1 out]
                    n791 = Number To Decimal String(number=w2108) -> (decimal integer string=w2109:string)  [unwired: 1 in]
                    "UUT SN Report" <- w2109
                    n792 = Search and Replace String(input string="EP=1\r\nSN=0\r\n" ("write buffer"), search string="0", replace string=w2109) -> (result string=w2126:string)  [unwired: 5 in, 3 out]
                    n793 = call "SerialMarvinSendGet.vi"("error in (no error)"=w2111, "Clear Log"=FALSE, "write buffer"=w2126, "VISA resource name"=w2124) -> ("error out"=w2115:errorcluster)  [unwired: 6 in, 1 out]
                    n794 = property on="UUT" class="DigNum (strict)"(error in=w2115) -> ("Value"=w2132:u8)  [unwired: 1 in, 2 out]
                    n795 = case shown="47" w2132 {
                      tunnel: ["AHU R Serial Number" ("key") "AHU L Serial Number" ("key") "EBAY Serial Number" ("key")] -> w2135
                      tunnel: [2 2 1] -> w2107
                      frame 63, Default {
                      }
                      frame 47 {
                      }
                      frame 95 {
                      }
                    }
                    n796 = call <vilib>:"Open Config Data.vi"("create file if necessary (T)"=FALSE, "configuration file path"=w2131) -> ("error out"=w2129:errorcluster, "refnum"=w2130:T5)  [unwired: 1 in, 7 out]
                    n797 = call-poly <vilib>:"Write Key.vi"("section"="Marvin", "error in (no error)"=w2129, "value"=w2109, "key"=w2135, "refnum"=w2130) -> ("error out"=w2119:errorcluster, "refnum out"=w2118:T5)  [unwired: 4 in, 1 out]
                    n798 = call <vilib>:"Close Config Data.vi"("error in (no error)"=w2119, "refnum"=w2118) -> ("error out"=w2117:errorcluster)  [unwired: 8 in, 1 out]
                    n799 = property on="Current SN" class="DigNum (strict)"("Value"=w2108) -> ()  [unwired: 2 in, 2 out]
                    n800 = property on="SetSN" class="Bool (strict)"(error in=w2117, "Value"=w2123) -> (error out=w2122:errorcluster)  [unwired: 1 in, 1 out]
                    n801 = property on="Automation" class="Bool (strict)"(error in=w2122, "Value"=w2123) -> (error out=w2121:errorcluster)  [unwired: 1 in, 1 out]
                    n802 = Add(x=w2108, y=w2107) -> (x+y=w2120:i32)
                    n803 = property on="Next SN" class="DigNum (strict)"(error in=w2121, "Value"=w2120) -> (error out=w2116:errorcluster)  [unwired: 1 in, 1 out]
                  }
                }
              }
            }
            n804 = call <vilib>:"Clear Errors.vi"("error in (no error)"=w2071) -> ("error out"=w2056:errorcluster)  [unwired: 5 in, 1 out]
            n805 = property on="SetSN" class="Bool (strict)"(error in=w2056, "Value"=FALSE ("SetSN")) -> (error out=w2070:errorcluster)  [unwired: 1 in, 1 out]
            n806 = case shown="True" w2073 {
              tunnel: w2070 -> [_ _]
              frame False {
              }
              frame True {
                w2142 = TRUE ("Value (Signaling)")
                n807 = property on="Report" class="Bool (strict)"("Val(Sgnl)"=w2142, "Value"=w2142) -> ()  [unwired: 2 in, 2 out]
              }
            }
          }
          event "ATR": Mouse Enter {
            n808 = event-data() -> ()  [unwired: 1 in, 4 out]
            n809 = call-poly <vilib>:"Set Cursor.vi"("error in (no error)"=w2151, "icon"=u16 1) -> ("error out"=w2152:errorcluster)  [unwired: 8 in, 1 out]
          }
          event "ATR": Mouse Leave {
            n810 = event-data() -> ()  [unwired: 1 in, 4 out]
            n811 = call-poly <vilib>:"Set Cursor.vi"("error in (no error)"=w2163, "icon"=u16 0) -> ("error out"=w2161:errorcluster)  [unwired: 8 in, 1 out]
          }
          event "ATR": Mouse Down? {
            n812 = event-data() -> ("Coords"=w2180:T29)  [unwired: 1 in, 4 out]
            n813 = invoke on="ATR" class="Tbl (strict)" method="Point To Row Column"("Point"=w2180) -> ("InBounds"=w2176:bool, "CellPosition"=w2175:T15)  [unwired: 5 in, 4 out]
            n814 = Greater Than 0?(x=w2175) -> (x > 0?=w2179:cluster{"Row":bool, "Column":bool})
            n815 = Cluster To Array(cluster=w2179) -> (array=w2178:bool[])
            n816 = Or Array Elements(Boolean array=w2178) -> (logical OR=w2177:bool)
            n817 = Or(x=w2176, y=w2177) -> (x .or. y?=w2174:bool)
            n818 = event-data("Discard?"=w2174) -> ()  [unwired: 1 in, 1 out]
          }
          event Panel Close? {
            n819 = event-data() -> ("VIRef"=w2186:refnum<vi>)  [unwired: 1 in, 3 out]
            n820 = Close Reference(reference=w2186) -> ()  [unwired: 1 in, 1 out]
            n821 = disable-structure shown="Disabled" {
              frame Disabled {
                n822 = property on="Stop Button" class="Bool (strict)"("Val(Sgnl)"=TRUE ("Stop Button"), "Value"=FALSE ("Stop Button")) -> ()  [unwired: 2 in, 2 out]
              }
              frame Enabled {
              }
            }
            n823 = event-data("Discard?"=TRUE) -> ()  [unwired: 1 in, 1 out]
            "ClosePanel" <- TRUE ("ClosePanel")
          }
          event "Start": Value Change {
            w2205 = T11 [] items=["Auxiliary", "Temp Sens Cal", "Com Test", "Enable Test", "Speed Command", "Stop Time", "Temp Control", "Burn in", "Visual Inspec", "Empty"]
            n824 = event-data() -> ()  [unwired: 1 in, 2 out]
            n825 = property on="UUT" class="Str"(error in=w2217) -> ("Value"=w2216:string)  [unwired: 1 in, 2 out]
            n826 = control-ref of="Pannel User Message"() -> (w2202:refnum<vi>)
            n827 = control-ref of="Stop Button"() -> (w2201:refnum<vi>)
            n828 = call "Write panel message Kinetics (SubVI).vi"("rpm"=FALSE, "PrintTime"=TRUE, "Stop"=w2201, "Strin"="TESTER BIT TEST OPERATION IN PROCESS", "String in"=w2202) -> ("error out"=w2203:errorcluster)  [unwired: 6 in]
            n829 = while {
              tunnel: w2216 -> [w2232]
              tunnel: [w2231] -> w2212
              tunnel: [w2230] -> w2211
              shift-right: [w2227] -> _
              shift-left: enum16{"Stop", "Tests", "Bit test", "Start"}."Start" -> [w2229]
              tunnel: w2206 -> [w2228]
              tunnel: w2205 -> [w2226]
              tunnel: w2203 -> [_]
              tunnel: w2201 -> [w2221]
              tunnel: w2202 -> [w2220]
              tunnel: w2197 -> [_]
              stop <- w2225 stop-if-true
              n830 = property on="CAN Status" class="Bool (strict)"() -> (error out=w2219:errorcluster, "Value"=w2222:bool)  [unwired: 2 in, 1 out]
              n831 = property on="Status" class="Bool (strict)"(error in=w2219) -> (error out=w2223:errorcluster, "Value"=w2224:bool)  [unwired: 1 in, 1 out]
              n832 = case shown="\"Start\"" w2229 {
                tunnel: w2232 -> [_ w2248 w2380 _]
                tunnel: [w2237 w2247 w2404 w2509] -> w2231
                tunnel: [w2233 w2246 w2378 w2501] -> w2230
                tunnel: w2228 -> [_ _ w2391 w2512]
                tunnel: w2220 -> [_ _ _ w2511]
                tunnel: w2221 -> [_ _ _ w2510]
                tunnel: [w2236 w2245 w2383 w2505] -> w2227
                tunnel: w2226 -> [w2237 _ w2404 w2509]
                tunnel: [w2235 w2244 FALSE FALSE] -> w2225
                tunnel: w2224 -> [_ _ _ w2507]
                tunnel: w2223 -> [w2233 _ _ _]
                tunnel: w2222 -> [_ _ _ w2502]
                frame "Stop", Default {
                  n833 = property on="Start" class="Bool (strict)"(error in=w2233, "Value"=FALSE ("Start")) -> ()  [unwired: 1 in, 2 out]
                  n834 = flat-sequence {
                    tunnel: [enum16{"Stop", "Tests", "Bit test", "Start"}."Stop"] -> w2236
                    tunnel: w2233 -> [_]
                    tunnel: [TRUE] -> w2235
                    frame #0 {
                    }
                  }
                }
                frame "Tests" {
                  w2243 = T14."Disabled and Grayed Out" ("Disabled")
                  n835 = case shown="\"EBAY\"" w2248 {
                    tunnel: [w2264 w2313] -> w2247
                    tunnel: [w2263 w2312] -> w2246
                    tunnel: [w2252 w2300] -> w2240
                    frame "AHU", Default {
                      n836 = call "Load Program Process AHU.vi"() -> ("Speed Command Test"=w2257:bool, "Enable Test"=w2258:bool, "Burn-in Test"=w2255:bool, "Auxiliary"=w2253:bool, "Temperature Sensor Calibration Test"=w2260:bool, "Communication Test"=w2259:bool, "Stop Time Test"=w2256:bool, "Visual Inspection"=w2254:bool, "OK"=w2261:bool, "Automation"=w2252:bool, "error out"=w2263:errorcluster)  [unwired: 8 in, 9 out]
                      n837 = Or(x=w2261, y=w2252) -> (x .or. y?=w2262:bool)
                      n838 = case shown="True" w2262 {
                        tunnel: [w2265 w2275] -> w2264
                        tunnel: w2252 -> [_ w2274]
                        tunnel: w2260 -> [_ w2273]
                        tunnel: w2259 -> [_ w2272]
                        tunnel: w2258 -> [_ w2271]
                        tunnel: w2257 -> [_ w2270]
                        tunnel: w2256 -> [_ w2269]
                        tunnel: w2255 -> [_ w2268]
                        tunnel: w2254 -> [_ w2267]
                        tunnel: w2253 -> [_ w2266]
                        frame False {
                          w2265 = T11 [] items=["Auxiliary", "Temp Sens Cal", "Com Test", "Enable Test", "Speed Command", "Stop Time", "Temp Control", "Burn in", "Visual Inspec", "Empty"]
                        }
                        frame True {
                          n839 = case shown="False" w2274 {
                            tunnel: [w2298 w2299] -> w2275
                            tunnel: w2273 -> [w2280 _]
                            tunnel: w2272 -> [w2279 _]
                            tunnel: w2271 -> [w2281 _]
                            tunnel: w2270 -> [w2278 _]
                            tunnel: w2269 -> [w2277 _]
                            tunnel: w2268 -> [w2291 _]
                            tunnel: w2267 -> [w2276 _]
                            tunnel: w2266 -> [_ _]
                            frame False {
                              w2284 = T1."Empty" ("f")
                              n840 = Select(t=T1."Com Test" ("f"), s=w2279, f=w2284) -> (s? t:f=w2290:T1)
                              n841 = Select(t=T1."Temp Sens Cal" ("f"), s=w2280, f=w2284) -> (s? t:f=w2289:T1)
                              n842 = Select(t=T1."Stop Time" ("f"), s=w2277, f=w2284) -> (s? t:f=w2288:T1)
                              n843 = Select(t=T1."Enable Test" ("f"), s=w2281, f=w2284) -> (s? t:f=w2287:T1)
                              n844 = Select(t=T1."Speed Command" ("f"), s=w2278, f=w2284) -> (s? t:f=w2286:T1)
                              n845 = Select(t=T1."Burn in" ("f"), s=w2291, f=w2284) -> (s? t:f=w2285:T1)
                              n846 = Select(t=T1."Visual Inspec" ("f"), s=w2276, f=w2284) -> (s? t:f=w2282:T1)
                              n847 = Build Array(w2290, w2289, w2288, w2287, w2286, w2285, w2282) -> (w2298:T11)
                            }
                            frame True {
                              w2299 = T11 [enum."Com Test", enum."Temp Sens Cal", enum."Stop Time", enum."Enable Test", enum."Speed Command", enum."Burn in", enum."Visual Inspec"] items=["Auxiliary", "Temp Sens Cal", "Com Test", "Enable Test", "Speed Command", "Stop Time", "Temp Control", "Burn in", "Visual Inspec", "Empty"]
                            }
                          }
                        }
                      }
                    }
                    frame "EBAY" {
                      n848 = call "Load Program Process EBAY.vi"() -> ("Speed Command Test"=w2306:bool, "Enable Test"=w2307:bool, "Burn-in Test"=w2304:bool, "Temperature Control Algorithm Test"=w2303:bool, "Auxiliary"=w2301:bool, "Temperature Sensor Calibration Test"=w2309:bool, "Communication Test"=w2308:bool, "Stop Time Test"=w2305:bool, "Visual Inspection"=w2302:bool, "OK"=w2310:bool, "Automation"=w2300:bool, "error out"=w2312:errorcluster)  [unwired: 8 in, 8 out]
                      n849 = Or(x=w2310, y=w2300) -> (x .or. y?=w2311:bool)
                      n850 = case shown="True" w2311 {
                        tunnel: [w2314 w2325] -> w2313
                        tunnel: w2300 -> [_ w2324]
                        tunnel: w2309 -> [_ w2323]
                        tunnel: w2308 -> [_ w2322]
                        tunnel: w2307 -> [_ w2321]
                        tunnel: w2306 -> [_ w2320]
                        tunnel: w2305 -> [_ w2319]
                        tunnel: w2304 -> [_ w2318]
                        tunnel: w2303 -> [_ w2317]
                        tunnel: w2302 -> [_ w2316]
                        tunnel: w2301 -> [_ w2315]
                        frame False {
                          w2314 = T11 [] items=["Auxiliary", "Temp Sens Cal", "Com Test", "Enable Test", "Speed Command", "Stop Time", "Temp Control", "Burn in", "Visual Inspec", "Empty"]
                        }
                        frame True {
                          n851 = case shown="False" w2324 {
                            tunnel: [w2354 w2355] -> w2325
                            tunnel: w2323 -> [w2331 _]
                            tunnel: w2322 -> [w2330 _]
                            tunnel: w2321 -> [w2329 _]
                            tunnel: w2320 -> [w2328 _]
                            tunnel: w2319 -> [w2327 _]
                            tunnel: w2318 -> [w2333 _]
                            tunnel: w2317 -> [w2332 _]
                            tunnel: w2316 -> [w2345 _]
                            tunnel: w2315 -> [w2336 _]
                            frame False {
                              w2334 = T1."Empty" ("f")
                              n852 = Select(t=T1."Com Test" ("f"), s=w2330, f=w2334) -> (s? t:f=w2344:T1)
                              n853 = Select(t=T1."Temp Sens Cal" ("f"), s=w2331, f=w2334) -> (s? t:f=w2343:T1)
                              n854 = Select(t=T1."Stop Time" ("f"), s=w2327, f=w2334) -> (s? t:f=w2342:T1)
                              n855 = Select(t=T1."Enable Test" ("f"), s=w2329, f=w2334) -> (s? t:f=w2341:T1)
                              n856 = Select(t=T1."Speed Command" ("f"), s=w2328, f=w2334) -> (s? t:f=w2340:T1)
                              n857 = Select(t=T1."Temp Control" ("f"), s=w2332, f=w2334) -> (s? t:f=w2339:T1)
                              n858 = Select(t=T1."Burn in" ("f"), s=w2333, f=w2334) -> (s? t:f=w2338:T1)
                              n859 = Select(t=T1."Visual Inspec" ("f"), s=w2345, f=w2334) -> (s? t:f=w2337:T1)
                              n860 = Select(t=T1."Auxiliary" ("f"), s=w2336, f=w2334) -> (s? t:f=w2326:T1)
                              n861 = Build Array(w2344, w2326, w2343, w2342, w2341, w2340, w2339, w2338, w2337) -> (w2354:T11)
                            }
                            frame True {
                              w2355 = T11 [enum."Com Test", enum."Auxiliary", enum."Temp Sens Cal", enum."Stop Time", enum."Enable Test", enum."Speed Command", enum."Temp Control", enum."Burn in", enum."Visual Inspec"] items=["Auxiliary", "Temp Sens Cal", "Com Test", "Enable Test", "Speed Command", "Stop Time", "Temp Control", "Burn in", "Visual Inspec", "Empty"]
                            }
                          }
                        }
                      }
                    }
                  }
                  "Automation" <- w2240
                  n862 = control-ref of="ATR"() -> (w2241:refnum<vi>)
                  n863 = flat-sequence {
                    tunnel: [enum16{"Stop", "Tests", "Bit test", "Start"}."Tests"] -> w2245
                    tunnel: [TRUE] -> w2244
                    frame #0 {
                    }
                  }
                  n864 = case shown="True" w2240 {
                    tunnel: w2241 -> [_ w2249]
                    frame False {
                    }
                    frame True {
                      n865 = call "ResetTable Result (SubVI).vi"("Table in"=w2249) -> ()  [unwired: 11 in]
                    }
                  }
                  n866 = property on="Stop Button" class="Bool (strict)"("Value"=FALSE ("Stop Burn-in")) -> ()  [unwired: 2 in, 2 out]
                  n867 = property on="Start" class="Bool (strict)"("DisabledEnum"=w2243) -> ()  [unwired: 2 in, 2 out]
                  n868 = property on="Report" class="Bool (strict)"("DisabledEnum"=w2243) -> ()  [unwired: 2 in, 2 out]
                }
                frame "Bit test" {
                  # "Stop"
                  n869 = call "SerialMarvinSendGet.vi"("write buffer"="TA[1]\r\n", "VISA resource name"=w2391) -> ("error out"=w2366:errorcluster, "read buffer"=w2401:string)  [unwired: 8 in]
                  n870 = Fract/Exp String To Number(string=w2401) -> (number=w2365:dbl)  [unwired: 3 in, 1 out]
                  n871 = call "TAs StartTest (SubVI).vi"("error in"=w2366, "Numeric"=w2365, "Enum"=enum16{"TA3", "TA2", "TA1"}."TA1") -> ("error out"=w2364:errorcluster, "String Out"=w2363:string, "Result"=w2362:bool)  [unwired: 6 in]
                  n872 = call "TesterOption (SubVI).vi"("On/Off 2"=FALSE, "Tester Option 2"=T6."Venable", "2 Options"=TRUE, "error in (no error)"=w2364, "On/Off"=TRUE, "Tester Option"=T6."25C") -> ("error out"=w2393:errorcluster)  [unwired: 4 in, 1 out]
                  n873 = call "Time Delay5"("error in (no error)"=w2393) -> ("error out"=w2392:errorcluster)  [unwired: 10 in]
                  n874 = call "SerialMarvinSendGet.vi"("error in (no error)"=w2392, "write buffer"="TA[2]\r\n", "VISA resource name"=w2391) -> ("error out"=w2360:errorcluster, "read buffer"=w2395:string)  [unwired: 7 in]
                  n875 = Fract/Exp String To Number(string=w2395) -> (number=w2359:dbl)  [unwired: 3 in, 1 out]
                  n876 = call "TAs StartTest (SubVI).vi"("error in"=w2360, "Numeric"=w2359, "Enum"=enum16{"TA3", "TA2", "TA1"}."TA2") -> ("error out"=w2358:errorcluster, "String Out"=w2357:string, "Result"=w2356:bool)  [unwired: 6 in]
                  n877 = call "GetADCTester (SubVI).vi"("error in (no error)"=w2358, "GetADCTester"=T8."Term1", "TimeToGet"=5) -> ("error out"=w2374:errorcluster, "ADCValOutput Single"=w2372:dbl)  [unwired: 6 in, 1 out]
                  n878 = case shown="\"EBAY\"" w2380 {
                    tunnel: w2391 -> [_ _ w2467]
                    tunnel: w2374 -> [w2434 w2451 w2466]
                    tunnel: [w2428 w2451 w2464] -> w2382
                    tunnel: [w2425 "" w2461] -> w2388
                    tunnel: [w2424 bool[] [] w2460] -> w2373
                    frame "AHU" {
                      n879 = call "TesterOption (SubVI).vi"("On/Off 2"=FALSE, "Tester Option 2"=T6."Venable", "2 Options"=TRUE, "error in (no error)"=w2434, "On/Off"=TRUE, "Tester Option"=T6."K17") -> ("error out"=w2436:errorcluster)  [unwired: 4 in, 1 out]
                      n880 = call "Time Delay7"("error in (no error)"=w2436) -> ("error out"=w2435:errorcluster)  [unwired: 10 in]
                      n881 = call "GetADCTester (SubVI).vi"("error in (no error)"=w2435, "GetADCTester"=T8."Current", "TimeToGet"=5) -> ("error out"=w2428:errorcluster, "ADCValOutput Single"=w2430:dbl)  [unwired: 6 in, 1 out]
                      n882 = Less Or Equal?(x=w2430, y=10.0) -> (x <= y?=w2429:bool)
                      n883 = Build Array(w2429) -> (w2424:bool[])
                      n884 = for {
                        tunnel: w2424 -> [w2448] mode=indexing
                        tunnel: string[] ["Current sensor not connected!"] -> [w2445] mode=indexing
                        shift-right: [w2446] -> w2425
                        shift-left: "" -> [w2443]
                        n885 = Concatenate Strings(w2445, "\r\n") -> (w2442:string)
                        n886 = Select(t=w2443, s=w2448, f=w2442) -> (s? t:f=w2447:string)
                        n887 = Concatenate Strings(w2443, w2447) -> (w2446:string)
                      }
                    }
                    frame Default {
                    }
                    frame "EBAY" {
                      w2465 = T30 [enum."Fan", enum."Current"] items=["Term1", "Term2", "Current", "Fan", "TempCPU"]
                      n888 = call "TesterOption (SubVI).vi"("On/Off 2"=FALSE, "Tester Option 2"=T6."Venable", "2 Options"=TRUE, "error in (no error)"=w2466, "On/Off"=TRUE, "Tester Option"=T6."K17") -> ("error out"=w2469:errorcluster)  [unwired: 4 in, 1 out]
                      n889 = call "Time Delay6"("error in (no error)"=w2469) -> ("error out"=w2468:errorcluster)  [unwired: 10 in]
                      n890 = call "SerialMarvinSendGet.vi"("error in (no error)"=w2468, "write buffer"="TA[3]\r\n", "VISA resource name"=w2467) -> ("error out"=w2455:errorcluster, "read buffer"=w2471:string)  [unwired: 7 in]
                      n891 = Fract/Exp String To Number(string=w2471) -> (number=w2456:dbl)  [unwired: 3 in, 1 out]
                      n892 = call "TAs StartTest (SubVI).vi"("error in"=w2455, "Numeric"=w2456, "Enum"=enum16{"TA3", "TA2", "TA1"}."TA3") -> ("error out"=w2452:errorcluster, "String Out"=w2454:string, "Result"=w2453:bool)  [unwired: 6 in]
                      n893 = for {
                        tunnel: w2465 -> [w2493] mode=indexing
                        tunnel: w2452 -> [w2491]
                        tunnel: [w2490] -> w2464
                        tunnel: [w2487] -> w2463 mode=indexing
                        i -> [w2488]
                        n894 = call "GetADCTester (SubVI).vi"("error in (no error)"=w2491, "GetADCTester"=w2493, "TimeToGet"=5) -> ("error out"=w2490:errorcluster, "ADCValOutput Single"=w2489:dbl)  [unwired: 6 in, 1 out]
                        n895 = case shown="1" w2488 {
                          tunnel: w2489 -> [w2496 w2499 _]
                          tunnel: [w2494 w2497 FALSE] -> w2487
                          frame 1 {
                            n896 = Less Or Equal?(x=w2496, y=10.0) -> (x <= y?=w2494:bool)
                          }
                          frame 0 {
                            n897 = Greater Or Equal?(x=w2499, y=2200.0) -> (x >= y?=w2497:bool)
                          }
                          frame Default {
                          }
                        }
                      }
                      n898 = Build Array (concatenate)(w2453, w2463) -> (w2460:bool[])
                      n899 = Build Array (concatenate)(w2454, string[] ["AUX Fan not connected!", "Current sensor not connected!"]) -> (w2458:string[])
                      n900 = for {
                        tunnel: w2460 -> [w2477] mode=indexing
                        tunnel: w2458 -> [w2480] mode=indexing
                        shift-right: [w2482] -> w2461
                        shift-left: "" -> [w2481]
                        n901 = Concatenate Strings(w2480, "\r\n") -> (w2478:string)
                        n902 = case shown="False" w2477 {
                          tunnel: [w2485 w2486] -> w2482
                          tunnel: w2481 -> [w2484 w2486]
                          tunnel: w2478 -> [w2483 _]
                          frame False {
                            n903 = Concatenate Strings(w2484, w2483) -> (w2485:string)
                          }
                          frame True {
                          }
                        }
                      }
                    }
                  }
                  n904 = Less Or Equal?(x=w2372, y=100.0) -> (x <= y?=w2370:bool)
                  n905 = Build Array(w2363, w2357, "Failure - check 28V or GND signals. Pin28 or Pin2") -> (w2369:string[])
                  n906 = Build Array(w2362, w2356, w2370) -> (w2387:bool[])
                  n907 = for {
                    tunnel: w2387 -> [w2413] mode=indexing
                    tunnel: w2369 -> [w2417] mode=indexing
                    shift-right: [w2419] -> w2389
                    shift-left: "" -> [w2418]
                    tunnel: w2382 -> [w2414]
                    tunnel: [w2414] -> w2381
                    n908 = Concatenate Strings(w2417, "\r\n") -> (w2415:string)
                    n909 = case shown="False" w2413 {
                      tunnel: [w2422 w2423] -> w2419
                      tunnel: w2418 -> [w2421 w2423]
                      tunnel: w2415 -> [w2420 _]
                      frame False {
                        n910 = Concatenate Strings(w2421, w2420) -> (w2422:string)
                      }
                      frame True {
                      }
                    }
                  }
                  n911 = Build Array (concatenate)(w2387, w2373) -> (w2386:bool[])
                  n912 = And Array Elements(Boolean array=w2386) -> (logical AND=w2377:bool)
                  n913 = case shown="False" w2377 {
                    tunnel: w2389 -> [w2411 _]
                    tunnel: w2388 -> [w2410 _]
                    tunnel: w2381 -> [w2408 w2412]
                    tunnel: [w2408 w2412] -> w2379
                    frame False {
                      n914 = Concatenate Strings(w2411, w2410) -> (w2409:string)
                      n915 = One Button Dialog(message=w2409) -> ()  [unwired: 1 in, 1 out]
                    }
                    frame True {
                    }
                  }
                  n916 = case shown="False" w2377 {
                    tunnel: w2379 -> [w2406 w2407]
                    tunnel: [w2405 w2407] -> w2378
                    frame False {
                      n917 = call "Display Message to User6"("error in (no error)"=w2406) -> ("error out"=w2405:errorcluster)  [unwired: 9 in, 1 out]
                    }
                    frame True {
                    }
                  }
                  n918 = Select(t=enum16{"Stop", "Tests", "Bit test", "Start"}."Tests", s=w2377, f=enum16{"Stop", "Tests", "Bit test", "Start"}."Stop") -> (s? t:f=w2383:enum16{"Stop", "Tests", "Bit test", "Start"})
                }
                frame "Start" {
                  n919 = And(x=w2502, y=w2507) -> (x .and. y?=w2503:bool)
                  n920 = case shown="True" w2503 {
                    tunnel: w2512 -> [_ w2535]
                    tunnel: w2511 -> [_ w2528]
                    tunnel: w2510 -> [_ w2524]
                    tunnel: [FALSE w2522] -> w2506
                    tunnel: [w2518 w2521] -> w2501
                    tunnel: [FALSE TRUE] -> w2504
                    frame False {
                      n921 = call "Display Message to User5"() -> ("error out"=w2518:errorcluster)  [unwired: 10 in, 1 out]
                    }
                    frame True {
                      n922 = call "TesterOption (SubVI).vi"("2 Options"=FALSE, "On/Off"=FALSE, "Tester Option"=T6."Venable") -> ("error out"=w2530:errorcluster)  [unwired: 7 in, 1 out]
                      n923 = call "Write panel message Kinetics (SubVI).vi"("rpm"=FALSE, "PrintTime"=FALSE, "Stop"=w2524, "error in (no error)"=w2530, "Time to wait"=3.0, "Strin"="TESTER BIT TEST OPERATION IN PROCESS\nPlease wait...", "String in"=w2528) -> ("error out"=w2529:errorcluster)  [unwired: 4 in]
                      n924 = property on="UUT SoftwareVer" class="Str"() -> ("Value"=w2520:string)  [unwired: 2 in, 2 out]
                      n925 = call "SerialMarvinSendGet.vi"("error in (no error)"=w2529, "write buffer"="VR\r\n", "VISA resource name"=w2535) -> ("error out"=w2521:errorcluster, "read buffer"=w2534:string)  [unwired: 7 in]
                      n926 = Equal?(x=w2534, y=w2520) -> (x = y?=w2522:bool)
                    }
                  }
                  n927 = case shown="True" w2506 {
                    tunnel: [enum16{"Stop", "Tests", "Bit test", "Start"}."Stop" enum16{"Stop", "Tests", "Bit test", "Start"}."Bit test"] -> w2505
                    tunnel: w2504 -> [w2513 _]
                    frame False {
                      n928 = case shown="True" w2513 {
                        frame False {
                        }
                        frame True {
                          n929 = call "Display Message to User4"() -> ()  [unwired: 10 in, 2 out]
                        }
                      }
                    }
                    frame True {
                    }
                  }
                }
              }
            }
            n930 = Bundle By Name(cluster=T2 {"VISA"="COM1", "Array Test"=[]}, "VISA"=w2206, "Array Test"=w2212) -> (w2208:T2)
            n931 = Enqueue Element(queue=w2214, element=w2208, error in (no error)=w2211) -> (queue out=w2209:refnum<queue>, error out=w2210:errorcluster)  [unwired: 2 out]
          }
          event "Report", "Stop Button": Value Change {
            w2564 = T31 1 items=["User Home"=0, "User Desktop"=1, "User Documents"=2, "User Application Data"=3, "User Preferences"=4, "User Temporary"=5, "Public Documents"=6, "Public Application Data"=7, "Public Preferences"=8, "Public Cache"=13, "System Core Libraries"=9, "System Installed Libraries"=10, "Application Files"=11, "Boot Volume Root"=12] ("system directory type")
            w2595 = "Marvin" ("section")
            n932 = event-data() -> ("CtlRef"=w2587:refnum<vi>)  [unwired: 1 in]
            n933 = local read "UUT"() -> (w2561:string)
            n934 = call <vilib>:"Get System Directory.vi"("system directory type"=w2564) -> ("system directory"=w2563:path)  [unwired: 10 in]
            n935 = Build Path(base path=w2563, name or relative path="MarvinReports") -> (appended path=w2624:path)
            n936 = property on="CAN Status" class="Bool (strict)"() -> ("Value"=w2567:bool)  [unwired: 2 in, 2 out]
            n937 = property on="Status" class="Bool (strict)"() -> ("Value"=w2568:bool)  [unwired: 2 in, 2 out]
            n938 = case shown="\"AHU\"" w2561 {
              tunnel: ["REV EBAY" ("key") "REV AHU" ("key")] -> w2593
              frame "EBAY", Default {
              }
              frame "AHU" {
              }
            }
            n939 = call <vilib>:"Check if File or Folder Exists.vi"("path"=w2624) -> ("error out"=w2622:errorcluster, "file or folder exists?"=w2625:bool, "dup path"=w2623:path)  [unwired: 8 in]
            n940 = And(x=w2568, y=w2567) -> (x .and. y?=w2569:bool)
            n941 = case shown="False" w2625 {
              tunnel: w2622 -> [w2689 w2690]
              tunnel: w2623 -> [w2688 w2691]
              tunnel: [w2687 w2691] -> w2566
              tunnel: [w2686 w2690] -> w2627
              frame False {
                n942 = Create Folder(path (use dialog)=w2688, error in=w2689) -> (created path=w2687:path, error out=w2686:errorcluster)  [unwired: 1 in, 1 out]
              }
              frame True {
              }
            }
            n943 = case shown="True" w2569 {
              tunnel: [w2634 w2654] -> w2611
              tunnel: [w2634 w2653] -> w2554
              tunnel: w2588 -> [_ w2642]
              tunnel: [w2634 w2647] -> w2559
              tunnel: [w2634 w2646] -> w2556
              tunnel: [w2634 w2650] -> w2581
              tunnel: [w2634 w2649] -> w2558
              tunnel: [w2634 w2638] -> w2555
              frame False {
                (unwired) "47"
                (unwired) " 413-8005_47_AHU"
                (unwired) "413-8005-1-47"
                (unwired) "5.3.9" ("read buffer")
                (unwired) "95"
                (unwired) "414-8005_95_EBAY_"
                (unwired) "414-8005-95"
                (unwired) "414-8005-95   "
                w2634 = "N_A" ("read buffer")
                n944 = disable-structure shown="Disabled" {
                  frame Disabled {
                    n945 = call "Display Message to User7"() -> ()  [unwired: 10 in, 2 out]
                  }
                  frame Enabled {
                  }
                }
                n946 = Decimal String To Number(string="1" ("Value")) -> (number=w2635:i32)  [unwired: 2 in, 1 out]
                n947 = Number To Decimal String(number=w2635, width (-)=i16 4) -> ()  [unwired: 1 out]
              }
              frame True {
                n948 = call "SerialMarvinSendGet.vi"("write buffer"="SN\r\n", "VISA resource name"=w2642) -> ("error out"=w2641:errorcluster, "read buffer"=w2644:string)  [unwired: 8 in]
                n949 = call "Time Delay2"("error in (no error)"=w2641) -> ("error out"=w2640:errorcluster)  [unwired: 10 in]
                n950 = Decimal String To Number(string=w2644) -> (number=w2643:i32)  [unwired: 2 in, 1 out]
                n951 = Number To Decimal String(number=w2643, width (-)=i16 4) -> (decimal integer string=w2647:string)
                n952 = call "SerialMarvinSendGet.vi"("error in (no error)"=w2640, "write buffer"="VR\r\n", "VISA resource name"=w2642) -> ("error out"=w2651:errorcluster, "read buffer"=w2646:string)  [unwired: 7 in]
                n953 = property on="UUT" class="DigNum (strict)"(error in=w2651) -> ("Value"=w2639:u8)  [unwired: 1 in, 2 out]
                n954 = call "SentenceFromFile (SubVI).vi"("UUT"=w2639) -> ("Sentence"=w2638:string)  [unwired: 9 in, 1 out]
                n955 = case shown="95, Default" w2639 {
                  tunnel: ["414-8005_95_EBAY_" " 413-8005_47_AHU" " 413-8005_63_AHU"] -> w2654
                  tunnel: ["414-8005-95   " w2660 w2663] -> w2653
                  tunnel: ["414-8005-95" w2660 w2663] -> w2650
                  tunnel: ["95" "47" "63"] -> w2649
                  frame 95, Default {
                  }
                  frame 47 {
                    w2660 = "413-8005-1-47"
                    (unwired) "AHU-L (47) 413-8005-1"
                  }
                  frame 63 {
                    w2663 = "413-8005-2-63"
                    (unwired) "AHU-R (63) 413-8005-2"
                  }
                }
              }
            }
            n956 = Get Date/Time String(want seconds? (F)=TRUE) -> (date string=w2626:string)  [unwired: 2 in, 1 out]
            n957 = call <vilib>:"Open Config Data.vi"("create file if necessary (T)"=FALSE, "configuration file path"=w2590) -> ("refnum"=w2602:T5)  [unwired: 1 in, 8 out]
            n958 = property on="Logger Path" class="Path"(error in=w2627, "Value"=w2566, "StartPath"=w2566) -> (error out=w2605:errorcluster)  [unwired: 1 in, 1 out]
            n959 = Search and Replace String(replace all?=TRUE ("replace all? (F)"), input string=w2626, search string="/") -> (result string=w2608:string)  [unwired: 5 in, 3 out]
            n960 = call-poly <vilib>:"Read Key.vi"("section"=w2595, "key"=w2593, "refnum"=w2602) -> ("error out"=w2597:errorcluster, "value"=w2600:string, "refnum out"=w2599:T5)  [unwired: 5 in, 1 out]
            n961 = call-poly <vilib>:"Read Key.vi"("section"=w2595, "error in (no error)"=w2597, "key"="Tester Software Ver", "refnum"=w2599) -> ("error out"=w2594:errorcluster, "value"=w2557:string, "refnum out"=w2598:T5)  [unwired: 4 in, 1 out]
            n962 = Concatenate Strings("ATR" ("string"), w2611, w2559, "_", w2608, ".docx" ("string")) -> (w2606:string)
            n963 = call <vilib>:"Close Config Data.vi"("error in (no error)"=w2594, "refnum"=w2598) -> ()  [unwired: 8 in, 2 out]
            n964 = Build Path(base path=w2566, name or relative path=w2606) -> (appended path=w2607:path)
            n965 = Concatenate Strings("  Rev-" ("string"), w2600) -> (w2589:string)
            n966 = while {
              tunnel: w2606 -> [w2671]
              tunnel: w2566 -> [w2668]
              shift-right: [w2670] -> w2604
              shift-left: w2607 -> [w2669]
              shift-right: [w2666] -> w2591
              shift-left: w2592 -> [w2667]
              tunnel: w2605 -> [w2672]
              tunnel: [w2673] -> w2565
              stop <- w2665 continue-if-true
              n967 = call <vilib>:"Check if File or Folder Exists.vi"("error in (no error)"=w2672, "path"=w2669) -> ("error out"=w2673:errorcluster, "file or folder exists?"=w2665:bool)  [unwired: 7 in, 1 out]
              n968 = case shown="True" w2665 {
                tunnel: w2671 -> [_ w2685]
                tunnel: w2667 -> [_ w2677]
                tunnel: [w2675 w2682] -> w2670
                tunnel: w2669 -> [w2675 _]
                tunnel: w2668 -> [_ w2683]
                tunnel: [1 w2676] -> w2666
                frame False {
                }
                frame True {
                  w2678 = ".docx" ("search string")
                  n969 = Search and Replace String(input string=w2685, search string=w2678) -> (result string=w2684:string)  [unwired: 6 in, 3 out]
                  n970 = Number To Decimal String(number=w2677) -> (decimal integer string=w2680:string)  [unwired: 1 in]
                  n971 = call <vilib>:"Space Constant.vi"() -> ("String"=w2679:string)
                  n972 = Concatenate Strings(w2684, w2679, w2680, w2678) -> (w2681:string)
                  n973 = Build Path(base path=w2683, name or relative path=w2681) -> (appended path=w2682:path)
                  n974 = Increment(x=w2677) -> (x+1=w2676:i32)
                }
              }
            }
            n975 = call "HeaderBis.vi"("UUTHeader"=w2561, "UA"=w2558, "Revision Param"=w2555, "P/N UUT"=w2554, "Driver S/N"=w2559, "VR"=w2556, "Oper."=w2560, "Tester Software Ver"=w2557) -> ("table header"=w2553:string, "Array"=w2552:string[][])  [unwired: 5 in, 1 out]
            n976 = Open/Create/Replace File(file path (use dialog)=w2604, error in=w2565, operation (0:open)=T18."create") -> (error out=w2617:errorcluster)  [unwired: 3 in, 2 out]
            n977 = control-ref of="ATR"() -> (w2629:refnum<vi>)
            n978 = property class="Tbl (strict)"(reference=w2629, error in=w2617) -> ("Value"=w2630:string[][])  [unwired: 2 out]
            n979 = control-ref of="ATR"() -> (w2545:refnum<vi>)
            n980 = call "PassFailUUT (SubVI).vi"("Table in"=w2545) -> ("PassFaileUUTresult"=w2538:bool)  [unwired: 8 in, 2 out]
            n981 = property on="Test Failed" class="Bool (strict)"("Value"=w2538) -> ()  [unwired: 2 in, 2 out]
            n982 = call "MarvinReport.vi"("HEADER1"=w2553, "ATR Or"=w2629, "Steps   pfull"=w2630, "Footer UUT"=w2581, "pageNum"=3, "InputHeaderArray"=w2552, "FILE NAME"=w2606, "Report Folder"=w2604, "REV"=w2589, "Test-Conductor"=w2560) -> ("error out"=w2576:errorcluster)  [unwired: 4 in, 1 out]
            n983 = Select(t="PASS" ("name or relative path"), s=w2538, f="FAIL" ("name or relative path")) -> (s? t:f=w2537:string)
            n984 = call <vilib>:"Clear Errors.vi"("error in (no error)"=w2576) -> ("error out"=w2575:errorcluster)  [unwired: 5 in, 1 out]
            n985 = property class="Bool (strict)"(reference=w2587, error in=w2575) -> ("BoolText.Text"=w2586:string)  [unwired: 2 out]
            n986 = Equal?(x=w2586, y="Report") -> (x = y?=w2580:bool)
            n987 = Select(t=T4."MainProgram", s=w2580, f=T4."Stop") -> (s? t:f=w2583:T4)
            n988 = call <vilib>:"Application Directory.vi"() -> ("Application Directory"=w2541:path)
            n989 = Build Path(base path=w2541, name or relative path="data\\TestResult.ini") -> (appended path=w2544:path)
            n990 = Select(t="Save Report...", s=w2580, f="Program Stopped...\r\nPlease turn OFF All Power sinks") -> (s? t:f=w2578:string)
            n991 = property on="Report" class="Bool (strict)"(error in=w2575, "Value"=FALSE ("Report")) -> (error out=w2570:errorcluster)  [unwired: 1 in, 1 out]
            n992 = call <vilib>:"Open Config Data.vi"("configuration file path"=w2544) -> ("error out"=w2542:errorcluster, "refnum"=w2543:T5)  [unwired: 2 in, 7 out]
            n993 = property on="Pannel User Message" class="Str"("Value"=w2578) -> ()  [unwired: 2 in, 2 out]
            n994 = call-poly <vilib>:"Write Key.vi"("section"="Kinetics", "error in (no error)"=w2542, "value"=w2537, "key"="Result", "refnum"=w2543) -> ("error out"=w2540:errorcluster, "refnum out"=w2539:T5)  [unwired: 4 in, 1 out]
            n995 = call <vilib>:"Close Config Data.vi"("error in (no error)"=w2540, "refnum"=w2539) -> ()  [unwired: 8 in, 2 out]
            n996 = call "TesterOption (SubVI).vi"("2 Options"=FALSE, "error in (no error)"=w2570, "On/Off"=FALSE, "Tester Option"=T6."Venable") -> ()  [unwired: 6 in, 2 out]
          }
          event "Help Button": Value Change {
            n997 = event-data() -> ()  [unwired: 1 in, 6 out]
            n998 = vi-ref "Help.vi"() -> (w2705:refnum<vi>)
            n999 = invoke class="VI" method="FP.Open"(reference=w2705, error in=w2703, "Activate"=TRUE ("Activate?"), "State"=T16."Standard") -> (error out=w2704:errorcluster)  [unwired: 1 in, 4 out]
            n1000 = call "Help.vi"("error in"=w2704, "TesterSWVersion"=w2695) -> ("error out"=w2702:errorcluster)  [unwired: 6 in]
            n1001 = property on="Help Button" class="Bool (strict)"("Value"=FALSE ("Help Button")) -> ()  [unwired: 2 in, 2 out]
          }
          event "Serial Com": Value Change {
            n1002 = event-data() -> ()  [unwired: 1 in, 6 out]
            n1003 = property on="Serial Com" class="Bool"(error in=w2716, "Visible"=FALSE) -> (error out=w2720:errorcluster)  [unwired: 1 in, 1 out]
            n1004 = property on="VISA Kinetics" class="VISAName"(error in=w2720, "Visible"=TRUE) -> (error out=w2717:errorcluster)  [unwired: 1 in, 1 out]
          }
          event "VISA Kinetics": Value Change {
            n1005 = event-data() -> ()  [unwired: 1 in, 6 out]
            n1006 = property on="Serial Com" class="Bool"(error in=w2724, "Visible"=FALSE) -> ()  [unwired: 1 in, 2 out]
            n1007 = property on="Pannel User Message" class="Str"(error in=w2724, "Value"="Serial connection in process" ("Pannel User Message")) -> ()  [unwired: 1 in, 2 out]
          }
          event "Refresh Button": Value Change {
            n1008 = event-data() -> ()  [unwired: 1 in, 6 out]
          }
          event "Settings": Value Change {
            n1009 = event-data() -> ()  [unwired: 1 in, 6 out]
          }
        }
      }
      frame "Initialize" {
        w2758 = 0
        w2761 = FALSE ("Visible")
        w2762 = FALSE ("Visible")
        w2763 = FALSE ("Visible")
        w2764 = FALSE ("Visible")
        w2771 = refnum<visa-resource-name> "COMx" ("VISA resource name")
        w2760 = FALSE ("Serial Status")
        n1010 = property on="ComTestResult" class="Bool (strict)"("Value"=w2764) -> ()  [unwired: 2 in, 2 out]
        n1011 = property on="VenableResult" class="Bool (strict)"("Value"=w2764) -> ()  [unwired: 2 in, 2 out]
        n1012 = property on="VenableDirectionResult" class="Bool (strict)"("Value"=w2764) -> ()  [unwired: 2 in, 2 out]
        n1013 = property on="Serial Com" class="Bool"(error in=errorcluster {"status"=FALSE, "code"=0, "source"=""} ("error out"), "Visible"=TRUE) -> (error out=w2773:errorcluster)  [unwired: 1 in, 1 out]
        n1014 = property on="AuxiOFFResult" class="Bool (strict)"("Value"=w2763) -> ()  [unwired: 2 in, 2 out]
        n1015 = property on="AuxiONResult" class="Bool (strict)"("Value"=w2763) -> ()  [unwired: 2 in, 2 out]
        n1016 = property on="VisualInspectionResult" class="Bool (strict)"("Value"=w2763) -> ()  [unwired: 2 in, 2 out]
        n1017 = property on="SensCalResult" class="Bool (strict)"("Value"=w2763) -> ()  [unwired: 2 in, 2 out]
        n1018 = property on="VISA Kinetics" class="VISAName"(error in=w2773, "Visible"=FALSE, "Value"=w2771) -> (error out=w2749:errorcluster)  [unwired: 1 in, 1 out]
        n1019 = property on="BurnDC" class="Bool (strict)"("Value"=w2762) -> ()  [unwired: 2 in, 2 out]
        n1020 = property on="BurnTemp" class="Bool (strict)"("Value"=w2762) -> ()  [unwired: 2 in, 2 out]
        n1021 = property on="BurnSpeed" class="Bool (strict)"("Value"=w2762) -> ()  [unwired: 2 in, 2 out]
        n1022 = property on="BurnResult" class="Bool (strict)"("Value"=w2762) -> ()  [unwired: 2 in, 2 out]
        n1023 = property on="Refresh Button" class="Bool (strict)"(error in=w2749, "Value"=FALSE ("Refresh Button")) -> (error out=w2750:errorcluster)  [unwired: 1 in, 1 out]
        n1024 = property on="MotorTempResult" class="Bool (strict)"("Value"=w2761) -> ()  [unwired: 2 in, 2 out]
        n1025 = property on="TempControlResult" class="Bool (strict)"("Value"=w2761) -> ()  [unwired: 2 in, 2 out]
        n1026 = property on="Automation" class="Bool (strict)"("Value"=w2761) -> ()  [unwired: 2 in, 2 out]
        n1027 = call "Find DAQ Devices.vi"("Error In"=w2750) -> ("Error Out"=w2754:errorcluster, "DAQmx Device Name"=w2755:tag)  [unwired: 9 in]
        "DAQmx Device Name" <- w2755
        n1028 = call <vilib>:"Clear Errors.vi"("error in (no error)"=w2754) -> ("error out"=w2753:errorcluster)  [unwired: 5 in, 1 out]
        n1029 = Not Equal?(x=w2755, y=tag "") -> (x != y?=w2756:bool)
        n1030 = case shown="True" w2756 {
          tunnel: w2755 -> [_ w2779]
          tunnel: w2753 -> [w2775 w2778]
          tunnel: [w2775 w2777] -> w2751
          frame False {
          }
          frame True {
            w2776 = u16 0 items=["Init", "0 ohm", "6 ohm", "13.2 ohm", "15 ohm", "25.9 ohm", "33 ohm", "Down", "Up", "Venable", "Firmware", "PowerSuply"] ("Operation")
            n1031 = call "Operation (SubVI).vi"("error in (no error)"=w2778, "Operation"=w2776, "DAQmx Device Name"=w2779) -> ("error out"=w2777:errorcluster)  [unwired: 8 in]
          }
        }
        "Status" <- w2760
        "Test Failed" <- w2760
      }
    }
  }
  n1032 = property on="Settings" class="Bool (strict)"("Visible"=w20) -> ()  [unwired: 2 in, 2 out]
  n1033 = call "ATRBuild.vi"() -> ()  [unwired: 10 in, 2 out]
  n1034 = disable-structure shown="Disabled" {
    frame Disabled {
      n1035 = control-ref of="Stop Button"() -> ()  [unwired: 1 out]
      n1036 = control-ref of="UUT"() -> ()  [unwired: 1 out]
      n1037 = control-ref of="UUT"() -> ()  [unwired: 1 out]
      n1038 = property on="UUT" class="DigNum (strict)" props=["Value"]() -> ()  [unwired: 2 in, 3 out]
      n1039 = control-ref of="Motor Speed RPM Serial"() -> ()  [unwired: 1 out]
      n1040 = call "Find_Number_LineMARVIN.vi"() -> ()  [unwired: 5 in, 4 out]
      n1041 = call "Write panel message Kinetics (SubVI).vi"() -> ()  [unwired: 11 in, 1 out]
      n1042 = control-ref of="ATR"() -> ()  [unwired: 1 out]
      n1043 = call "PassOrFail (SubVI).vi"() -> ()  [unwired: 11 in, 1 out]
    }
    frame Enabled {
    }
  }
  n1044 = disable-structure shown="Disabled" {
    frame Disabled {
      w2780 = T14."Disabled and Grayed Out" ("Disabled")
      w2781 = FALSE ("Start")
      n1045 = property on="Current SN" class="DigNum (strict)" props=["Value"]() -> ()  [unwired: 2 in, 3 out]
      n1046 = property on="UUT" class="DigNum (strict)" props=["Value"]() -> ()  [unwired: 2 in, 3 out]
      n1047 = property on="Status" class="Bool (strict)" props=["Value"]() -> ()  [unwired: 2 in, 3 out]
      n1048 = property on="UUT SoftwareVer" class="Str" props=["Value"]() -> ()  [unwired: 2 in, 3 out]
      n1049 = call "Operation (SubVI).vi"() -> ()  [unwired: 11 in, 1 out]
      n1050 = property on="Next SN" class="DigNum (strict)" props=["Value"]() -> ()  [unwired: 3 in, 2 out]
      n1051 = property on="Start" class="Bool (strict)"("Value"=w2781, "DisabledEnum"=w2780) -> ()  [unwired: 2 in, 2 out]
      n1052 = property on="Report" class="Bool (strict)"("Value"=w2781, "DisabledEnum"=w2780) -> ()  [unwired: 2 in, 2 out]
    }
    frame Enabled {
    }
  }
  n1053 = disable-structure shown="Disabled" {
    frame Disabled {
      n1054 = flat-sequence {
        frame #0 {
          n1055 = call "CANSendMessage.vi"(7:TRUE ("Remote"), "Data"=u16 0 ("Motor Speed RPM")) -> ("error out"=w2782:errorcluster, "ID"=w2785:u32)  [unwired: 8 in]
          n1056 = call "TesterOption (SubVI).vi"("error in (no error)"=w2782, "On/Off"=FALSE, "Tester Option"=T6."Power") -> ()  [unwired: 7 in, 2 out]
        }
      }
    }
    frame Enabled {
    }
  }
  "Pannel User Message" <- w19
